vi "ui move files.vi"() -> ()   [LabVIEW 2023]
panel:
  out "Array 2":errorcluster[](array[cluster])
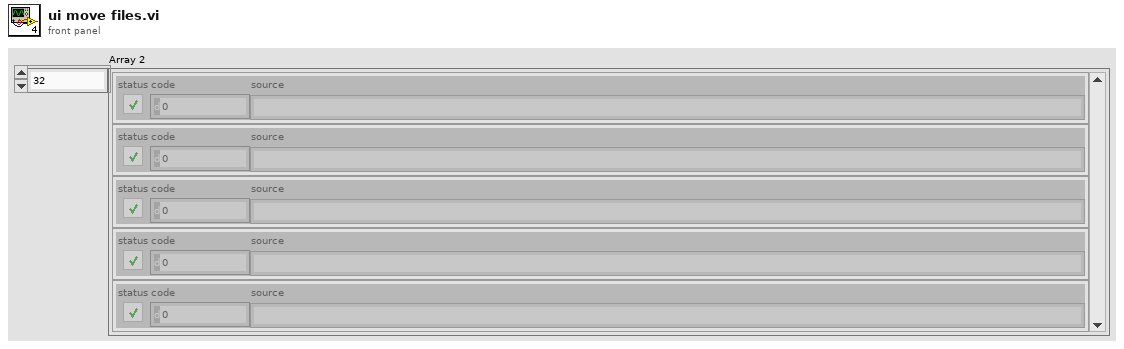
[diagram p1: front panel]
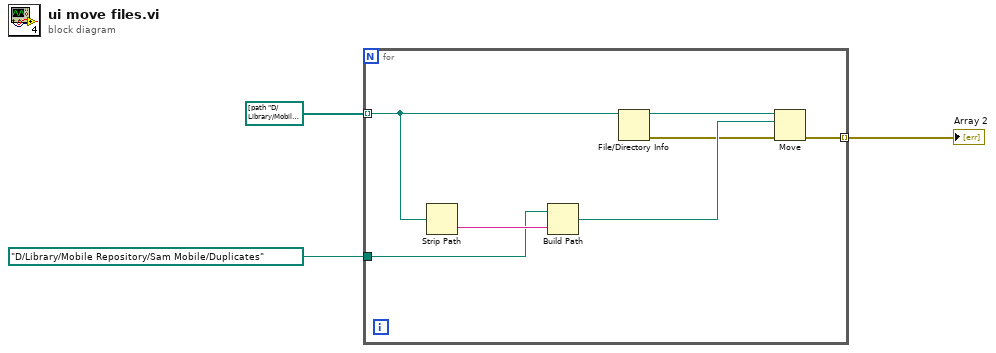
[diagram p0: block diagram]
diagram:
  n1 = for {
    tunnel: path[] [path "D:/Library/Mobile Repository/Sam Mobile/Albums/2017/08 August/iPhone 6s/20170810_162319 036_0000 iPhone 6s.JPG", path "D:/Library/Mobile Repository/Sam Mobile/Albums/2017/08 August/iPhone 6s/20170810_162319 121_0403 iPhone 6s.JPG", path "D:/Library/Mobile Repository/Sam Mobile/Albums/2017/08 August/iPhone 6s/20170814_132441 027_0000 iPhone 6s.JPG", path "D:/Library/Mobile Repository/Sam Mobile/Albums/2017/08 August/iPhone 6s/20170814_132441 121_0403 iPhone 6s.JPG", path "D:/Library/Mobile Repository/Sam Mobile/Albums/2017/08 August/iPhone 6s/20170814_134311 060_0000 iPhone 6s.JPG", path "D:/Library/Mobile Repository/Sam Mobile/Albums/2017/08 August/iPhone 6s/20170814_134311 121_0403 iPhone 6s.JPG", path "D:/Library/Mobile Repository/Sam Mobile/Albums/2017/08 August/iPhone 6s/20170816_123500 042_0000 iPhone 6s.JPG", path "D:/Library/Mobile Repository/Sam Mobile/Albums/2017/08 August/iPhone 6s/20170816_123500 121_0403 iPhone 6s.JPG", path "D:/Library/Mobile Repository/Sam Mobile/Albums/2017/08 August/iPhone 6s/20170822_182046 064_0000 iPhone 6s.JPG", path "D:/Library/Mobile Repository/Sam Mobile/Albums/2017/08 August/iPhone 6s/20170822_182046 121_0403 iPhone 6s.JPG", path "D:/Library/Mobile Repository/Sam Mobile/Albums/2017/08 August/iPhone 6s/20170823_115543 027_0000 iPhone 6s.JPG", path "D:/Library/Mobile Repository/Sam Mobile/Albums/2017/08 August/iPhone 6s/20170823_115543 121_0403 iPhone 6s.JPG", path "D:/Library/Mobile Repository/Sam Mobile/Albums/2017/08 August/iPhone 6s/20170823_115549 031_0000 iPhone 6s.JPG", path "D:/Library/Mobile Repository/Sam Mobile/Albums/2017/08 August/iPhone 6s/20170823_115549 121_0403 iPhone 6s.JPG", path "D:/Library/Mobile Repository/Sam Mobile/Albums/2017/08 August/iPhone 6s/20170825_201654 088_0000 iPhone 6s.JPG", path "D:/Library/Mobile Repository/Sam Mobile/Albums/2017/08 August/iPhone 6s/20170825_201654 121_0403 iPhone 6s.JPG", path "D:/Library/Mobile Repository/Sam Mobile/Albums/2017/08 August/iPhone 6s/20170825_204405 020_0000 iPhone 6s.JPG", path "D:/Library/Mobile Repository/Sam Mobile/Albums/2017/08 August/iPhone 6s/20170825_204405 121_0403 iPhone 6s.JPG", path "D:/Library/Mobile Repository/Sam Mobile/Albums/2017/09 September/iPhone 6s/20170907_130931 040_0000 iPhone 6s.JPG", path "D:/Library/Mobile Repository/Sam Mobile/Albums/2017/09 September/iPhone 6s/20170907_130931 121_0403 iPhone 6s.JPG", path "D:/Library/Mobile Repository/Sam Mobile/Albums/2017/09 September/iPhone 6s/20170907_223224 028_0000 iPhone 6s.JPG", path "D:/Library/Mobile Repository/Sam Mobile/Albums/2017/09 September/iPhone 6s/20170907_223224 121_0403 iPhone 6s.JPG", path "D:/Library/Mobile Repository/Sam Mobile/Albums/2017/09 September/iPhone 6s/20170923_163143 016_0000 iPhone 6s.JPG", path "D:/Library/Mobile Repository/Sam Mobile/Albums/2017/09 September/iPhone 6s/20170923_163143 121_0403 iPhone 6s.JPG", path "D:/Library/Mobile Repository/Sam Mobile/Albums/2017/10 October/iPhone 6s/20171013_075457 058_0000 iPhone 6s.JPG", path "D:/Library/Mobile Repository/Sam Mobile/Albums/2017/10 October/iPhone 6s/20171013_075457 121_0403 iPhone 6s.JPG", path "D:/Library/Mobile Repository/Sam Mobile/Albums/2017/10 October/iPhone 6s/20171030_155745 035_0000 iPhone 6s.JPG", path "D:/Library/Mobile Repository/Sam Mobile/Albums/2017/10 October/iPhone 6s/20171030_155745 121_0403 iPhone 6s.JPG", path "D:/Library/Mobile Repository/Sam Mobile/Albums/2017/12 December/iPhone 6s/20171204_111158 031_0000 iPhone 6s.JPG", path "D:/Library/Mobile Repository/Sam Mobile/Albums/2017/12 December/iPhone 6s/20171204_111158 121_0403 iPhone 6s.JPG", path "D:/Library/Mobile Repository/Sam Mobile/Albums/2017/12 December/iPhone 6s/20171209_180705 096_0000 iPhone 6s.JPG", path "D:/Library/Mobile Repository/Sam Mobile/Albums/2017/12 December/iPhone 6s/20171209_180705 121_0403 iPhone 6s.JPG", path "D:/Library/Mobile Repository/Sam Mobile/Albums/2017/12 December/iPhone 6s/20171221_164753 051_0000 iPhone 6s.JPG", path "D:/Library/Mobile Repository/Sam Mobile/Albums/2017/12 December/iPhone 6s/20171221_164753 121_0403 iPhone 6s.JPG", path "D:/Library/Mobile Repository/Sam Mobile/Albums/2018/02 February/iPhone 6s/20180203_103521 071_0000 iPhone 6s.JPG", path "D:/Library/Mobile Repository/Sam Mobile/Albums/2018/02 February/iPhone 6s/20180203_103521 121_0403 iPhone 6s.JPG", path "D:/Library/Mobile Repository/Sam Mobile/Albums/2018/02 February/iPhone 6s/20180212_064540 016_0000 iPhone 6s.JPG", path "D:/Library/Mobile Repository/Sam Mobile/Albums/2018/02 February/iPhone 6s/20180212_064540 121_0403 iPhone 6s.JPG", path "D:/Library/Mobile Repository/Sam Mobile/Albums/2018/02 February/iPhone 6s/20180224_102935 031_0000 iPhone 6s.JPG", path "D:/Library/Mobile Repository/Sam Mobile/Albums/2018/02 February/iPhone 6s/20180224_102935 121_0403 iPhone 6s.JPG", path "D:/Library/Mobile Repository/Sam Mobile/Albums/2018/02 February/iPhone 6s/20180224_152749 099_0000 iPhone 6s.JPG", path "D:/Library/Mobile Repository/Sam Mobile/Albums/2018/02 February/iPhone 6s/20180224_152749 121_0403 iPhone 6s.JPG", path "D:/Library/Mobile Repository/Sam Mobile/Albums/2018/03 March/iPhone 6s/20180315_064600 038_0000 iPhone 6s.JPG", path "D:/Library/Mobile Repository/Sam Mobile/Albums/2018/03 March/iPhone 6s/20180315_064600 121_0403 iPhone 6s.JPG", path "D:/Library/Mobile Repository/Sam Mobile/Albums/2018/03 March/iPhone 6s/20180318_193958 057_0000 iPhone 6s.JPG", path "D:/Library/Mobile Repository/Sam Mobile/Albums/2018/03 March/iPhone 6s/20180318_193958 121_0403 iPhone 6s.JPG", path "D:/Library/Mobile Repository/Sam Mobile/Albums/2018/04 April/iPhone 6s/20180426_163707 061_0000 iPhone 6s.JPG", path "D:/Library/Mobile Repository/Sam Mobile/Albums/2018/04 April/iPhone 6s/20180426_163707 121_0403 iPhone 6s.JPG", path "D:/Library/Mobile Repository/Sam Mobile/Albums/2018/05 May/iPhone 6s/20180513_133729 108_0000 iPhone 6s.JPG", path "D:/Library/Mobile Repository/Sam Mobile/Albums/2018/05 May/iPhone 6s/20180513_133729 121_0403 iPhone 6s.JPG", path "D:/Library/Mobile Repository/Sam Mobile/Albums/2018/05 May/iPhone 6s/20180518_112206 115_0000 iPhone 6s.JPG", path "D:/Library/Mobile Repository/Sam Mobile/Albums/2018/05 May/iPhone 6s/20180518_112206 121_0403 iPhone 6s.JPG", path "D:/Library/Mobile Repository/Sam Mobile/Albums/2018/05 May/iPhone 6s/20180521_132134 040_4745 iPhone 6s.JPG", path "D:/Library/Mobile Repository/Sam Mobile/Albums/2018/05 May/iPhone 6s/20180521_132134 121_0403 iPhone 6s.JPG", path "D:/Library/Mobile Repository/Sam Mobile/Albums/2018/06 June/iPhone 6s/20180629_113101 031_0000 iPhone 6s.JPG", path "D:/Library/Mobile Repository/Sam Mobile/Albums/2018/06 June/iPhone 6s/20180629_113101 121_0403 iPhone 6s.JPG", path "D:/Library/Mobile Repository/Sam Mobile/Albums/2018/06 June/iPhone 6s/20180629_113248 039_2914 iPhone 6s.JPG", path "D:/Library/Mobile Repository/Sam Mobile/Albums/2018/06 June/iPhone 6s/20180629_113248 121_0403 iPhone 6s.JPG", path "D:/Library/Mobile Repository/Sam Mobile/Albums/2018/07 July/iPhone 6s/20180719_113510 030_0000 iPhone 6s.JPG", path "D:/Library/Mobile Repository/Sam Mobile/Albums/2018/07 July/iPhone 6s/20180719_113510 121_0403 iPhone 6s.JPG", path "D:/Library/Mobile Repository/Sam Mobile/Albums/2018/07 July/iPhone 6s/20180720_182812 053_0000 iPhone 6s.JPG", path "D:/Library/Mobile Repository/Sam Mobile/Albums/2018/07 July/iPhone 6s/20180720_182812 121_0403 iPhone 6s.JPG", path "D:/Library/Mobile Repository/Sam Mobile/Albums/2018/07 July/iPhone 6s/20180723_190344 047_0000 iPhone 6s.JPG", path "D:/Library/Mobile Repository/Sam Mobile/Albums/2018/07 July/iPhone 6s/20180723_190344 121_0403 iPhone 6s.JPG", path "D:/Library/Mobile Repository/Sam Mobile/Albums/2018/07 July/iPhone 6s/20180730_211945 022_0000 iPhone 6s.JPG", path "D:/Library/Mobile Repository/Sam Mobile/Albums/2018/07 July/iPhone 6s/20180730_211945 121_0403 iPhone 6s.JPG", path "D:/Library/Mobile Repository/Sam Mobile/Albums/2018/08 August/iPhone 6s/20180811_092853 121_0304 iPhone 6s.JPG", path "D:/Library/Mobile Repository/Sam Mobile/Albums/2018/08 August/iPhone 6s/20180811_092853 121_0403 iPhone 6s.JPG", path "D:/Library/Mobile Repository/Sam Mobile/Albums/2018/08 August/iPhone 6s/20180812_113231 064_0000 iPhone 6s.JPG", path "D:/Library/Mobile Repository/Sam Mobile/Albums/2018/08 August/iPhone 6s/20180812_113231 121_0403 iPhone 6s.JPG", path "D:/Library/Mobile Repository/Sam Mobile/Albums/2018/09 September/iPhone 6s/20180901_123218 049_0304 iPhone 6s.JPG", path "D:/Library/Mobile Repository/Sam Mobile/Albums/2018/09 September/iPhone 6s/20180901_123218 049_0403 iPhone 6s.JPG", path "D:/Library/Mobile Repository/Sam Mobile/Albums/2018/10 October/iPhone 6s/20181008_175917 030_0000 iPhone 6s.JPG", path "D:/Library/Mobile Repository/Sam Mobile/Albums/2018/10 October/iPhone 6s/20181008_175917 121_0403 iPhone 6s.JPG", path "D:/Library/Mobile Repository/Sam Mobile/Albums/2018/12 December/iPhone 6s/20181210_155900 113_0000 iPhone 6s.JPG", path "D:/Library/Mobile Repository/Sam Mobile/Albums/2018/12 December/iPhone 6s/20181210_155900 121_0403 iPhone 6s.JPG", path "D:/Library/Mobile Repository/Sam Mobile/Albums/2019/01 January/iPhone 6s/20190106_113535 112_0000 iPhone 6s.JPG", path "D:/Library/Mobile Repository/Sam Mobile/Albums/2019/01 January/iPhone 6s/20190106_113535 121_0403 iPhone 6s.JPG", path "D:/Library/Mobile Repository/Sam Mobile/Albums/2019/01 January/iPhone 6s/20190112_084609 027_0000 iPhone 6s.JPG", path "D:/Library/Mobile Repository/Sam Mobile/Albums/2019/01 January/iPhone 6s/20190112_084609 121_0403 iPhone 6s.JPG", path "D:/Library/Mobile Repository/Sam Mobile/Albums/2019/01 January/iPhone 6s/20190112_084725 115_0000 iPhone 6s.JPG", path "D:/Library/Mobile Repository/Sam Mobile/Albums/2019/01 January/iPhone 6s/20190112_084725 121_0403 iPhone 6s.JPG", path "D:/Library/Mobile Repository/Sam Mobile/Albums/2019/01 January/iPhone 6s/20190126_103106 082_0000 iPhone 6s.JPG", path "D:/Library/Mobile Repository/Sam Mobile/Albums/2019/01 January/iPhone 6s/20190126_103106 121_0403 iPhone 6s.JPG", path "D:/Library/Mobile Repository/Sam Mobile/Albums/2019/02 February/iPhone 6s/20190219_194932 045_0000 iPhone 6s.JPG", path "D:/Library/Mobile Repository/Sam Mobile/Albums/2019/02 February/iPhone 6s/20190219_194932 121_0403 iPhone 6s.JPG", path "D:/Library/Mobile Repository/Sam Mobile/Albums/2019/03 March/iPhone 6s/20190315_211817 049_0000 iPhone 6s.JPG", path "D:/Library/Mobile Repository/Sam Mobile/Albums/2019/03 March/iPhone 6s/20190315_211817 121_0403 iPhone 6s.JPG", path "D:/Library/Mobile Repository/Sam Mobile/Albums/2019/03 March/iPhone 6s/20190319_212044 066_0000 iPhone 6s.JPG", path "D:/Library/Mobile Repository/Sam Mobile/Albums/2019/03 March/iPhone 6s/20190319_212044 121_0403 iPhone 6s.JPG", path "D:/Library/Mobile Repository/Sam Mobile/Albums/2019/04 April/iPhone 6s/20190410_091255 062_0000 iPhone 6s.JPG", path "D:/Library/Mobile Repository/Sam Mobile/Albums/2019/04 April/iPhone 6s/20190410_091255 121_0403 iPhone 6s.JPG", path "D:/Library/Mobile Repository/Sam Mobile/Albums/2019/04 April/iPhone 6s/20190410_091539 062_0000 iPhone 6s.JPG", path "D:/Library/Mobile Repository/Sam Mobile/Albums/2019/04 April/iPhone 6s/20190410_091539 121_0403 iPhone 6s.JPG", path "D:/Library/Mobile Repository/Sam Mobile/Albums/2019/04 April/iPhone 6s/20190410_094849 072_0000 iPhone 6s.JPG", path "D:/Library/Mobile Repository/Sam Mobile/Albums/2019/04 April/iPhone 6s/20190410_094849 121_0403 iPhone 6s.JPG", path "D:/Library/Mobile Repository/Sam Mobile/Albums/2019/04 April/iPhone 6s/20190420_141805 033_0000 iPhone 6s.JPG", path "D:/Library/Mobile Repository/Sam Mobile/Albums/2019/04 April/iPhone 6s/20190420_141805 121_0403 iPhone 6s.JPG", path "D:/Library/Mobile Repository/Sam Mobile/Albums/2019/05 May/iPhone 6s/20190516_180355 049_0000 iPhone 6s.JPG", path "D:/Library/Mobile Repository/Sam Mobile/Albums/2019/05 May/iPhone 6s/20190516_180355 121_0403 iPhone 6s.JPG", path "D:/Library/Mobile Repository/Sam Mobile/Albums/2019/05 May/iPhone 6s/20190519_175531 038_0000 iPhone 6s.JPG", path "D:/Library/Mobile Repository/Sam Mobile/Albums/2019/05 May/iPhone 6s/20190519_175531 121_0403 iPhone 6s.JPG", path "D:/Library/Mobile Repository/Sam Mobile/Albums/2019/05 May/iPhone 6s/20190523_190807 103_0000 iPhone 6s.JPG", path "D:/Library/Mobile Repository/Sam Mobile/Albums/2019/05 May/iPhone 6s/20190523_190807 121_0403 iPhone 6s.JPG", path "D:/Library/Mobile Repository/Sam Mobile/Albums/2019/06 June/iPhone 6s/20190608_173251 031_0000 iPhone 6s.JPG", path "D:/Library/Mobile Repository/Sam Mobile/Albums/2019/06 June/iPhone 6s/20190608_173251 121_0403 iPhone 6s.JPG", path "D:/Library/Mobile Repository/Sam Mobile/Albums/2019/06 June/iPhone 6s/20190608_215637 022_0000 iPhone 6s.JPG", path "D:/Library/Mobile Repository/Sam Mobile/Albums/2019/06 June/iPhone 6s/20190608_215637 121_0403 iPhone 6s.JPG", path "D:/Library/Mobile Repository/Sam Mobile/Albums/2019/07 July/iPhone 6s/20190706_160745 047_0000 iPhone 6s.JPG", path "D:/Library/Mobile Repository/Sam Mobile/Albums/2019/07 July/iPhone 6s/20190706_160745 121_0403 iPhone 6s.JPG", path "D:/Library/Mobile Repository/Sam Mobile/Albums/2019/07 July/iPhone 6s/20190721_093251 052_0000 iPhone 6s.JPG", path "D:/Library/Mobile Repository/Sam Mobile/Albums/2019/07 July/iPhone 6s/20190721_093251 121_0403 iPhone 6s.JPG", path "D:/Library/Mobile Repository/Sam Mobile/Albums/2019/08 August/iPhone 6s/20190810_091113 115_0000 iPhone 6s.JPG", path "D:/Library/Mobile Repository/Sam Mobile/Albums/2019/08 August/iPhone 6s/20190810_091113 121_0403 iPhone 6s.JPG", path "D:/Library/Mobile Repository/Sam Mobile/Albums/2019/08 August/iPhone 6s/20190817_105504 034_0000 iPhone 6s.JPG", path "D:/Library/Mobile Repository/Sam Mobile/Albums/2019/08 August/iPhone 6s/20190817_105504 121_0403 iPhone 6s.JPG", path "D:/Library/Mobile Repository/Sam Mobile/Albums/2019/09 September/iPhone 6s/20190907_143850 066_0000 iPhone 6s.JPG", path "D:/Library/Mobile Repository/Sam Mobile/Albums/2019/09 September/iPhone 6s/20190907_143850 121_0403 iPhone 6s.JPG", path "D:/Library/Mobile Repository/Sam Mobile/Albums/2019/09 September/iPhone 6s/20190910_001051 027_0000 iPhone 6s.JPG", path "D:/Library/Mobile Repository/Sam Mobile/Albums/2019/09 September/iPhone 6s/20190910_001051 121_0403 iPhone 6s.JPG", path "D:/Library/Mobile Repository/Sam Mobile/Albums/2019/09 September/iPhone 6s/20190918_162911 030_0000 iPhone 6s.JPG", path "D:/Library/Mobile Repository/Sam Mobile/Albums/2019/09 September/iPhone 6s/20190918_162911 121_0403 iPhone 6s.JPG", path "D:/Library/Mobile Repository/Sam Mobile/Albums/2019/10 October/iPhone 6s/20191006_111017 039_0000 iPhone 6s.JPG", path "D:/Library/Mobile Repository/Sam Mobile/Albums/2019/10 October/iPhone 6s/20191006_111017 121_0403 iPhone 6s.JPG", path "D:/Library/Mobile Repository/Sam Mobile/Albums/2019/10 October/iPhone 6s/20191010_103749 042_0000 iPhone 6s.JPG", path "D:/Library/Mobile Repository/Sam Mobile/Albums/2019/10 October/iPhone 6s/20191010_103749 121_0403 iPhone 6s.JPG", path "D:/Library/Mobile Repository/Sam Mobile/Albums/2019/10 October/iPhone 6s/20191023_130324 099_0000 iPhone 6s.JPG", path "D:/Library/Mobile Repository/Sam Mobile/Albums/2019/10 October/iPhone 6s/20191023_130324 121_0403 iPhone 6s.JPG", path "D:/Library/Mobile Repository/Sam Mobile/Albums/2019/11 November/iPhone 6s/20191102_142400 033_0000 iPhone 6s.JPG", path "D:/Library/Mobile Repository/Sam Mobile/Albums/2019/11 November/iPhone 6s/20191102_142400 121_0403 iPhone 6s.JPG", path "D:/Library/Mobile Repository/Sam Mobile/Albums/2019/11 November/iPhone 6s/20191111_204028 011_0000 iPhone 6s.JPG", path "D:/Library/Mobile Repository/Sam Mobile/Albums/2019/11 November/iPhone 6s/20191111_204028 121_0403 iPhone 6s.JPG", path "D:/Library/Mobile Repository/Sam Mobile/Albums/2019/11 November/iPhone 6s/20191111_204316 014_0000 iPhone 6s.JPG", path "D:/Library/Mobile Repository/Sam Mobile/Albums/2019/11 November/iPhone 6s/20191111_204316 121_0403 iPhone 6s.JPG", path "D:/Library/Mobile Repository/Sam Mobile/Albums/2019/11 November/iPhone 6s/20191123_203345 078_0000 iPhone 6s.JPG", path "D:/Library/Mobile Repository/Sam Mobile/Albums/2019/11 November/iPhone 6s/20191123_203345 121_0403 iPhone 6s.JPG", path "D:/Library/Mobile Repository/Sam Mobile/Albums/2019/12 December/iPhone 6s/20191204_222631 042_0000 iPhone 6s.JPG", path "D:/Library/Mobile Repository/Sam Mobile/Albums/2019/12 December/iPhone 6s/20191204_222631 121_0403 iPhone 6s.JPG", path "D:/Library/Mobile Repository/Sam Mobile/Albums/2019/12 December/iPhone 6s/20191224_094055 121_0304 iPhone 6s.JPG", path "D:/Library/Mobile Repository/Sam Mobile/Albums/2019/12 December/iPhone 6s/20191224_094055 121_0403 iPhone 6s.JPG", path "D:/Library/Mobile Repository/Sam Mobile/Albums/2020/01 January/iPhone 6s/20200125_103055 043_0000 iPhone 6s.JPG", path "D:/Library/Mobile Repository/Sam Mobile/Albums/2020/01 January/iPhone 6s/20200125_103055 121_0403 iPhone 6s.JPG", path "D:/Library/Mobile Repository/Sam Mobile/Albums/2020/02 February/iPhone 6s/20200202_192427 075_0000 iPhone 6s.JPG", path "D:/Library/Mobile Repository/Sam Mobile/Albums/2020/02 February/iPhone 6s/20200202_192427 121_0403 iPhone 6s.JPG", path "D:/Library/Mobile Repository/Sam Mobile/Albums/2020/03 March/iPhone 6s/20200310_135353 025_0000 iPhone 6s.JPG", path "D:/Library/Mobile Repository/Sam Mobile/Albums/2020/03 March/iPhone 6s/20200310_135353 121_0403 iPhone 6s.JPG", path "D:/Library/Mobile Repository/Sam Mobile/Albums/2020/03 March/iPhone 6s/20200324_082125 053_0000 iPhone 6s.JPG", path "D:/Library/Mobile Repository/Sam Mobile/Albums/2020/03 March/iPhone 6s/20200324_082125 121_0403 iPhone 6s.JPG", path "D:/Library/Mobile Repository/Sam Mobile/Albums/2020/03 March/iPhone 6s/20200324_082348 071_0000 iPhone 6s.JPG", path "D:/Library/Mobile Repository/Sam Mobile/Albums/2020/03 March/iPhone 6s/20200324_082348 121_0403 iPhone 6s.JPG", path "D:/Library/Mobile Repository/Sam Mobile/Albums/2020/04 April/iPhone 6s/20200404_214631 037_0000 iPhone 6s.JPG", path "D:/Library/Mobile Repository/Sam Mobile/Albums/2020/04 April/iPhone 6s/20200404_214631 121_0403 iPhone 6s.JPG", path "D:/Library/Mobile Repository/Sam Mobile/Albums/2020/04 April/iPhone 6s/20200426_205825 079_0000 iPhone 6s.JPG", path "D:/Library/Mobile Repository/Sam Mobile/Albums/2020/04 April/iPhone 6s/20200426_205825 121_0403 iPhone 6s.JPG", path "D:/Library/Mobile Repository/Sam Mobile/Albums/2020/07 July/iPhone 6s/20200727_124741 077_0000 iPhone 6s.JPG", path "D:/Library/Mobile Repository/Sam Mobile/Albums/2020/07 July/iPhone 6s/20200727_124741 121_0403 iPhone 6s.JPG", path "D:/Library/Mobile Repository/Sam Mobile/Albums/2020/08 August/iPhone 6s/20200825_221705 090_0000 iPhone 6s.JPG", path "D:/Library/Mobile Repository/Sam Mobile/Albums/2020/08 August/iPhone 6s/20200825_221705 121_0403 iPhone 6s.JPG", path "D:/Library/Mobile Repository/Sam Mobile/Albums/2020/09 September/iPhone 6s/20200920_113554 015_0000 iPhone 6s.JPG", path "D:/Library/Mobile Repository/Sam Mobile/Albums/2020/09 September/iPhone 6s/20200920_113554 121_0403 iPhone 6s.JPG", path "D:/Library/Mobile Repository/Sam Mobile/Albums/2020/10 October/iPhone 6s/20201002_174203 101_0000 iPhone 6s.JPG", path "D:/Library/Mobile Repository/Sam Mobile/Albums/2020/10 October/iPhone 6s/20201002_174203 121_0403 iPhone 6s.JPG", path "D:/Library/Mobile Repository/Sam Mobile/Albums/2020/10 October/iPhone 6s/20201017_131705 020_0000 iPhone 6s.JPG", path "D:/Library/Mobile Repository/Sam Mobile/Albums/2020/10 October/iPhone 6s/20201017_131705 121_0403 iPhone 6s.JPG", path "D:/Library/Mobile Repository/Sam Mobile/Albums/2020/10 October/iPhone 6s/20201020_091612 014_0000 iPhone 6s.JPG", path "D:/Library/Mobile Repository/Sam Mobile/Albums/2020/10 October/iPhone 6s/20201020_091612 121_0403 iPhone 6s.JPG", path "D:/Library/Mobile Repository/Sam Mobile/Albums/2020/11 November/iPhone 6s/20201102_093115 033_0000 iPhone 6s.JPG", path "D:/Library/Mobile Repository/Sam Mobile/Albums/2020/11 November/iPhone 6s/20201102_093115 121_0403 iPhone 6s.JPG", path "D:/Library/Mobile Repository/Sam Mobile/Albums/2020/11 November/iPhone 6s/20201103_142351 062_0000 iPhone 6s.JPG", path "D:/Library/Mobile Repository/Sam Mobile/Albums/2020/11 November/iPhone 6s/20201103_142351 121_0403 iPhone 6s.JPG", path "D:/Library/Mobile Repository/Sam Mobile/Albums/2020/11 November/iPhone 6s/20201106_190833 093_0000 iPhone 6s.JPG", path "D:/Library/Mobile Repository/Sam Mobile/Albums/2020/11 November/iPhone 6s/20201106_190833 121_0403 iPhone 6s.JPG", path "D:/Library/Mobile Repository/Sam Mobile/Albums/2021/01 January/iPhone SE/20210110_114045 035_0000 iPhone SE.JPG", path "D:/Library/Mobile Repository/Sam Mobile/Albums/2021/01 January/iPhone SE/20210110_114045 121_0403 iPhone SE.JPG", path "D:/Library/Mobile Repository/Sam Mobile/Albums/2021/01 January/iPhone SE/20210124_173927 026_0000 iPhone SE.JPG", path "D:/Library/Mobile Repository/Sam Mobile/Albums/2021/01 January/iPhone SE/20210124_173927 121_0403 iPhone SE.JPG", path "D:/Library/Mobile Repository/Sam Mobile/Albums/2021/03 March/iPhone SE/20210306_155858 087_0000 iPhone SE.JPG", path "D:/Library/Mobile Repository/Sam Mobile/Albums/2021/03 March/iPhone SE/20210306_155858 121_0403 iPhone SE.JPG", path "D:/Library/Mobile Repository/Sam Mobile/Albums/2021/03 March/iPhone SE/20210312_181408 088_0000 iPhone SE.JPG", path "D:/Library/Mobile Repository/Sam Mobile/Albums/2021/03 March/iPhone SE/20210312_181408 121_0403 iPhone SE.JPG", path "D:/Library/Mobile Repository/Sam Mobile/Albums/2021/04 April/iPhone SE/20210403_194008 028_0000 iPhone SE.JPG", path "D:/Library/Mobile Repository/Sam Mobile/Albums/2021/04 April/iPhone SE/20210403_194008 121_0403 iPhone SE.JPG", path "D:/Library/Mobile Repository/Sam Mobile/Albums/2021/05 May/iPhone SE/20210529_163718 020_0000 iPhone SE.JPG", path "D:/Library/Mobile Repository/Sam Mobile/Albums/2021/05 May/iPhone SE/20210529_163718 121_0403 iPhone SE.JPG", path "D:/Library/Mobile Repository/Sam Mobile/Albums/2021/06 June/iPhone SE/20210603_194256 082_1609 iPhone SE.JPG", path "D:/Library/Mobile Repository/Sam Mobile/Albums/2021/06 June/iPhone SE/20210603_194256 121_0403 iPhone SE.JPG", path "D:/Library/Mobile Repository/Sam Mobile/Albums/2021/07 July/iPhone SE/20210707_110414 039_0000 iPhone SE.JPG", path "D:/Library/Mobile Repository/Sam Mobile/Albums/2021/07 July/iPhone SE/20210707_110414 121_0403 iPhone SE.JPG", path "D:/Library/Mobile Repository/Sam Mobile/Albums/2021/07 July/iPhone SE/20210711_120127 078_0000 iPhone SE.JPG", path "D:/Library/Mobile Repository/Sam Mobile/Albums/2021/07 July/iPhone SE/20210711_120127 121_0403 iPhone SE.JPG", path "D:/Library/Mobile Repository/Sam Mobile/Albums/2021/07 July/iPhone SE/20210711_120302 088_0000 iPhone SE.JPG", path "D:/Library/Mobile Repository/Sam Mobile/Albums/2021/07 July/iPhone SE/20210711_120302 121_0403 iPhone SE.JPG", path "D:/Library/Mobile Repository/Sam Mobile/Albums/2021/07 July/iPhone SE/20210722_185415 092_0000 iPhone SE.JPG", path "D:/Library/Mobile Repository/Sam Mobile/Albums/2021/07 July/iPhone SE/20210722_185415 121_0403 iPhone SE.JPG", path "D:/Library/Mobile Repository/Sam Mobile/Albums/2021/08 August/iPhone SE/20210806_192444 077_0000 iPhone SE.JPG", path "D:/Library/Mobile Repository/Sam Mobile/Albums/2021/08 August/iPhone SE/20210806_192444 121_0403 iPhone SE.JPG", path "D:/Library/Mobile Repository/Sam Mobile/Albums/2022/03 March/iPhone SE/20220324_102052 082_1609 iPhone SE.JPG", path "D:/Library/Mobile Repository/Sam Mobile/Albums/2022/03 March/iPhone SE/20220324_102052 110_0403 iPhone SE.JPG", path "D:/Library/Mobile Repository/Sam Mobile/Albums/2022/03 March/iPhone SE/20220324_114316 082_1609 iPhone SE.JPG", path "D:/Library/Mobile Repository/Sam Mobile/Albums/2022/03 March/iPhone SE/20220324_114316 110_0403 iPhone SE.JPG", path "D:/Library/Mobile Repository/Sam Mobile/Albums/2022/03 March/iPhone SE/20220324_114806 110_0304 iPhone SE.JPG", path "D:/Library/Mobile Repository/Sam Mobile/Albums/2022/03 March/iPhone SE/20220324_114806 121_0304 iPhone SE.JPG", path "D:/Library/Mobile Repository/Sam Mobile/Albums/2022/03 March/iPhone SE/20220324_114833 110_0304 iPhone SE.JPG", path "D:/Library/Mobile Repository/Sam Mobile/Albums/2022/03 March/iPhone SE/20220324_114833 121_0304 iPhone SE.JPG", path "D:/Library/Mobile Repository/Sam Mobile/Albums/2022/03 March/iPhone SE/20220324_133518 082_1609 iPhone SE.JPG", path "D:/Library/Mobile Repository/Sam Mobile/Albums/2022/03 March/iPhone SE/20220324_133518 110_0403 iPhone SE.JPG", path "D:/Library/Mobile Repository/Sam Mobile/Albums/2022/03 March/iPhone SE/20220324_133531 082_1609 iPhone SE.JPG", path "D:/Library/Mobile Repository/Sam Mobile/Albums/2022/03 March/iPhone SE/20220324_133531 110_0403 iPhone SE.JPG", path "D:/Library/Mobile Repository/Sam Mobile/Albums/2022/03 March/iPhone SE/20220324_134958 082_1609 iPhone SE.JPG", path "D:/Library/Mobile Repository/Sam Mobile/Albums/2022/03 March/iPhone SE/20220324_134958 110_0403 iPhone SE.JPG", path "D:/Library/Mobile Repository/Sam Mobile/Albums/2022/03 March/iPhone SE/20220331_112844 082_1609 iPhone SE.JPG", path "D:/Library/Mobile Repository/Sam Mobile/Albums/2022/03 March/iPhone SE/20220331_112844 110_0403 iPhone SE.JPG", path "D:/Library/Mobile Repository/Sam Mobile/Albums/2022/03 March/iPhone SE/20220331_112925 082_1609 iPhone SE.JPG", path "D:/Library/Mobile Repository/Sam Mobile/Albums/2022/03 March/iPhone SE/20220331_112925 110_0403 iPhone SE.JPG", path "D:/Library/Mobile Repository/Sam Mobile/Albums/2022/03 March/iPhone SE/20220331_113028 082_1609 iPhone SE.JPG", path "D:/Library/Mobile Repository/Sam Mobile/Albums/2022/03 March/iPhone SE/20220331_113028 110_0403 iPhone SE.JPG", path "D:/Library/Mobile Repository/Sam Mobile/Albums/2022/06 June/iPhone 12/20220623_185013 082_1609 iPhone 12.JPG", path "D:/Library/Mobile Repository/Sam Mobile/Albums/2022/06 June/iPhone 12/20220623_185013 121_0403 iPhone 12.JPG", path "D:/Library/Mobile Repository/Sam Mobile/Albums/2022/06 June/iPhone 12/20220629_190101 023_0000 iPhone 12.JPG", path "D:/Library/Mobile Repository/Sam Mobile/Albums/2022/06 June/iPhone 12/20220629_190101 121_0403 iPhone 12.JPG", path "D:/Library/Mobile Repository/Sam Mobile/Albums/2022/06 June/iPhone 12/20220629_191223 110_0403 iPhone 12.JPG", path "D:/Library/Mobile Repository/Sam Mobile/Albums/2022/06 June/iPhone 12/20220629_191223 121_0403 iPhone 12.JPG", path "D:/Library/Mobile Repository/Sam Mobile/Albums/2022/06 June/iPhone 12/20220629_191719 110_0403 iPhone 12.JPG", path "D:/Library/Mobile Repository/Sam Mobile/Albums/2022/06 June/iPhone 12/20220629_191719 121_0403 iPhone 12.JPG", path "D:/Library/Mobile Repository/Sam Mobile/Albums/2022/06 June/iPhone 12/20220630_130151 110_0403 iPhone 12.JPG", path "D:/Library/Mobile Repository/Sam Mobile/Albums/2022/06 June/iPhone 12/20220630_130151 121_0403 iPhone 12.JPG", path "D:/Library/Mobile Repository/Sam Mobile/Albums/2022/07 July/iPhone 12/20220701_130456 029_0000 iPhone 12.JPG", path "D:/Library/Mobile Repository/Sam Mobile/Albums/2022/07 July/iPhone 12/20220701_130456 121_0403 iPhone 12.JPG", path "D:/Library/Mobile Repository/Sam Mobile/Albums/2022/07 July/iPhone 12/20220701_165602 006_0000 iPhone 12.JPG", path "D:/Library/Mobile Repository/Sam Mobile/Albums/2022/07 July/iPhone 12/20220701_165602 121_0403 iPhone 12.JPG", path "D:/Library/Mobile Repository/Sam Mobile/Albums/2022/07 July/iPhone 12/20220702_150102 110_0403 iPhone 12.JPG", path "D:/Library/Mobile Repository/Sam Mobile/Albums/2022/07 July/iPhone 12/20220702_150102 121_0403 iPhone 12.JPG", path "D:/Library/Mobile Repository/Sam Mobile/Albums/2022/07 July/iPhone 12/20220709_085812 082_1609 iPhone 12.JPG", path "D:/Library/Mobile Repository/Sam Mobile/Albums/2022/07 July/iPhone 12/20220709_085812 091_1609 iPhone 12.JPG", path "D:/Library/Mobile Repository/Sam Mobile/Albums/2022/07 July/iPhone 12/20220709_085812 121_0403 iPhone 12.JPG", path "D:/Library/Mobile Repository/Sam Mobile/Albums/2022/07 July/iPhone 12/20220710_124915 082_1609 iPhone 12.JPG", path "D:/Library/Mobile Repository/Sam Mobile/Albums/2022/07 July/iPhone 12/20220710_124915 091_1609 iPhone 12.JPG", path "D:/Library/Mobile Repository/Sam Mobile/Albums/2022/07 July/iPhone 12/20220710_124915 121_0403 iPhone 12.JPG", path "D:/Library/Mobile Repository/Sam Mobile/Albums/2022/07 July/iPhone 12/20220711_131706 091_1609 iPhone 12.JPG", path "D:/Library/Mobile Repository/Sam Mobile/Albums/2022/07 July/iPhone 12/20220711_131706 121_0403 iPhone 12.JPG", path "D:/Library/Mobile Repository/Sam Mobile/Albums/2022/07 July/iPhone 12/20220711_131711 082_1609 iPhone 12.JPG", path "D:/Library/Mobile Repository/Sam Mobile/Albums/2022/07 July/iPhone 12/20220711_131711 091_1609 iPhone 12.JPG", path "D:/Library/Mobile Repository/Sam Mobile/Albums/2022/07 July/iPhone 12/20220711_131711 121_0403 iPhone 12.JPG", path "D:/Library/Mobile Repository/Sam Mobile/Albums/2022/07 July/iPhone 12/20220711_131740 082_1609 iPhone 12.JPG", path "D:/Library/Mobile Repository/Sam Mobile/Albums/2022/07 July/iPhone 12/20220711_131740 091_1609 iPhone 12.JPG", path "D:/Library/Mobile Repository/Sam Mobile/Albums/2022/07 July/iPhone 12/20220711_131740 121_0403 iPhone 12.JPG", path "D:/Library/Mobile Repository/Sam Mobile/Albums/2022/07 July/iPhone 12/20220712_094432 082_1609 iPhone 12.JPG", path "D:/Library/Mobile Repository/Sam Mobile/Albums/2022/07 July/iPhone 12/20220712_094432 121_0403 iPhone 12.JPG", path "D:/Library/Mobile Repository/Sam Mobile/Albums/2022/07 July/iPhone 12/20220713_140852 082_1609 iPhone 12.JPG", path "D:/Library/Mobile Repository/Sam Mobile/Albums/2022/07 July/iPhone 12/20220713_140852 091_1609 iPhone 12.JPG", path "D:/Library/Mobile Repository/Sam Mobile/Albums/2022/07 July/iPhone 12/20220713_140852 121_0403 iPhone 12.JPG", path "D:/Library/Mobile Repository/Sam Mobile/Albums/2022/07 July/iPhone 12/20220714_100950 082_1609 iPhone 12.JPG", path "D:/Library/Mobile Repository/Sam Mobile/Albums/2022/07 July/iPhone 12/20220714_100950 091_1609 iPhone 12.JPG", path "D:/Library/Mobile Repository/Sam Mobile/Albums/2022/07 July/iPhone 12/20220714_100950 121_0403 iPhone 12.JPG", path "D:/Library/Mobile Repository/Sam Mobile/Albums/2022/07 July/iPhone 12/20220714_103534 082_1609 iPhone 12.JPG", path "D:/Library/Mobile Repository/Sam Mobile/Albums/2022/07 July/iPhone 12/20220714_103534 091_1609 iPhone 12.JPG", path "D:/Library/Mobile Repository/Sam Mobile/Albums/2022/07 July/iPhone 12/20220714_103534 121_0403 iPhone 12.JPG", path "D:/Library/Mobile Repository/Sam Mobile/Albums/2022/07 July/iPhone 12/20220714_103755 082_1609 iPhone 12.JPG", path "D:/Library/Mobile Repository/Sam Mobile/Albums/2022/07 July/iPhone 12/20220714_103755 091_1609 iPhone 12.JPG", path "D:/Library/Mobile Repository/Sam Mobile/Albums/2022/07 July/iPhone 12/20220714_103755 121_0403 iPhone 12.JPG", path "D:/Library/Mobile Repository/Sam Mobile/Albums/2022/07 July/iPhone 12/20220715_182135 082_1609 iPhone 12.JPG", path "D:/Library/Mobile Repository/Sam Mobile/Albums/2022/07 July/iPhone 12/20220715_182135 091_1609 iPhone 12.JPG", path "D:/Library/Mobile Repository/Sam Mobile/Albums/2022/07 July/iPhone 12/20220715_182135 121_0403 iPhone 12.JPG", path "D:/Library/Mobile Repository/Sam Mobile/Albums/2022/07 July/iPhone 12/20220715_182948 082_1609 iPhone 12.JPG", path "D:/Library/Mobile Repository/Sam Mobile/Albums/2022/07 July/iPhone 12/20220715_182948 091_1609 iPhone 12.JPG", path "D:/Library/Mobile Repository/Sam Mobile/Albums/2022/07 July/iPhone 12/20220715_182948 121_0403 iPhone 12.JPG", path "D:/Library/Mobile Repository/Sam Mobile/Albums/2022/07 July/iPhone 12/20220715_183238 082_1609 iPhone 12.JPG", path "D:/Library/Mobile Repository/Sam Mobile/Albums/2022/07 July/iPhone 12/20220715_183238 091_1609 iPhone 12.JPG", path "D:/Library/Mobile Repository/Sam Mobile/Albums/2022/07 July/iPhone 12/20220715_183238 121_0403 iPhone 12.JPG", path "D:/Library/Mobile Repository/Sam Mobile/Albums/2022/07 July/iPhone 12/20220715_183325 082_1609 iPhone 12.JPG", path "D:/Library/Mobile Repository/Sam Mobile/Albums/2022/07 July/iPhone 12/20220715_183325 091_1609 iPhone 12.JPG", path "D:/Library/Mobile Repository/Sam Mobile/Albums/2022/07 July/iPhone 12/20220715_183325 121_0403 iPhone 12.JPG", path "D:/Library/Mobile Repository/Sam Mobile/Albums/2022/07 July/iPhone 12/20220723_161536 028_0000 iPhone 12.JPG", path "D:/Library/Mobile Repository/Sam Mobile/Albums/2022/07 July/iPhone 12/20220723_161536 121_0403 iPhone 12.JPG", path "D:/Library/Mobile Repository/Sam Mobile/Albums/2022/07 July/iPhone 12/20220730_194549 091_0916 iPhone 12.JPG", path "D:/Library/Mobile Repository/Sam Mobile/Albums/2022/07 July/iPhone 12/20220730_194549 121_0403 iPhone 12.JPG", path "D:/Library/Mobile Repository/Sam Mobile/Albums/2022/07 July/iPhone 12/20220730_212000 082_1609 iPhone 12.JPG", path "D:/Library/Mobile Repository/Sam Mobile/Albums/2022/07 July/iPhone 12/20220730_212000 091_1609 iPhone 12.JPG", path "D:/Library/Mobile Repository/Sam Mobile/Albums/2022/07 July/iPhone 12/20220730_212000 121_0403 iPhone 12.JPG", path "D:/Library/Mobile Repository/Sam Mobile/Albums/2022/07 July/iPhone 12/20220730_215327 082_1609 iPhone 12.JPG", path "D:/Library/Mobile Repository/Sam Mobile/Albums/2022/07 July/iPhone 12/20220730_215327 091_1609 iPhone 12.JPG", path "D:/Library/Mobile Repository/Sam Mobile/Albums/2022/07 July/iPhone 12/20220730_215327 121_0403 iPhone 12.JPG", path "D:/Library/Mobile Repository/Sam Mobile/Albums/2022/07 July/iPhone 12/20220730_215725 082_1609 iPhone 12.JPG", path "D:/Library/Mobile Repository/Sam Mobile/Albums/2022/07 July/iPhone 12/20220730_215725 121_0403 iPhone 12.JPG", path "D:/Library/Mobile Repository/Sam Mobile/Albums/2022/07 July/iPhone 12/20220730_215757 082_1609 iPhone 12.JPG", path "D:/Library/Mobile Repository/Sam Mobile/Albums/2022/07 July/iPhone 12/20220730_215757 121_0403 iPhone 12.JPG", path "D:/Library/Mobile Repository/Sam Mobile/Albums/2022/07 July/iPhone 12/20220730_221630 082_1609 iPhone 12.JPG", path "D:/Library/Mobile Repository/Sam Mobile/Albums/2022/07 July/iPhone 12/20220730_221630 091_1609 iPhone 12.JPG", path "D:/Library/Mobile Repository/Sam Mobile/Albums/2022/07 July/iPhone 12/20220730_221630 121_0403 iPhone 12.JPG", path "D:/Library/Mobile Repository/Sam Mobile/Albums/2022/07 July/iPhone 12/20220730_221720 082_1609 iPhone 12.JPG", path "D:/Library/Mobile Repository/Sam Mobile/Albums/2022/07 July/iPhone 12/20220730_221720 091_1609 iPhone 12.JPG", path "D:/Library/Mobile Repository/Sam Mobile/Albums/2022/07 July/iPhone 12/20220730_221720 121_0403 iPhone 12.JPG", path "D:/Library/Mobile Repository/Sam Mobile/Albums/2022/07 July/iPhone 12/20220730_221734 082_1609 iPhone 12.JPG", path "D:/Library/Mobile Repository/Sam Mobile/Albums/2022/07 July/iPhone 12/20220730_221734 091_1609 iPhone 12.JPG", path "D:/Library/Mobile Repository/Sam Mobile/Albums/2022/07 July/iPhone 12/20220730_221734 121_0403 iPhone 12.JPG", path "D:/Library/Mobile Repository/Sam Mobile/Albums/2022/08 August/iPhone 12/20220801_114551 082_1609 iPhone 12.JPG", path "D:/Library/Mobile Repository/Sam Mobile/Albums/2022/08 August/iPhone 12/20220801_114551 091_1609 iPhone 12.JPG", path "D:/Library/Mobile Repository/Sam Mobile/Albums/2022/08 August/iPhone 12/20220801_114551 121_0403 iPhone 12.JPG", path "D:/Library/Mobile Repository/Sam Mobile/Albums/2022/08 August/iPhone 12/20220802_174320 082_1609 iPhone 12.JPG", path "D:/Library/Mobile Repository/Sam Mobile/Albums/2022/08 August/iPhone 12/20220802_174320 091_1609 iPhone 12.JPG", path "D:/Library/Mobile Repository/Sam Mobile/Albums/2022/08 August/iPhone 12/20220802_174320 121_0403 iPhone 12.JPG", path "D:/Library/Mobile Repository/Sam Mobile/Albums/2022/08 August/iPhone 12/20220803_152050 082_1609 iPhone 12.JPG", path "D:/Library/Mobile Repository/Sam Mobile/Albums/2022/08 August/iPhone 12/20220803_152050 091_1609 iPhone 12.JPG", path "D:/Library/Mobile Repository/Sam Mobile/Albums/2022/08 August/iPhone 12/20220803_152050 121_0403 iPhone 12.JPG", path "D:/Library/Mobile Repository/Sam Mobile/Albums/2022/08 August/iPhone 12/20220803_175329 082_1609 iPhone 12.JPG", path "D:/Library/Mobile Repository/Sam Mobile/Albums/2022/08 August/iPhone 12/20220803_175329 091_1609 iPhone 12.JPG", path "D:/Library/Mobile Repository/Sam Mobile/Albums/2022/08 August/iPhone 12/20220803_175329 121_0403 iPhone 12.JPG", path "D:/Library/Mobile Repository/Sam Mobile/Albums/2022/08 August/iPhone 12/20220803_175414 082_1609 iPhone 12.JPG", path "D:/Library/Mobile Repository/Sam Mobile/Albums/2022/08 August/iPhone 12/20220803_175414 091_1609 iPhone 12.JPG", path "D:/Library/Mobile Repository/Sam Mobile/Albums/2022/08 August/iPhone 12/20220803_175414 121_0403 iPhone 12.JPG", path "D:/Library/Mobile Repository/Sam Mobile/Albums/2022/08 August/iPhone 12/20220805_212914 082_1609 iPhone 12.JPG", path "D:/Library/Mobile Repository/Sam Mobile/Albums/2022/08 August/iPhone 12/20220805_212914 121_0403 iPhone 12.JPG", path "D:/Library/Mobile Repository/Sam Mobile/Albums/2022/08 August/iPhone 12/20220806_150052 074_0000 iPhone 12.JPG", path "D:/Library/Mobile Repository/Sam Mobile/Albums/2022/08 August/iPhone 12/20220806_150052 121_0403 iPhone 12.JPG", path "D:/Library/Mobile Repository/Sam Mobile/Albums/2022/08 August/iPhone 12/20220806_204659 082_1609 iPhone 12.JPG", path "D:/Library/Mobile Repository/Sam Mobile/Albums/2022/08 August/iPhone 12/20220806_204659 091_1609 iPhone 12.JPG", path "D:/Library/Mobile Repository/Sam Mobile/Albums/2022/08 August/iPhone 12/20220806_204659 121_0403 iPhone 12.JPG", path "D:/Library/Mobile Repository/Sam Mobile/Albums/2022/08 August/iPhone 12/20220806_204704 082_1609 iPhone 12.JPG", path "D:/Library/Mobile Repository/Sam Mobile/Albums/2022/08 August/iPhone 12/20220806_204704 091_1609 iPhone 12.JPG", path "D:/Library/Mobile Repository/Sam Mobile/Albums/2022/08 August/iPhone 12/20220806_204704 121_0403 iPhone 12.JPG", path "D:/Library/Mobile Repository/Sam Mobile/Albums/2022/08 August/iPhone 12/20220806_204801 082_1609 iPhone 12.JPG", path "D:/Library/Mobile Repository/Sam Mobile/Albums/2022/08 August/iPhone 12/20220806_204801 091_1609 iPhone 12.JPG", path "D:/Library/Mobile Repository/Sam Mobile/Albums/2022/08 August/iPhone 12/20220806_204801 121_0403 iPhone 12.JPG", path "D:/Library/Mobile Repository/Sam Mobile/Albums/2022/08 August/iPhone 12/20220806_204805 091_0916 iPhone 12.JPG", path "D:/Library/Mobile Repository/Sam Mobile/Albums/2022/08 August/iPhone 12/20220806_204805 121_0403 iPhone 12.JPG", path "D:/Library/Mobile Repository/Sam Mobile/Albums/2022/08 August/iPhone 12/20220806_204810 091_0916 iPhone 12.JPG", path "D:/Library/Mobile Repository/Sam Mobile/Albums/2022/08 August/iPhone 12/20220806_204810 110_0403 iPhone 12.JPG", path "D:/Library/Mobile Repository/Sam Mobile/Albums/2022/08 August/iPhone 12/20220806_204810 121_0403 iPhone 12.JPG", path "D:/Library/Mobile Repository/Sam Mobile/Albums/2022/08 August/iPhone 12/20220806_204812 091_0916 iPhone 12.JPG", path "D:/Library/Mobile Repository/Sam Mobile/Albums/2022/08 August/iPhone 12/20220806_204812 110_0403 iPhone 12.JPG", path "D:/Library/Mobile Repository/Sam Mobile/Albums/2022/08 August/iPhone 12/20220806_204812 121_0403 iPhone 12.JPG", path "D:/Library/Mobile Repository/Sam Mobile/Albums/2022/08 August/iPhone 12/20220807_180146 089_0000 iPhone 12.JPG", path "D:/Library/Mobile Repository/Sam Mobile/Albums/2022/08 August/iPhone 12/20220807_180146 121_0403 iPhone 12.JPG", path "D:/Library/Mobile Repository/Sam Mobile/Albums/2022/08 August/iPhone 12/20220807_181044 121_0304 iPhone 12.JPG", path "D:/Library/Mobile Repository/Sam Mobile/Albums/2022/08 August/iPhone 12/20220807_181044 121_0403 iPhone 12.JPG", path "D:/Library/Mobile Repository/Sam Mobile/Albums/2022/08 August/iPhone 12/20220809_124037 082_1609 iPhone 12.JPG", path "D:/Library/Mobile Repository/Sam Mobile/Albums/2022/08 August/iPhone 12/20220809_124037 091_1609 iPhone 12.JPG", path "D:/Library/Mobile Repository/Sam Mobile/Albums/2022/08 August/iPhone 12/20220809_124037 121_0403 iPhone 12.JPG", path "D:/Library/Mobile Repository/Sam Mobile/Albums/2022/08 August/iPhone 12/20220809_124503 082_1609 iPhone 12.JPG", path "D:/Library/Mobile Repository/Sam Mobile/Albums/2022/08 August/iPhone 12/20220809_124503 091_1609 iPhone 12.JPG", path "D:/Library/Mobile Repository/Sam Mobile/Albums/2022/08 August/iPhone 12/20220809_124503 121_0403 iPhone 12.JPG", path "D:/Library/Mobile Repository/Sam Mobile/Albums/2022/08 August/iPhone 12/20220810_120340 022_0000 iPhone 12.JPG", path "D:/Library/Mobile Repository/Sam Mobile/Albums/2022/08 August/iPhone 12/20220810_120340 110_0403 iPhone 12.JPG", path "D:/Library/Mobile Repository/Sam Mobile/Albums/2022/08 August/iPhone 12/20220810_120340 121_0403 iPhone 12.JPG", path "D:/Library/Mobile Repository/Sam Mobile/Albums/2022/08 August/iPhone 12/20220811_203614 110_0403 iPhone 12.JPG", path "D:/Library/Mobile Repository/Sam Mobile/Albums/2022/08 August/iPhone 12/20220811_203614 121_0403 iPhone 12.JPG", path "D:/Library/Mobile Repository/Sam Mobile/Albums/2022/08 August/iPhone 12/20220811_223750 082_0916 iPhone 12.JPG", path "D:/Library/Mobile Repository/Sam Mobile/Albums/2022/08 August/iPhone 12/20220811_223750 082_1609 iPhone 12.JPG", path "D:/Library/Mobile Repository/Sam Mobile/Albums/2022/08 August/iPhone 12/20220812_173711 082_1609 iPhone 12.JPG", path "D:/Library/Mobile Repository/Sam Mobile/Albums/2022/08 August/iPhone 12/20220812_173711 121_0403 iPhone 12.JPG", path "D:/Library/Mobile Repository/Sam Mobile/Albums/2022/08 August/iPhone 12/20220812_192048 082_1609 iPhone 12.JPG", path "D:/Library/Mobile Repository/Sam Mobile/Albums/2022/08 August/iPhone 12/20220812_192048 091_0000 iPhone 12.JPG", path "D:/Library/Mobile Repository/Sam Mobile/Albums/2022/08 August/iPhone 12/20220812_192048 121_0403 iPhone 12.JPG", path "D:/Library/Mobile Repository/Sam Mobile/Albums/2022/08 August/iPhone 12/20220812_192052 082_1609 iPhone 12.JPG", path "D:/Library/Mobile Repository/Sam Mobile/Albums/2022/08 August/iPhone 12/20220812_192052 091_0000 iPhone 12.JPG", path "D:/Library/Mobile Repository/Sam Mobile/Albums/2022/08 August/iPhone 12/20220812_192052 121_0403 iPhone 12.JPG", path "D:/Library/Mobile Repository/Sam Mobile/Albums/2022/08 August/iPhone 12/20220812_192255 082_1609 iPhone 12.JPG", path "D:/Library/Mobile Repository/Sam Mobile/Albums/2022/08 August/iPhone 12/20220812_192255 091_0000 iPhone 12.JPG", path "D:/Library/Mobile Repository/Sam Mobile/Albums/2022/08 August/iPhone 12/20220812_192255 121_0403 iPhone 12.JPG", path "D:/Library/Mobile Repository/Sam Mobile/Albums/2022/08 August/iPhone 12/20220812_192340 082_1609 iPhone 12.JPG", path "D:/Library/Mobile Repository/Sam Mobile/Albums/2022/08 August/iPhone 12/20220812_192340 091_1609 iPhone 12.JPG", path "D:/Library/Mobile Repository/Sam Mobile/Albums/2022/08 August/iPhone 12/20220812_192340 121_0403 iPhone 12.JPG", path "D:/Library/Mobile Repository/Sam Mobile/Albums/2022/08 August/iPhone 12/20220812_192359 082_1609 iPhone 12.JPG", path "D:/Library/Mobile Repository/Sam Mobile/Albums/2022/08 August/iPhone 12/20220812_192359 091_1609 iPhone 12.JPG", path "D:/Library/Mobile Repository/Sam Mobile/Albums/2022/08 August/iPhone 12/20220812_192359 121_0403 iPhone 12.JPG", path "D:/Library/Mobile Repository/Sam Mobile/Albums/2022/08 August/iPhone 12/20220813_180510 067_0000 iPhone 12.JPG", path "D:/Library/Mobile Repository/Sam Mobile/Albums/2022/08 August/iPhone 12/20220813_180510 121_0403 iPhone 12.JPG", path "D:/Library/Mobile Repository/Sam Mobile/Albums/2022/08 August/iPhone 12/20220813_181140 074_0000 iPhone 12.JPG", path "D:/Library/Mobile Repository/Sam Mobile/Albums/2022/08 August/iPhone 12/20220813_181140 121_0403 iPhone 12.JPG", path "D:/Library/Mobile Repository/Sam Mobile/Albums/2022/08 August/iPhone 12/20220815_143916 082_1609 iPhone 12.JPG", path "D:/Library/Mobile Repository/Sam Mobile/Albums/2022/08 August/iPhone 12/20220815_143916 091_1609 iPhone 12.JPG", path "D:/Library/Mobile Repository/Sam Mobile/Albums/2022/08 August/iPhone 12/20220815_143916 121_0403 iPhone 12.JPG", path "D:/Library/Mobile Repository/Sam Mobile/Albums/2022/08 August/iPhone 12/20220818_130608 082_1609 iPhone 12.JPG", path "D:/Library/Mobile Repository/Sam Mobile/Albums/2022/08 August/iPhone 12/20220818_130608 091_1609 iPhone 12.JPG", path "D:/Library/Mobile Repository/Sam Mobile/Albums/2022/08 August/iPhone 12/20220818_130608 121_0403 iPhone 12.JPG", path "D:/Library/Mobile Repository/Sam Mobile/Albums/2022/08 August/iPhone 12/20220820_125037 082_1609 iPhone 12.JPG", path "D:/Library/Mobile Repository/Sam Mobile/Albums/2022/08 August/iPhone 12/20220820_125037 091_1609 iPhone 12.JPG", path "D:/Library/Mobile Repository/Sam Mobile/Albums/2022/08 August/iPhone 12/20220820_125037 121_0403 iPhone 12.JPG", path "D:/Library/Mobile Repository/Sam Mobile/Albums/2022/08 August/iPhone 12/20220822_115113 082_1609 iPhone 12.JPG", path "D:/Library/Mobile Repository/Sam Mobile/Albums/2022/08 August/iPhone 12/20220822_115113 091_1609 iPhone 12.JPG", path "D:/Library/Mobile Repository/Sam Mobile/Albums/2022/08 August/iPhone 12/20220822_115113 121_0403 iPhone 12.JPG", path "D:/Library/Mobile Repository/Sam Mobile/Albums/2022/08 August/iPhone 12/20220822_115145 082_1609 iPhone 12.JPG", path "D:/Library/Mobile Repository/Sam Mobile/Albums/2022/08 August/iPhone 12/20220822_115145 091_1609 iPhone 12.JPG", path "D:/Library/Mobile Repository/Sam Mobile/Albums/2022/08 August/iPhone 12/20220822_115145 121_0403 iPhone 12.JPG", path "D:/Library/Mobile Repository/Sam Mobile/Albums/2022/08 August/iPhone 12/20220822_143820 082_1609 iPhone 12.JPG", path "D:/Library/Mobile Repository/Sam Mobile/Albums/2022/08 August/iPhone 12/20220822_143820 091_1609 iPhone 12.JPG", path "D:/Library/Mobile Repository/Sam Mobile/Albums/2022/08 August/iPhone 12/20220822_143820 121_0403 iPhone 12.JPG", path "D:/Library/Mobile Repository/Sam Mobile/Albums/2022/08 August/iPhone 12/20220823_112320 082_1609 iPhone 12.JPG", path "D:/Library/Mobile Repository/Sam Mobile/Albums/2022/08 August/iPhone 12/20220823_112320 091_1609 iPhone 12.JPG", path "D:/Library/Mobile Repository/Sam Mobile/Albums/2022/08 August/iPhone 12/20220823_112320 121_0403 iPhone 12.JPG", path "D:/Library/Mobile Repository/Sam Mobile/Albums/2022/08 August/iPhone 12/20220823_112408 082_1609 iPhone 12.JPG", path "D:/Library/Mobile Repository/Sam Mobile/Albums/2022/08 August/iPhone 12/20220823_112408 091_1609 iPhone 12.JPG", path "D:/Library/Mobile Repository/Sam Mobile/Albums/2022/08 August/iPhone 12/20220823_112408 121_0403 iPhone 12.JPG", path "D:/Library/Mobile Repository/Sam Mobile/Albums/2022/08 August/iPhone 12/20220825_070249 082_1609 iPhone 12.JPG", path "D:/Library/Mobile Repository/Sam Mobile/Albums/2022/08 August/iPhone 12/20220825_070249 121_0403 iPhone 12.JPG", path "D:/Library/Mobile Repository/Sam Mobile/Albums/2022/08 August/iPhone 12/20220825_115740 036_0000 iPhone 12.JPG", path "D:/Library/Mobile Repository/Sam Mobile/Albums/2022/08 August/iPhone 12/20220825_115740 121_0403 iPhone 12.JPG", path "D:/Library/Mobile Repository/Sam Mobile/Albums/2022/08 August/iPhone 12/20220826_165727 082_1609 iPhone 12.JPG", path "D:/Library/Mobile Repository/Sam Mobile/Albums/2022/08 August/iPhone 12/20220826_165727 091_1609 iPhone 12.JPG", path "D:/Library/Mobile Repository/Sam Mobile/Albums/2022/08 August/iPhone 12/20220826_165727 121_0403 iPhone 12.JPG", path "D:/Library/Mobile Repository/Sam Mobile/Albums/2022/08 August/iPhone 12/20220826_165751 082_1609 iPhone 12.JPG", path "D:/Library/Mobile Repository/Sam Mobile/Albums/2022/08 August/iPhone 12/20220826_165751 091_1609 iPhone 12.JPG", path "D:/Library/Mobile Repository/Sam Mobile/Albums/2022/08 August/iPhone 12/20220826_165751 121_0403 iPhone 12.JPG", path "D:/Library/Mobile Repository/Sam Mobile/Albums/2022/08 August/iPhone 12/20220826_165832 082_1609 iPhone 12.JPG", path "D:/Library/Mobile Repository/Sam Mobile/Albums/2022/08 August/iPhone 12/20220826_165832 091_1609 iPhone 12.JPG", path "D:/Library/Mobile Repository/Sam Mobile/Albums/2022/08 August/iPhone 12/20220826_165832 121_0403 iPhone 12.JPG", path "D:/Library/Mobile Repository/Sam Mobile/Albums/2022/08 August/iPhone 12/20220826_205412 082_1609 iPhone 12.JPG", path "D:/Library/Mobile Repository/Sam Mobile/Albums/2022/08 August/iPhone 12/20220826_205412 091_1609 iPhone 12.JPG", path "D:/Library/Mobile Repository/Sam Mobile/Albums/2022/08 August/iPhone 12/20220826_205412 121_0403 iPhone 12.JPG", path "D:/Library/Mobile Repository/Sam Mobile/Albums/2022/08 August/iPhone 12/20220826_205424 082_1609 iPhone 12.JPG", path "D:/Library/Mobile Repository/Sam Mobile/Albums/2022/08 August/iPhone 12/20220826_205424 091_1609 iPhone 12.JPG", path "D:/Library/Mobile Repository/Sam Mobile/Albums/2022/08 August/iPhone 12/20220826_205424 121_0403 iPhone 12.JPG", path "D:/Library/Mobile Repository/Sam Mobile/Albums/2022/08 August/iPhone 12/20220828_125812 082_1609 iPhone 12.JPG", path "D:/Library/Mobile Repository/Sam Mobile/Albums/2022/08 August/iPhone 12/20220828_125812 091_1609 iPhone 12.JPG", path "D:/Library/Mobile Repository/Sam Mobile/Albums/2022/08 August/iPhone 12/20220828_125812 121_0403 iPhone 12.JPG", path "D:/Library/Mobile Repository/Sam Mobile/Albums/2022/08 August/iPhone 12/20220828_131126 082_1609 iPhone 12.JPG", path "D:/Library/Mobile Repository/Sam Mobile/Albums/2022/08 August/iPhone 12/20220828_131126 091_1609 iPhone 12.JPG", path "D:/Library/Mobile Repository/Sam Mobile/Albums/2022/08 August/iPhone 12/20220828_131126 121_0403 iPhone 12.JPG", path "D:/Library/Mobile Repository/Sam Mobile/Albums/2022/08 August/iPhone 12/20220828_131147 082_1609 iPhone 12.JPG", path "D:/Library/Mobile Repository/Sam Mobile/Albums/2022/08 August/iPhone 12/20220828_131147 091_1609 iPhone 12.JPG", path "D:/Library/Mobile Repository/Sam Mobile/Albums/2022/08 August/iPhone 12/20220828_131147 121_0403 iPhone 12.JPG", path "D:/Library/Mobile Repository/Sam Mobile/Albums/2022/08 August/iPhone 12/20220828_131156 082_1609 iPhone 12.JPG", path "D:/Library/Mobile Repository/Sam Mobile/Albums/2022/08 August/iPhone 12/20220828_131156 091_1609 iPhone 12.JPG", path "D:/Library/Mobile Repository/Sam Mobile/Albums/2022/08 August/iPhone 12/20220828_131156 121_0403 iPhone 12.JPG", path "D:/Library/Mobile Repository/Sam Mobile/Albums/2022/08 August/iPhone 12/20220828_131159 082_1609 iPhone 12.JPG", path "D:/Library/Mobile Repository/Sam Mobile/Albums/2022/08 August/iPhone 12/20220828_131159 091_1609 iPhone 12.JPG", path "D:/Library/Mobile Repository/Sam Mobile/Albums/2022/08 August/iPhone 12/20220828_131159 121_0403 iPhone 12.JPG", path "D:/Library/Mobile Repository/Sam Mobile/Albums/2022/08 August/iPhone 12/20220828_131205 082_1609 iPhone 12.JPG", path "D:/Library/Mobile Repository/Sam Mobile/Albums/2022/08 August/iPhone 12/20220828_131205 091_1609 iPhone 12.JPG", path "D:/Library/Mobile Repository/Sam Mobile/Albums/2022/08 August/iPhone 12/20220828_131205 121_0403 iPhone 12.JPG", path "D:/Library/Mobile Repository/Sam Mobile/Albums/2022/08 August/iPhone 12/20220831_084100 024_0000 iPhone 12.JPG", path "D:/Library/Mobile Repository/Sam Mobile/Albums/2022/08 August/iPhone 12/20220831_084100 121_0403 iPhone 12.JPG", path "D:/Library/Mobile Repository/Sam Mobile/Albums/2022/09 September/iPhone 12/20220901_122010 082_1609 iPhone 12.JPG", path "D:/Library/Mobile Repository/Sam Mobile/Albums/2022/09 September/iPhone 12/20220901_122010 091_1609 iPhone 12.JPG", path "D:/Library/Mobile Repository/Sam Mobile/Albums/2022/09 September/iPhone 12/20220901_122010 121_0403 iPhone 12.JPG", path "D:/Library/Mobile Repository/Sam Mobile/Albums/2022/09 September/iPhone 12/20220901_144555 082_1609 iPhone 12.JPG", path "D:/Library/Mobile Repository/Sam Mobile/Albums/2022/09 September/iPhone 12/20220901_144555 091_1609 iPhone 12.JPG", path "D:/Library/Mobile Repository/Sam Mobile/Albums/2022/09 September/iPhone 12/20220901_144555 121_0403 iPhone 12.JPG", path "D:/Library/Mobile Repository/Sam Mobile/Albums/2022/09 September/iPhone 12/20220901_144609 082_1609 iPhone 12.JPG", path "D:/Library/Mobile Repository/Sam Mobile/Albums/2022/09 September/iPhone 12/20220901_144609 091_1609 iPhone 12.JPG", path "D:/Library/Mobile Repository/Sam Mobile/Albums/2022/09 September/iPhone 12/20220901_144609 121_0403 iPhone 12.JPG", path "D:/Library/Mobile Repository/Sam Mobile/Albums/2022/09 September/iPhone 12/20220903_175855 057_0000 iPhone 12.JPG", path "D:/Library/Mobile Repository/Sam Mobile/Albums/2022/09 September/iPhone 12/20220903_175855 121_0403 iPhone 12.JPG", path "D:/Library/Mobile Repository/Sam Mobile/Albums/2022/09 September/iPhone 12/20220906_124848 082_1609 iPhone 12.JPG", path "D:/Library/Mobile Repository/Sam Mobile/Albums/2022/09 September/iPhone 12/20220906_124848 091_1609 iPhone 12.JPG", path "D:/Library/Mobile Repository/Sam Mobile/Albums/2022/09 September/iPhone 12/20220906_124848 121_0403 iPhone 12.JPG", path "D:/Library/Mobile Repository/Sam Mobile/Albums/2022/09 September/iPhone 12/20220908_122004 082_1609 iPhone 12.JPG", path "D:/Library/Mobile Repository/Sam Mobile/Albums/2022/09 September/iPhone 12/20220908_122004 091_1609 iPhone 12.JPG", path "D:/Library/Mobile Repository/Sam Mobile/Albums/2022/09 September/iPhone 12/20220908_122004 121_0403 iPhone 12.JPG", path "D:/Library/Mobile Repository/Sam Mobile/Albums/2022/09 September/iPhone 12/20220908_122014 091_1609 iPhone 12.JPG", path "D:/Library/Mobile Repository/Sam Mobile/Albums/2022/09 September/iPhone 12/20220908_122014 121_0403 iPhone 12.JPG", path "D:/Library/Mobile Repository/Sam Mobile/Albums/2022/09 September/iPhone 12/20220908_122023 082_1609 iPhone 12.JPG", path "D:/Library/Mobile Repository/Sam Mobile/Albums/2022/09 September/iPhone 12/20220908_122023 091_1609 iPhone 12.JPG", path "D:/Library/Mobile Repository/Sam Mobile/Albums/2022/09 September/iPhone 12/20220908_122023 121_0403 iPhone 12.JPG", path "D:/Library/Mobile Repository/Sam Mobile/Albums/2022/09 September/iPhone 12/20220920_191733 067_0000 iPhone 12.JPG", path "D:/Library/Mobile Repository/Sam Mobile/Albums/2022/09 September/iPhone 12/20220920_191733 121_0403 iPhone 12.JPG", path "D:/Library/Mobile Repository/Sam Mobile/Albums/2022/09 September/iPhone 12/20220924_185958 082_1609 iPhone 12.JPG", path "D:/Library/Mobile Repository/Sam Mobile/Albums/2022/09 September/iPhone 12/20220924_185958 121_0403 iPhone 12.JPG", path "D:/Library/Mobile Repository/Sam Mobile/Albums/2022/09 September/iPhone 12/20220930_151054 082_1609 iPhone 12.JPG", path "D:/Library/Mobile Repository/Sam Mobile/Albums/2022/09 September/iPhone 12/20220930_151054 091_1609 iPhone 12.JPG", path "D:/Library/Mobile Repository/Sam Mobile/Albums/2022/09 September/iPhone 12/20220930_151054 121_0403 iPhone 12.JPG", path "D:/Library/Mobile Repository/Sam Mobile/Albums/2022/09 September/iPhone 12/20220930_151122 082_1609 iPhone 12.JPG", path "D:/Library/Mobile Repository/Sam Mobile/Albums/2022/09 September/iPhone 12/20220930_151122 091_1609 iPhone 12.JPG", path "D:/Library/Mobile Repository/Sam Mobile/Albums/2022/09 September/iPhone 12/20220930_151122 121_0403 iPhone 12.JPG", path "D:/Library/Mobile Repository/Sam Mobile/Albums/2022/09 September/iPhone 12/20220930_181647 091_0916 iPhone 12.JPG", path "D:/Library/Mobile Repository/Sam Mobile/Albums/2022/09 September/iPhone 12/20220930_181647 121_0403 iPhone 12.JPG", path "D:/Library/Mobile Repository/Sam Mobile/Albums/2022/09 September/iPhone 12/20220930_181655 082_1609 iPhone 12.JPG", path "D:/Library/Mobile Repository/Sam Mobile/Albums/2022/09 September/iPhone 12/20220930_181655 091_0916 iPhone 12.JPG", path "D:/Library/Mobile Repository/Sam Mobile/Albums/2022/09 September/iPhone 12/20220930_181655 121_0403 iPhone 12.JPG", path "D:/Library/Mobile Repository/Sam Mobile/Albums/2022/10 October/iPhone 12/20221001_171638 091_1609 iPhone 12.JPG", path "D:/Library/Mobile Repository/Sam Mobile/Albums/2022/10 October/iPhone 12/20221001_171638 121_0403 iPhone 12.JPG", path "D:/Library/Mobile Repository/Sam Mobile/Albums/2022/10 October/iPhone 12/20221001_172923 091_1609 iPhone 12.JPG", path "D:/Library/Mobile Repository/Sam Mobile/Albums/2022/10 October/iPhone 12/20221001_172923 121_0403 iPhone 12.JPG", path "D:/Library/Mobile Repository/Sam Mobile/Albums/2022/10 October/iPhone 12/20221002_113250 091_1609 iPhone 12.JPG", path "D:/Library/Mobile Repository/Sam Mobile/Albums/2022/10 October/iPhone 12/20221002_113250 121_0403 iPhone 12.JPG", path "D:/Library/Mobile Repository/Sam Mobile/Albums/2022/10 October/iPhone 12/20221002_180125 091_1609 iPhone 12.JPG", path "D:/Library/Mobile Repository/Sam Mobile/Albums/2022/10 October/iPhone 12/20221002_180125 121_0403 iPhone 12.JPG", path "D:/Library/Mobile Repository/Sam Mobile/Albums/2022/10 October/iPhone 12/20221002_214531 091_1609 iPhone 12.JPG", path "D:/Library/Mobile Repository/Sam Mobile/Albums/2022/10 October/iPhone 12/20221002_214531 121_0403 iPhone 12.JPG", path "D:/Library/Mobile Repository/Sam Mobile/Albums/2022/10 October/iPhone 12/20221002_214549 091_1609 iPhone 12.JPG", path "D:/Library/Mobile Repository/Sam Mobile/Albums/2022/10 October/iPhone 12/20221002_214549 121_0403 iPhone 12.JPG", path "D:/Library/Mobile Repository/Sam Mobile/Albums/2022/10 October/iPhone 12/20221002_214608 091_1609 iPhone 12.JPG", path "D:/Library/Mobile Repository/Sam Mobile/Albums/2022/10 October/iPhone 12/20221002_214608 121_0403 iPhone 12.JPG", path "D:/Library/Mobile Repository/Sam Mobile/Albums/2022/10 October/iPhone 12/20221002_214628 091_1609 iPhone 12.JPG", path "D:/Library/Mobile Repository/Sam Mobile/Albums/2022/10 October/iPhone 12/20221002_214628 121_0403 iPhone 12.JPG", path "D:/Library/Mobile Repository/Sam Mobile/Albums/2022/10 October/iPhone 12/20221002_214630 091_1609 iPhone 12.JPG", path "D:/Library/Mobile Repository/Sam Mobile/Albums/2022/10 October/iPhone 12/20221002_214630 121_0403 iPhone 12.JPG", path "D:/Library/Mobile Repository/Sam Mobile/Albums/2022/10 October/iPhone 12/20221003_205859 091_1609 iPhone 12.JPG", path "D:/Library/Mobile Repository/Sam Mobile/Albums/2022/10 October/iPhone 12/20221003_205859 121_0403 iPhone 12.JPG", path "D:/Library/Mobile Repository/Sam Mobile/Albums/2022/10 October/iPhone 12/20221004_114948 074_0000 iPhone 12.JPG", path "D:/Library/Mobile Repository/Sam Mobile/Albums/2022/10 October/iPhone 12/20221004_114948 121_0403 iPhone 12.JPG", path "D:/Library/Mobile Repository/Sam Mobile/Albums/2022/10 October/iPhone 12/20221004_164809 034_0000 iPhone 12.JPG", path "D:/Library/Mobile Repository/Sam Mobile/Albums/2022/10 October/iPhone 12/20221004_164809 121_0403 iPhone 12.JPG", path "D:/Library/Mobile Repository/Sam Mobile/Albums/2022/10 October/iPhone 12/20221005_110828 054_0000 iPhone 12.JPG", path "D:/Library/Mobile Repository/Sam Mobile/Albums/2022/10 October/iPhone 12/20221005_110828 121_0403 iPhone 12.JPG", path "D:/Library/Mobile Repository/Sam Mobile/Albums/2022/10 October/iPhone 12/20221010_131252 091_1609 iPhone 12.JPG", path "D:/Library/Mobile Repository/Sam Mobile/Albums/2022/10 October/iPhone 12/20221010_131252 121_0403 iPhone 12.JPG", path "D:/Library/Mobile Repository/Sam Mobile/Albums/2022/10 October/iPhone 12/20221010_131327 091_1609 iPhone 12.JPG", path "D:/Library/Mobile Repository/Sam Mobile/Albums/2022/10 October/iPhone 12/20221010_131327 121_0403 iPhone 12.JPG", path "D:/Library/Mobile Repository/Sam Mobile/Albums/2022/10 October/iPhone 12/20221010_142325 091_1609 iPhone 12.JPG", path "D:/Library/Mobile Repository/Sam Mobile/Albums/2022/10 October/iPhone 12/20221010_142325 121_0403 iPhone 12.JPG", path "D:/Library/Mobile Repository/Sam Mobile/Albums/2022/10 October/iPhone 12/20221014_090704 091_1609 iPhone 12.JPG", path "D:/Library/Mobile Repository/Sam Mobile/Albums/2022/10 October/iPhone 12/20221014_090704 121_0403 iPhone 12.JPG", path "D:/Library/Mobile Repository/Sam Mobile/Albums/2022/10 October/iPhone 12/20221014_090708 091_1609 iPhone 12.JPG", path "D:/Library/Mobile Repository/Sam Mobile/Albums/2022/10 October/iPhone 12/20221014_090708 121_0403 iPhone 12.JPG", path "D:/Library/Mobile Repository/Sam Mobile/Albums/2022/10 October/iPhone 12/20221018_180334 091_1609 iPhone 12.JPG", path "D:/Library/Mobile Repository/Sam Mobile/Albums/2022/10 October/iPhone 12/20221018_180334 121_0403 iPhone 12.JPG", path "D:/Library/Mobile Repository/Sam Mobile/Albums/2022/10 October/iPhone 12/20221024_190050 091_1609 iPhone 12.JPG", path "D:/Library/Mobile Repository/Sam Mobile/Albums/2022/10 October/iPhone 12/20221024_190050 121_0403 iPhone 12.JPG", path "D:/Library/Mobile Repository/Sam Mobile/Albums/2022/10 October/iPhone 12/20221024_190326 091_1609 iPhone 12.JPG", path "D:/Library/Mobile Repository/Sam Mobile/Albums/2022/10 October/iPhone 12/20221024_190326 121_0403 iPhone 12.JPG", path "D:/Library/Mobile Repository/Sam Mobile/Albums/2022/10 October/iPhone 12/20221024_190342 091_1609 iPhone 12.JPG", path "D:/Library/Mobile Repository/Sam Mobile/Albums/2022/10 October/iPhone 12/20221024_190342 121_0403 iPhone 12.JPG", path "D:/Library/Mobile Repository/Sam Mobile/Albums/2022/10 October/iPhone 12/20221028_131826 091_1609 iPhone 12.JPG", path "D:/Library/Mobile Repository/Sam Mobile/Albums/2022/10 October/iPhone 12/20221028_131826 121_0403 iPhone 12.JPG", path "D:/Library/Mobile Repository/Sam Mobile/Albums/2022/10 October/iPhone 12/20221028_221816 091_1609 iPhone 12.JPG", path "D:/Library/Mobile Repository/Sam Mobile/Albums/2022/10 October/iPhone 12/20221028_221816 121_0403 iPhone 12.JPG", path "D:/Library/Mobile Repository/Sam Mobile/Albums/2022/10 October/iPhone 12/20221028_221839 091_1609 iPhone 12.JPG", path "D:/Library/Mobile Repository/Sam Mobile/Albums/2022/10 October/iPhone 12/20221028_221839 121_0403 iPhone 12.JPG", path "D:/Library/Mobile Repository/Sam Mobile/Albums/2022/10 October/iPhone 12/20221029_124323 091_1609 iPhone 12.JPG", path "D:/Library/Mobile Repository/Sam Mobile/Albums/2022/10 October/iPhone 12/20221029_124323 121_0403 iPhone 12.JPG", path "D:/Library/Mobile Repository/Sam Mobile/Albums/2022/10 October/iPhone 12/20221029_124343 091_1609 iPhone 12.JPG", path "D:/Library/Mobile Repository/Sam Mobile/Albums/2022/10 October/iPhone 12/20221029_124343 121_0403 iPhone 12.JPG", path "D:/Library/Mobile Repository/Sam Mobile/Albums/2022/11 November/iPhone 12/20221102_180104 091_1609 iPhone 12.JPG", path "D:/Library/Mobile Repository/Sam Mobile/Albums/2022/11 November/iPhone 12/20221102_180104 121_0403 iPhone 12.JPG", path "D:/Library/Mobile Repository/Sam Mobile/Albums/2022/11 November/iPhone 12/20221103_133443 091_0000 iPhone 12.JPG", path "D:/Library/Mobile Repository/Sam Mobile/Albums/2022/11 November/iPhone 12/20221103_133443 121_0403 iPhone 12.JPG", path "D:/Library/Mobile Repository/Sam Mobile/Albums/2022/11 November/iPhone 12/20221105_173130 091_1609 iPhone 12.JPG", path "D:/Library/Mobile Repository/Sam Mobile/Albums/2022/11 November/iPhone 12/20221105_173130 121_0403 iPhone 12.JPG", path "D:/Library/Mobile Repository/Sam Mobile/Albums/2022/11 November/iPhone 12/20221106_083229 091_1609 iPhone 12.JPG", path "D:/Library/Mobile Repository/Sam Mobile/Albums/2022/11 November/iPhone 12/20221106_083229 121_0403 iPhone 12.JPG", path "D:/Library/Mobile Repository/Sam Mobile/Albums/2022/11 November/iPhone 12/20221108_184055 091_1609 iPhone 12.JPG", path "D:/Library/Mobile Repository/Sam Mobile/Albums/2022/11 November/iPhone 12/20221108_184055 121_0403 iPhone 12.JPG", path "D:/Library/Mobile Repository/Sam Mobile/Albums/2022/11 November/iPhone 12/20221109_220358 091_1609 iPhone 12.JPG", path "D:/Library/Mobile Repository/Sam Mobile/Albums/2022/11 November/iPhone 12/20221109_220358 121_0403 iPhone 12.JPG", path "D:/Library/Mobile Repository/Sam Mobile/Albums/2022/11 November/iPhone 12/20221110_155751 091_1609 iPhone 12.JPG", path "D:/Library/Mobile Repository/Sam Mobile/Albums/2022/11 November/iPhone 12/20221110_155751 121_0403 iPhone 12.JPG", path "D:/Library/Mobile Repository/Sam Mobile/Albums/2022/11 November/iPhone 12/20221110_155910 091_1609 iPhone 12.JPG", path "D:/Library/Mobile Repository/Sam Mobile/Albums/2022/11 November/iPhone 12/20221110_155910 121_0403 iPhone 12.JPG", path "D:/Library/Mobile Repository/Sam Mobile/Albums/2022/11 November/iPhone 12/20221110_160149 091_1609 iPhone 12.JPG", path "D:/Library/Mobile Repository/Sam Mobile/Albums/2022/11 November/iPhone 12/20221110_160149 121_0403 iPhone 12.JPG", path "D:/Library/Mobile Repository/Sam Mobile/Albums/2022/11 November/iPhone 12/20221110_160204 091_1609 iPhone 12.JPG", path "D:/Library/Mobile Repository/Sam Mobile/Albums/2022/11 November/iPhone 12/20221110_160204 121_0403 iPhone 12.JPG", path "D:/Library/Mobile Repository/Sam Mobile/Albums/2022/11 November/iPhone 12/20221110_204226 091_1609 iPhone 12.JPG", path "D:/Library/Mobile Repository/Sam Mobile/Albums/2022/11 November/iPhone 12/20221110_204226 121_0403 iPhone 12.JPG", path "D:/Library/Mobile Repository/Sam Mobile/Albums/2022/11 November/iPhone 12/20221111_103731 091_1609 iPhone 12.JPG", path "D:/Library/Mobile Repository/Sam Mobile/Albums/2022/11 November/iPhone 12/20221111_103731 121_0403 iPhone 12.JPG", path "D:/Library/Mobile Repository/Sam Mobile/Albums/2022/11 November/iPhone 12/20221111_103755 091_1609 iPhone 12.JPG", path "D:/Library/Mobile Repository/Sam Mobile/Albums/2022/11 November/iPhone 12/20221111_103755 121_0403 iPhone 12.JPG", path "D:/Library/Mobile Repository/Sam Mobile/Albums/2022/11 November/iPhone 12/20221113_085644 091_1609 iPhone 12.JPG", path "D:/Library/Mobile Repository/Sam Mobile/Albums/2022/11 November/iPhone 12/20221113_085644 121_0403 iPhone 12.JPG", path "D:/Library/Mobile Repository/Sam Mobile/Albums/2022/11 November/iPhone 12/20221113_085726 091_1609 iPhone 12.JPG", path "D:/Library/Mobile Repository/Sam Mobile/Albums/2022/11 November/iPhone 12/20221113_085726 121_0403 iPhone 12.JPG", path "D:/Library/Mobile Repository/Sam Mobile/Albums/2022/11 November/iPhone 12/20221113_085812 091_1609 iPhone 12.JPG", path "D:/Library/Mobile Repository/Sam Mobile/Albums/2022/11 November/iPhone 12/20221113_085812 121_0403 iPhone 12.JPG", path "D:/Library/Mobile Repository/Sam Mobile/Albums/2022/11 November/iPhone 12/20221113_085942 091_1609 iPhone 12.JPG", path "D:/Library/Mobile Repository/Sam Mobile/Albums/2022/11 November/iPhone 12/20221113_085942 121_0403 iPhone 12.JPG", path "D:/Library/Mobile Repository/Sam Mobile/Albums/2022/11 November/iPhone 12/20221113_090308 091_1609 iPhone 12.JPG", path "D:/Library/Mobile Repository/Sam Mobile/Albums/2022/11 November/iPhone 12/20221113_090308 121_0403 iPhone 12.JPG", path "D:/Library/Mobile Repository/Sam Mobile/Albums/2022/11 November/iPhone 12/20221113_090522 091_1609 iPhone 12.JPG", path "D:/Library/Mobile Repository/Sam Mobile/Albums/2022/11 November/iPhone 12/20221113_090522 121_0403 iPhone 12.JPG", path "D:/Library/Mobile Repository/Sam Mobile/Albums/2022/11 November/iPhone 12/20221113_092056 091_1609 iPhone 12.JPG", path "D:/Library/Mobile Repository/Sam Mobile/Albums/2022/11 November/iPhone 12/20221113_092056 121_0403 iPhone 12.JPG", path "D:/Library/Mobile Repository/Sam Mobile/Albums/2022/11 November/iPhone 12/20221115_102502 091_1609 iPhone 12.JPG", path "D:/Library/Mobile Repository/Sam Mobile/Albums/2022/11 November/iPhone 12/20221115_102502 121_0403 iPhone 12.JPG", path "D:/Library/Mobile Repository/Sam Mobile/Albums/2022/11 November/iPhone 12/20221116_105438 091_1609 iPhone 12.JPG", path "D:/Library/Mobile Repository/Sam Mobile/Albums/2022/11 November/iPhone 12/20221116_105438 121_0403 iPhone 12.JPG", path "D:/Library/Mobile Repository/Sam Mobile/Albums/2022/11 November/iPhone 12/20221116_105458 091_1609 iPhone 12.JPG", path "D:/Library/Mobile Repository/Sam Mobile/Albums/2022/11 November/iPhone 12/20221116_105458 121_0403 iPhone 12.JPG", path "D:/Library/Mobile Repository/Sam Mobile/Albums/2022/11 November/iPhone 12/20221116_105544 091_1609 iPhone 12.JPG", path "D:/Library/Mobile Repository/Sam Mobile/Albums/2022/11 November/iPhone 12/20221116_105544 121_0403 iPhone 12.JPG", path "D:/Library/Mobile Repository/Sam Mobile/Albums/2022/11 November/iPhone 12/20221118_165536 057_0000 iPhone 12.JPG", path "D:/Library/Mobile Repository/Sam Mobile/Albums/2022/11 November/iPhone 12/20221118_165536 121_0403 iPhone 12.JPG", path "D:/Library/Mobile Repository/Sam Mobile/Albums/2022/11 November/iPhone 12/20221119_145215 091_1609 iPhone 12.JPG", path "D:/Library/Mobile Repository/Sam Mobile/Albums/2022/11 November/iPhone 12/20221119_145215 121_0403 iPhone 12.JPG", path "D:/Library/Mobile Repository/Sam Mobile/Albums/2022/11 November/iPhone 12/20221119_145217 091_1609 iPhone 12.JPG", path "D:/Library/Mobile Repository/Sam Mobile/Albums/2022/11 November/iPhone 12/20221119_145217 121_0403 iPhone 12.JPG", path "D:/Library/Mobile Repository/Sam Mobile/Albums/2022/11 November/iPhone 12/20221123_181425 091_1609 iPhone 12.JPG", path "D:/Library/Mobile Repository/Sam Mobile/Albums/2022/11 November/iPhone 12/20221123_181425 121_0403 iPhone 12.JPG", path "D:/Library/Mobile Repository/Sam Mobile/Albums/2022/11 November/iPhone 12/20221123_181459 091_1609 iPhone 12.JPG", path "D:/Library/Mobile Repository/Sam Mobile/Albums/2022/11 November/iPhone 12/20221123_181459 121_0403 iPhone 12.JPG", path "D:/Library/Mobile Repository/Sam Mobile/Albums/2022/11 November/iPhone 12/20221123_181503 091_1609 iPhone 12.JPG", path "D:/Library/Mobile Repository/Sam Mobile/Albums/2022/11 November/iPhone 12/20221123_181503 121_0403 iPhone 12.JPG", path "D:/Library/Mobile Repository/Sam Mobile/Albums/2022/11 November/iPhone 12/20221125_102948 033_0101 iPhone 12.JPG", path "D:/Library/Mobile Repository/Sam Mobile/Albums/2022/11 November/iPhone 12/20221125_102948 121_0403 iPhone 12.JPG", path "D:/Library/Mobile Repository/Sam Mobile/Albums/2022/11 November/iPhone 12/20221127_202836 091_1609 iPhone 12.JPG", path "D:/Library/Mobile Repository/Sam Mobile/Albums/2022/11 November/iPhone 12/20221127_202836 121_0403 iPhone 12.JPG", path "D:/Library/Mobile Repository/Sam Mobile/Albums/2022/11 November/iPhone 12/20221128_122430 091_1609 iPhone 12.JPG", path "D:/Library/Mobile Repository/Sam Mobile/Albums/2022/11 November/iPhone 12/20221128_122430 121_0403 iPhone 12.JPG", path "D:/Library/Mobile Repository/Sam Mobile/Albums/2022/11 November/iPhone 12/20221128_122532 091_1609 iPhone 12.JPG", path "D:/Library/Mobile Repository/Sam Mobile/Albums/2022/11 November/iPhone 12/20221128_122532 121_0403 iPhone 12.JPG", path "D:/Library/Mobile Repository/Sam Mobile/Albums/2022/11 November/iPhone 12/20221129_130500 091_1609 iPhone 12.JPG", path "D:/Library/Mobile Repository/Sam Mobile/Albums/2022/11 November/iPhone 12/20221129_130500 121_0403 iPhone 12.JPG", path "D:/Library/Mobile Repository/Sam Mobile/Albums/2022/11 November/iPhone 12/20221129_130826 091_1609 iPhone 12.JPG", path "D:/Library/Mobile Repository/Sam Mobile/Albums/2022/11 November/iPhone 12/20221129_130826 121_0403 iPhone 12.JPG", path "D:/Library/Mobile Repository/Sam Mobile/Albums/2022/11 November/iPhone 12/20221130_194654 091_1609 iPhone 12.JPG", path "D:/Library/Mobile Repository/Sam Mobile/Albums/2022/11 November/iPhone 12/20221130_194654 121_0403 iPhone 12.JPG", path "D:/Library/Mobile Repository/Sam Mobile/Albums/2022/11 November/iPhone 12/20221130_194659 091_1609 iPhone 12.JPG", path "D:/Library/Mobile Repository/Sam Mobile/Albums/2022/11 November/iPhone 12/20221130_194659 121_0403 iPhone 12.JPG", path "D:/Library/Mobile Repository/Sam Mobile/Albums/2022/11 November/iPhone 12/20221130_194709 091_1609 iPhone 12.JPG", path "D:/Library/Mobile Repository/Sam Mobile/Albums/2022/11 November/iPhone 12/20221130_194709 121_0403 iPhone 12.JPG", path "D:/Library/Mobile Repository/Sam Mobile/Albums/2022/11 November/iPhone 12/20221130_194713 091_1609 iPhone 12.JPG", path "D:/Library/Mobile Repository/Sam Mobile/Albums/2022/11 November/iPhone 12/20221130_194713 121_0403 iPhone 12.JPG", path "D:/Library/Mobile Repository/Sam Mobile/Albums/2022/11 November/iPhone 12/20221130_194730 091_1609 iPhone 12.JPG", path "D:/Library/Mobile Repository/Sam Mobile/Albums/2022/11 November/iPhone 12/20221130_194730 121_0403 iPhone 12.JPG", path "D:/Library/Mobile Repository/Sam Mobile/Albums/2022/11 November/iPhone 12/20221130_194739 091_1609 iPhone 12.JPG", path "D:/Library/Mobile Repository/Sam Mobile/Albums/2022/11 November/iPhone 12/20221130_194739 121_0403 iPhone 12.JPG", path "D:/Library/Mobile Repository/Sam Mobile/Albums/2022/11 November/iPhone 12/20221130_194756 091_1609 iPhone 12.JPG", path "D:/Library/Mobile Repository/Sam Mobile/Albums/2022/11 November/iPhone 12/20221130_194756 121_0403 iPhone 12.JPG", path "D:/Library/Mobile Repository/Sam Mobile/Albums/2022/11 November/iPhone 12/20221130_194801 091_1609 iPhone 12.JPG", path "D:/Library/Mobile Repository/Sam Mobile/Albums/2022/11 November/iPhone 12/20221130_194801 121_0403 iPhone 12.JPG", path "D:/Library/Mobile Repository/Sam Mobile/Albums/2022/11 November/iPhone 12/20221130_195016 091_1609 iPhone 12.JPG", path "D:/Library/Mobile Repository/Sam Mobile/Albums/2022/11 November/iPhone 12/20221130_195016 121_0403 iPhone 12.JPG", path "D:/Library/Mobile Repository/Sam Mobile/Albums/2022/11 November/iPhone 12/20221130_195020 091_1609 iPhone 12.JPG", path "D:/Library/Mobile Repository/Sam Mobile/Albums/2022/11 November/iPhone 12/20221130_195020 121_0403 iPhone 12.JPG", path "D:/Library/Mobile Repository/Sam Mobile/Albums/2022/11 November/iPhone 12/20221130_195345 091_1609 iPhone 12.JPG", path "D:/Library/Mobile Repository/Sam Mobile/Albums/2022/11 November/iPhone 12/20221130_195345 121_0403 iPhone 12.JPG", path "D:/Library/Mobile Repository/Sam Mobile/Albums/2022/11 November/iPhone 12/20221130_195350 091_1609 iPhone 12.JPG", path "D:/Library/Mobile Repository/Sam Mobile/Albums/2022/11 November/iPhone 12/20221130_195350 121_0403 iPhone 12.JPG", path "D:/Library/Mobile Repository/Sam Mobile/Albums/2022/12 December/iPhone 12/20221202_185554 091_1609 iPhone 12.JPG", path "D:/Library/Mobile Repository/Sam Mobile/Albums/2022/12 December/iPhone 12/20221202_185554 121_0403 iPhone 12.JPG", path "D:/Library/Mobile Repository/Sam Mobile/Albums/2022/12 December/iPhone 12/20221202_185559 091_1609 iPhone 12.JPG", path "D:/Library/Mobile Repository/Sam Mobile/Albums/2022/12 December/iPhone 12/20221202_185559 121_0403 iPhone 12.JPG", path "D:/Library/Mobile Repository/Sam Mobile/Albums/2022/12 December/iPhone 12/20221202_185604 091_1609 iPhone 12.JPG", path "D:/Library/Mobile Repository/Sam Mobile/Albums/2022/12 December/iPhone 12/20221202_185604 121_0403 iPhone 12.JPG", path "D:/Library/Mobile Repository/Sam Mobile/Albums/2022/12 December/iPhone 12/20221203_135533 086_0000 iPhone 12.JPG", path "D:/Library/Mobile Repository/Sam Mobile/Albums/2022/12 December/iPhone 12/20221203_135533 121_0403 iPhone 12.JPG", path "D:/Library/Mobile Repository/Sam Mobile/Albums/2022/12 December/iPhone 12/20221203_135603 091_1609 iPhone 12.JPG", path "D:/Library/Mobile Repository/Sam Mobile/Albums/2022/12 December/iPhone 12/20221203_135603 121_0403 iPhone 12.JPG", path "D:/Library/Mobile Repository/Sam Mobile/Albums/2022/12 December/iPhone 12/20221210_080935 091_1609 iPhone 12.JPG", path "D:/Library/Mobile Repository/Sam Mobile/Albums/2022/12 December/iPhone 12/20221210_080935 121_0403 iPhone 12.JPG", path "D:/Library/Mobile Repository/Sam Mobile/Albums/2022/12 December/iPhone 12/20221210_080950 091_1609 iPhone 12.JPG", path "D:/Library/Mobile Repository/Sam Mobile/Albums/2022/12 December/iPhone 12/20221210_080950 121_0403 iPhone 12.JPG", path "D:/Library/Mobile Repository/Sam Mobile/Albums/2022/12 December/iPhone 12/20221213_164523 091_1609 iPhone 12.JPG", path "D:/Library/Mobile Repository/Sam Mobile/Albums/2022/12 December/iPhone 12/20221213_164523 121_0403 iPhone 12.JPG", path "D:/Library/Mobile Repository/Sam Mobile/Albums/2022/12 December/iPhone 12/20221218_221100 091_1609 iPhone 12.JPG", path "D:/Library/Mobile Repository/Sam Mobile/Albums/2022/12 December/iPhone 12/20221218_221100 121_0403 iPhone 12.JPG", path "D:/Library/Mobile Repository/Sam Mobile/Albums/2022/12 December/iPhone 12/20221218_231342 091_1609 iPhone 12.JPG", path "D:/Library/Mobile Repository/Sam Mobile/Albums/2022/12 December/iPhone 12/20221218_231342 121_0403 iPhone 12.JPG", path "D:/Library/Mobile Repository/Sam Mobile/Albums/2022/12 December/iPhone 12/20221219_000101 091_1609 iPhone 12.JPG", path "D:/Library/Mobile Repository/Sam Mobile/Albums/2022/12 December/iPhone 12/20221219_000101 121_0403 iPhone 12.JPG", path "D:/Library/Mobile Repository/Sam Mobile/Albums/2022/12 December/iPhone 12/20221219_000121 091_1609 iPhone 12.JPG", path "D:/Library/Mobile Repository/Sam Mobile/Albums/2022/12 December/iPhone 12/20221219_000121 121_0403 iPhone 12.JPG", path "D:/Library/Mobile Repository/Sam Mobile/Albums/2022/12 December/iPhone 12/20221219_000125 091_1609 iPhone 12.JPG", path "D:/Library/Mobile Repository/Sam Mobile/Albums/2022/12 December/iPhone 12/20221219_000125 121_0403 iPhone 12.JPG", path "D:/Library/Mobile Repository/Sam Mobile/Albums/2022/12 December/iPhone 12/20221219_000142 091_1609 iPhone 12.JPG", path "D:/Library/Mobile Repository/Sam Mobile/Albums/2022/12 December/iPhone 12/20221219_000142 121_0403 iPhone 12.JPG", path "D:/Library/Mobile Repository/Sam Mobile/Albums/2022/12 December/iPhone 12/20221219_000153 091_1609 iPhone 12.JPG", path "D:/Library/Mobile Repository/Sam Mobile/Albums/2022/12 December/iPhone 12/20221219_000153 121_0403 iPhone 12.JPG", path "D:/Library/Mobile Repository/Sam Mobile/Albums/2022/12 December/iPhone 12/20221219_000200 091_1609 iPhone 12.JPG", path "D:/Library/Mobile Repository/Sam Mobile/Albums/2022/12 December/iPhone 12/20221219_000200 121_0403 iPhone 12.JPG", path "D:/Library/Mobile Repository/Sam Mobile/Albums/2022/12 December/iPhone 12/20221219_000215 091_1609 iPhone 12.JPG", path "D:/Library/Mobile Repository/Sam Mobile/Albums/2022/12 December/iPhone 12/20221219_000215 121_0403 iPhone 12.JPG", path "D:/Library/Mobile Repository/Sam Mobile/Albums/2022/12 December/iPhone 12/20221219_000218 091_1609 iPhone 12.JPG", path "D:/Library/Mobile Repository/Sam Mobile/Albums/2022/12 December/iPhone 12/20221219_000218 121_0403 iPhone 12.JPG", path "D:/Library/Mobile Repository/Sam Mobile/Albums/2022/12 December/iPhone 12/20221219_122627 091_1609 iPhone 12.JPG", path "D:/Library/Mobile Repository/Sam Mobile/Albums/2022/12 December/iPhone 12/20221219_122627 121_0403 iPhone 12.JPG", path "D:/Library/Mobile Repository/Sam Mobile/Albums/2022/12 December/iPhone 12/20221222_173822 091_1609 iPhone 12.JPG", path "D:/Library/Mobile Repository/Sam Mobile/Albums/2022/12 December/iPhone 12/20221222_173822 121_0403 iPhone 12.JPG", path "D:/Library/Mobile Repository/Sam Mobile/Albums/2022/12 December/iPhone 12/20221222_174058 091_1609 iPhone 12.JPG", path "D:/Library/Mobile Repository/Sam Mobile/Albums/2022/12 December/iPhone 12/20221222_174058 121_0403 iPhone 12.JPG", path "D:/Library/Mobile Repository/Sam Mobile/Albums/2022/12 December/iPhone 12/20221222_174108 091_1609 iPhone 12.JPG", path "D:/Library/Mobile Repository/Sam Mobile/Albums/2022/12 December/iPhone 12/20221222_174108 121_0403 iPhone 12.JPG", path "D:/Library/Mobile Repository/Sam Mobile/Albums/2022/12 December/iPhone 12/20221223_151618 091_1609 iPhone 12.JPG", path "D:/Library/Mobile Repository/Sam Mobile/Albums/2022/12 December/iPhone 12/20221223_151618 121_0403 iPhone 12.JPG", path "D:/Library/Mobile Repository/Sam Mobile/Albums/2022/12 December/iPhone 12/20221223_160733 091_1609 iPhone 12.JPG", path "D:/Library/Mobile Repository/Sam Mobile/Albums/2022/12 December/iPhone 12/20221223_160733 121_0403 iPhone 12.JPG", path "D:/Library/Mobile Repository/Sam Mobile/Albums/2022/12 December/iPhone 12/20221224_114759 091_1609 iPhone 12.JPG", path "D:/Library/Mobile Repository/Sam Mobile/Albums/2022/12 December/iPhone 12/20221224_114759 121_0403 iPhone 12.JPG", path "D:/Library/Mobile Repository/Sam Mobile/Albums/2022/12 December/iPhone 12/20221225_083005 091_1609 iPhone 12.JPG", path "D:/Library/Mobile Repository/Sam Mobile/Albums/2022/12 December/iPhone 12/20221225_083005 121_0403 iPhone 12.JPG", path "D:/Library/Mobile Repository/Sam Mobile/Albums/2022/12 December/iPhone 12/20221225_144421 091_1609 iPhone 12.JPG", path "D:/Library/Mobile Repository/Sam Mobile/Albums/2022/12 December/iPhone 12/20221225_144421 121_0403 iPhone 12.JPG", path "D:/Library/Mobile Repository/Sam Mobile/Albums/2022/12 December/iPhone 12/20221225_144444 091_1609 iPhone 12.JPG", path "D:/Library/Mobile Repository/Sam Mobile/Albums/2022/12 December/iPhone 12/20221225_144444 121_0403 iPhone 12.JPG", path "D:/Library/Mobile Repository/Sam Mobile/Albums/2022/12 December/iPhone 12/20221225_144448 091_1609 iPhone 12.JPG", path "D:/Library/Mobile Repository/Sam Mobile/Albums/2022/12 December/iPhone 12/20221225_144448 121_0403 iPhone 12.JPG", path "D:/Library/Mobile Repository/Sam Mobile/Albums/2022/12 December/iPhone 12/20221225_144500 091_1609 iPhone 12.JPG", path "D:/Library/Mobile Repository/Sam Mobile/Albums/2022/12 December/iPhone 12/20221225_144500 121_0403 iPhone 12.JPG", path "D:/Library/Mobile Repository/Sam Mobile/Albums/2022/12 December/iPhone 12/20221225_144509 091_1609 iPhone 12.JPG", path "D:/Library/Mobile Repository/Sam Mobile/Albums/2022/12 December/iPhone 12/20221225_144509 121_0403 iPhone 12.JPG", path "D:/Library/Mobile Repository/Sam Mobile/Albums/2023/01 January/iPhone 12/20230102_205936 091_1609 iPhone 12.JPG", path "D:/Library/Mobile Repository/Sam Mobile/Albums/2023/01 January/iPhone 12/20230102_205936 121_0403 iPhone 12.JPG", path "D:/Library/Mobile Repository/Sam Mobile/Albums/2023/01 January/iPhone 12/20230102_205944 091_1609 iPhone 12.JPG", path "D:/Library/Mobile Repository/Sam Mobile/Albums/2023/01 January/iPhone 12/20230102_205944 121_0403 iPhone 12.JPG", path "D:/Library/Mobile Repository/Sam Mobile/Albums/2023/01 January/iPhone 12/20230102_210004 091_1609 iPhone 12.JPG", path "D:/Library/Mobile Repository/Sam Mobile/Albums/2023/01 January/iPhone 12/20230102_210004 121_0403 iPhone 12.JPG", path "D:/Library/Mobile Repository/Sam Mobile/Albums/2023/01 January/iPhone 12/20230102_210012 091_1609 iPhone 12.JPG", path "D:/Library/Mobile Repository/Sam Mobile/Albums/2023/01 January/iPhone 12/20230102_210012 121_0403 iPhone 12.JPG", path "D:/Library/Mobile Repository/Sam Mobile/Albums/2023/01 January/iPhone 12/20230102_210022 091_1609 iPhone 12.JPG", path "D:/Library/Mobile Repository/Sam Mobile/Albums/2023/01 January/iPhone 12/20230102_210022 121_0403 iPhone 12.JPG", path "D:/Library/Mobile Repository/Sam Mobile/Albums/2023/01 January/iPhone 12/20230102_212104 091_1609 iPhone 12.JPG", path "D:/Library/Mobile Repository/Sam Mobile/Albums/2023/01 January/iPhone 12/20230102_212104 121_0403 iPhone 12.JPG", path "D:/Library/Mobile Repository/Sam Mobile/Albums/2023/01 January/iPhone 12/20230102_212123 091_1609 iPhone 12.JPG", path "D:/Library/Mobile Repository/Sam Mobile/Albums/2023/01 January/iPhone 12/20230102_212123 121_0403 iPhone 12.JPG", path "D:/Library/Mobile Repository/Sam Mobile/Albums/2023/01 January/iPhone 12/20230102_212128 091_1609 iPhone 12.JPG", path "D:/Library/Mobile Repository/Sam Mobile/Albums/2023/01 January/iPhone 12/20230102_212128 121_0403 iPhone 12.JPG", path "D:/Library/Mobile Repository/Sam Mobile/Albums/2023/01 January/iPhone 12/20230102_212138 091_1609 iPhone 12.JPG", path "D:/Library/Mobile Repository/Sam Mobile/Albums/2023/01 January/iPhone 12/20230102_212138 121_0403 iPhone 12.JPG", path "D:/Library/Mobile Repository/Sam Mobile/Albums/2023/01 January/iPhone 12/20230102_212227 091_1609 iPhone 12.JPG", path "D:/Library/Mobile Repository/Sam Mobile/Albums/2023/01 January/iPhone 12/20230102_212227 121_0403 iPhone 12.JPG", path "D:/Library/Mobile Repository/Sam Mobile/Albums/2023/01 January/iPhone 12/20230106_083616 091_1609 iPhone 12.JPG", path "D:/Library/Mobile Repository/Sam Mobile/Albums/2023/01 January/iPhone 12/20230106_083616 121_0403 iPhone 12.JPG", path "D:/Library/Mobile Repository/Sam Mobile/Albums/2023/01 January/iPhone 12/20230106_083619 091_1609 iPhone 12.JPG", path "D:/Library/Mobile Repository/Sam Mobile/Albums/2023/01 January/iPhone 12/20230106_083619 121_0403 iPhone 12.JPG", path "D:/Library/Mobile Repository/Sam Mobile/Albums/2023/01 January/iPhone 12/20230106_095742 091_1609 iPhone 12.JPG", path "D:/Library/Mobile Repository/Sam Mobile/Albums/2023/01 January/iPhone 12/20230106_095742 121_0403 iPhone 12.JPG", path "D:/Library/Mobile Repository/Sam Mobile/Albums/2023/01 January/iPhone 12/20230106_095748 091_1609 iPhone 12.JPG", path "D:/Library/Mobile Repository/Sam Mobile/Albums/2023/01 January/iPhone 12/20230106_095748 121_0403 iPhone 12.JPG", path "D:/Library/Mobile Repository/Sam Mobile/Albums/2023/01 January/iPhone 12/20230106_122032 091_1609 iPhone 12.JPG", path "D:/Library/Mobile Repository/Sam Mobile/Albums/2023/01 January/iPhone 12/20230106_122032 121_0403 iPhone 12.JPG", path "D:/Library/Mobile Repository/Sam Mobile/Albums/2023/01 January/iPhone 12/20230106_122133 091_1609 iPhone 12.JPG", path "D:/Library/Mobile Repository/Sam Mobile/Albums/2023/01 January/iPhone 12/20230106_122133 121_0403 iPhone 12.JPG", path "D:/Library/Mobile Repository/Sam Mobile/Albums/2023/01 January/iPhone 12/20230106_135548 091_1609 iPhone 12.JPG", path "D:/Library/Mobile Repository/Sam Mobile/Albums/2023/01 January/iPhone 12/20230106_135548 121_0403 iPhone 12.JPG", path "D:/Library/Mobile Repository/Sam Mobile/Albums/2023/01 January/iPhone 12/20230106_135945 091_1609 iPhone 12.JPG", path "D:/Library/Mobile Repository/Sam Mobile/Albums/2023/01 January/iPhone 12/20230106_135945 121_0403 iPhone 12.JPG", path "D:/Library/Mobile Repository/Sam Mobile/Albums/2023/01 January/iPhone 12/20230106_140003 091_1609 iPhone 12.JPG", path "D:/Library/Mobile Repository/Sam Mobile/Albums/2023/01 January/iPhone 12/20230106_140003 121_0403 iPhone 12.JPG", path "D:/Library/Mobile Repository/Sam Mobile/Albums/2023/01 January/iPhone 12/20230106_140006 091_1609 iPhone 12.JPG", path "D:/Library/Mobile Repository/Sam Mobile/Albums/2023/01 January/iPhone 12/20230106_140006 121_0403 iPhone 12.JPG", path "D:/Library/Mobile Repository/Sam Mobile/Albums/2023/01 January/iPhone 12/20230106_144620 091_1609 iPhone 12.JPG", path "D:/Library/Mobile Repository/Sam Mobile/Albums/2023/01 January/iPhone 12/20230106_144620 121_0403 iPhone 12.JPG", path "D:/Library/Mobile Repository/Sam Mobile/Albums/2023/01 January/iPhone 12/20230106_144625 091_1609 iPhone 12.JPG", path "D:/Library/Mobile Repository/Sam Mobile/Albums/2023/01 January/iPhone 12/20230106_144625 121_0403 iPhone 12.JPG", path "D:/Library/Mobile Repository/Sam Mobile/Albums/2023/01 January/iPhone 12/20230106_144700 091_1609 iPhone 12.JPG", path "D:/Library/Mobile Repository/Sam Mobile/Albums/2023/01 January/iPhone 12/20230106_144700 121_0403 iPhone 12.JPG", path "D:/Library/Mobile Repository/Sam Mobile/Albums/2023/01 January/iPhone 12/20230106_144702 091_1609 iPhone 12.JPG", path "D:/Library/Mobile Repository/Sam Mobile/Albums/2023/01 January/iPhone 12/20230106_144702 121_0403 iPhone 12.JPG", path "D:/Library/Mobile Repository/Sam Mobile/Albums/2023/01 January/iPhone 12/20230106_144720 091_1609 iPhone 12.JPG", path "D:/Library/Mobile Repository/Sam Mobile/Albums/2023/01 January/iPhone 12/20230106_144720 121_0403 iPhone 12.JPG", path "D:/Library/Mobile Repository/Sam Mobile/Albums/2023/01 January/iPhone 12/20230106_144737 091_1609 iPhone 12.JPG", path "D:/Library/Mobile Repository/Sam Mobile/Albums/2023/01 January/iPhone 12/20230106_144737 121_0403 iPhone 12.JPG", path "D:/Library/Mobile Repository/Sam Mobile/Albums/2023/01 January/iPhone 12/20230106_144744 091_0916 iPhone 12.JPG", path "D:/Library/Mobile Repository/Sam Mobile/Albums/2023/01 January/iPhone 12/20230106_144744 121_0304 iPhone 12.JPG", path "D:/Library/Mobile Repository/Sam Mobile/Albums/2023/01 January/iPhone 12/20230106_144755 091_1609 iPhone 12.JPG", path "D:/Library/Mobile Repository/Sam Mobile/Albums/2023/01 January/iPhone 12/20230106_144755 121_0403 iPhone 12.JPG", path "D:/Library/Mobile Repository/Sam Mobile/Albums/2023/01 January/iPhone 12/20230106_165140 091_1609 iPhone 12.JPG", path "D:/Library/Mobile Repository/Sam Mobile/Albums/2023/01 January/iPhone 12/20230106_165140 121_0403 iPhone 12.JPG", path "D:/Library/Mobile Repository/Sam Mobile/Albums/2023/01 January/iPhone 12/20230106_165144 091_1609 iPhone 12.JPG", path "D:/Library/Mobile Repository/Sam Mobile/Albums/2023/01 January/iPhone 12/20230106_165144 121_0403 iPhone 12.JPG", path "D:/Library/Mobile Repository/Sam Mobile/Albums/2023/01 January/iPhone 12/20230106_170121 091_1609 iPhone 12.JPG", path "D:/Library/Mobile Repository/Sam Mobile/Albums/2023/01 January/iPhone 12/20230106_170121 121_0403 iPhone 12.JPG", path "D:/Library/Mobile Repository/Sam Mobile/Albums/2023/01 January/iPhone 12/20230106_170141 091_1609 iPhone 12.JPG", path "D:/Library/Mobile Repository/Sam Mobile/Albums/2023/01 January/iPhone 12/20230106_170141 121_0403 iPhone 12.JPG", path "D:/Library/Mobile Repository/Sam Mobile/Albums/2023/01 January/iPhone 12/20230106_170219 091_1609 iPhone 12.JPG", path "D:/Library/Mobile Repository/Sam Mobile/Albums/2023/01 January/iPhone 12/20230106_170219 121_0403 iPhone 12.JPG", path "D:/Library/Mobile Repository/Sam Mobile/Albums/2023/01 January/iPhone 12/20230106_170721 091_1609 iPhone 12.JPG", path "D:/Library/Mobile Repository/Sam Mobile/Albums/2023/01 January/iPhone 12/20230106_170721 121_0403 iPhone 12.JPG", path "D:/Library/Mobile Repository/Sam Mobile/Albums/2023/01 January/iPhone 12/20230106_170729 091_1609 iPhone 12.JPG", path "D:/Library/Mobile Repository/Sam Mobile/Albums/2023/01 January/iPhone 12/20230106_170729 121_0403 iPhone 12.JPG", path "D:/Library/Mobile Repository/Sam Mobile/Albums/2023/01 January/iPhone 12/20230106_174004 091_1609 iPhone 12.JPG", path "D:/Library/Mobile Repository/Sam Mobile/Albums/2023/01 January/iPhone 12/20230106_174004 121_0403 iPhone 12.JPG", path "D:/Library/Mobile Repository/Sam Mobile/Albums/2023/01 January/iPhone 12/20230106_174007 091_1609 iPhone 12.JPG", path "D:/Library/Mobile Repository/Sam Mobile/Albums/2023/01 January/iPhone 12/20230106_174007 121_0403 iPhone 12.JPG", path "D:/Library/Mobile Repository/Sam Mobile/Albums/2023/01 January/iPhone 12/20230106_174015 091_1609 iPhone 12.JPG", path "D:/Library/Mobile Repository/Sam Mobile/Albums/2023/01 January/iPhone 12/20230106_174015 121_0403 iPhone 12.JPG", path "D:/Library/Mobile Repository/Sam Mobile/Albums/2023/01 January/iPhone 12/20230106_174750 091_1609 iPhone 12.JPG", path "D:/Library/Mobile Repository/Sam Mobile/Albums/2023/01 January/iPhone 12/20230106_174750 121_0403 iPhone 12.JPG", path "D:/Library/Mobile Repository/Sam Mobile/Albums/2023/01 January/iPhone 12/20230106_174755 091_1609 iPhone 12.JPG", path "D:/Library/Mobile Repository/Sam Mobile/Albums/2023/01 January/iPhone 12/20230106_174755 121_0403 iPhone 12.JPG", path "D:/Library/Mobile Repository/Sam Mobile/Albums/2023/01 January/iPhone 12/20230107_115722 091_1609 iPhone 12.JPG", path "D:/Library/Mobile Repository/Sam Mobile/Albums/2023/01 January/iPhone 12/20230107_115722 121_0403 iPhone 12.JPG", path "D:/Library/Mobile Repository/Sam Mobile/Albums/2023/01 January/iPhone 12/20230107_123636 091_1609 iPhone 12.JPG", path "D:/Library/Mobile Repository/Sam Mobile/Albums/2023/01 January/iPhone 12/20230107_123636 121_0403 iPhone 12.JPG", path "D:/Library/Mobile Repository/Sam Mobile/Albums/2023/01 January/iPhone 12/20230107_151239 091_1609 iPhone 12.JPG", path "D:/Library/Mobile Repository/Sam Mobile/Albums/2023/01 January/iPhone 12/20230107_151239 121_0403 iPhone 12.JPG", path "D:/Library/Mobile Repository/Sam Mobile/Albums/2023/01 January/iPhone 12/20230107_151245 091_1609 iPhone 12.JPG", path "D:/Library/Mobile Repository/Sam Mobile/Albums/2023/01 January/iPhone 12/20230107_151245 121_0403 iPhone 12.JPG", path "D:/Library/Mobile Repository/Sam Mobile/Albums/2023/01 January/iPhone 12/20230108_000938 021_0000 iPhone 12.JPG", path "D:/Library/Mobile Repository/Sam Mobile/Albums/2023/01 January/iPhone 12/20230108_000938 023_0000 iPhone 12.JPG", path "D:/Library/Mobile Repository/Sam Mobile/Albums/2023/01 January/iPhone 12/20230108_000938 121_0304 iPhone 12.JPG", path "D:/Library/Mobile Repository/Sam Mobile/Albums/2023/01 January/iPhone 12/20230108_000938 121_0403 iPhone 12.JPG", path "D:/Library/Mobile Repository/Sam Mobile/Albums/2023/01 January/iPhone 12/20230108_093847 121_0304 iPhone 12.JPG", path "D:/Library/Mobile Repository/Sam Mobile/Albums/2023/01 January/iPhone 12/20230108_093847 121_0403 iPhone 12.JPG", path "D:/Library/Mobile Repository/Sam Mobile/Albums/2023/01 January/iPhone 12/20230108_203021 091_1609 iPhone 12.JPG", path "D:/Library/Mobile Repository/Sam Mobile/Albums/2023/01 January/iPhone 12/20230108_203021 121_0403 iPhone 12.JPG", path "D:/Library/Mobile Repository/Sam Mobile/Albums/2023/01 January/iPhone 12/20230109_110354 121_0304 iPhone 12.JPG", path "D:/Library/Mobile Repository/Sam Mobile/Albums/2023/01 January/iPhone 12/20230109_110354 121_0403 iPhone 12.JPG", path "D:/Library/Mobile Repository/Sam Mobile/Albums/2023/01 January/iPhone 12/20230109_183016 121_0304 iPhone 12.JPG", path "D:/Library/Mobile Repository/Sam Mobile/Albums/2023/01 January/iPhone 12/20230109_183016 121_0403 iPhone 12.JPG", path "D:/Library/Mobile Repository/Sam Mobile/Albums/2023/01 January/iPhone 12/20230114_193305 121_0304 iPhone 12.JPG", path "D:/Library/Mobile Repository/Sam Mobile/Albums/2023/01 January/iPhone 12/20230114_193305 121_0403 iPhone 12.JPG", path "D:/Library/Mobile Repository/Sam Mobile/Albums/2023/01 January/iPhone 12/20230115_091333 091_1609 iPhone 12.JPG", path "D:/Library/Mobile Repository/Sam Mobile/Albums/2023/01 January/iPhone 12/20230115_091333 121_0403 iPhone 12.JPG", path "D:/Library/Mobile Repository/Sam Mobile/Albums/2023/01 January/iPhone 12/20230115_091339 091_1609 iPhone 12.JPG", path "D:/Library/Mobile Repository/Sam Mobile/Albums/2023/01 January/iPhone 12/20230115_091339 121_0403 iPhone 12.JPG", path "D:/Library/Mobile Repository/Sam Mobile/Albums/2023/01 January/iPhone 12/20230115_091539 091_1609 iPhone 12.JPG", path "D:/Library/Mobile Repository/Sam Mobile/Albums/2023/01 January/iPhone 12/20230115_091539 121_0403 iPhone 12.JPG", path "D:/Library/Mobile Repository/Sam Mobile/Albums/2023/01 January/iPhone 12/20230115_091541 091_1609 iPhone 12.JPG", path "D:/Library/Mobile Repository/Sam Mobile/Albums/2023/01 January/iPhone 12/20230115_091541 121_0403 iPhone 12.JPG", path "D:/Library/Mobile Repository/Sam Mobile/Albums/2023/01 January/iPhone 12/20230115_092959 091_1609 iPhone 12.JPG", path "D:/Library/Mobile Repository/Sam Mobile/Albums/2023/01 January/iPhone 12/20230115_092959 121_0403 iPhone 12.JPG", path "D:/Library/Mobile Repository/Sam Mobile/Albums/2023/01 January/iPhone 12/20230115_100732 091_1609 iPhone 12.JPG", path "D:/Library/Mobile Repository/Sam Mobile/Albums/2023/01 January/iPhone 12/20230115_100732 121_0403 iPhone 12.JPG", path "D:/Library/Mobile Repository/Sam Mobile/Albums/2023/01 January/iPhone 12/20230115_123111 091_1609 iPhone 12.JPG", path "D:/Library/Mobile Repository/Sam Mobile/Albums/2023/01 January/iPhone 12/20230115_123111 121_0403 iPhone 12.JPG", path "D:/Library/Mobile Repository/Sam Mobile/Albums/2023/01 January/iPhone 12/20230115_155446 091_1609 iPhone 12.JPG", path "D:/Library/Mobile Repository/Sam Mobile/Albums/2023/01 January/iPhone 12/20230115_155446 121_0403 iPhone 12.JPG", path "D:/Library/Mobile Repository/Sam Mobile/Albums/2023/01 January/iPhone 12/20230115_155525 091_1609 iPhone 12.JPG", path "D:/Library/Mobile Repository/Sam Mobile/Albums/2023/01 January/iPhone 12/20230115_155525 121_0403 iPhone 12.JPG", path "D:/Library/Mobile Repository/Sam Mobile/Albums/2023/01 January/iPhone 12/20230115_155536 091_1609 iPhone 12.JPG", path "D:/Library/Mobile Repository/Sam Mobile/Albums/2023/01 January/iPhone 12/20230115_155536 121_0403 iPhone 12.JPG", path "D:/Library/Mobile Repository/Sam Mobile/Albums/2023/01 January/iPhone 12/20230115_155548 091_1609 iPhone 12.JPG", path "D:/Library/Mobile Repository/Sam Mobile/Albums/2023/01 January/iPhone 12/20230115_155548 121_0403 iPhone 12.JPG", path "D:/Library/Mobile Repository/Sam Mobile/Albums/2023/01 January/iPhone 12/20230115_155621 091_1609 iPhone 12.JPG", path "D:/Library/Mobile Repository/Sam Mobile/Albums/2023/01 January/iPhone 12/20230115_155621 121_0403 iPhone 12.JPG", path "D:/Library/Mobile Repository/Sam Mobile/Albums/2023/01 January/iPhone 12/20230115_161014 091_1609 iPhone 12.JPG", path "D:/Library/Mobile Repository/Sam Mobile/Albums/2023/01 January/iPhone 12/20230115_161014 121_0403 iPhone 12.JPG", path "D:/Library/Mobile Repository/Sam Mobile/Albums/2023/01 January/iPhone 12/20230115_161015 091_1609 iPhone 12.JPG", path "D:/Library/Mobile Repository/Sam Mobile/Albums/2023/01 January/iPhone 12/20230115_161015 121_0403 iPhone 12.JPG", path "D:/Library/Mobile Repository/Sam Mobile/Albums/2023/01 January/iPhone 12/20230115_161239 091_1609 iPhone 12.JPG", path "D:/Library/Mobile Repository/Sam Mobile/Albums/2023/01 January/iPhone 12/20230115_161239 121_0403 iPhone 12.JPG", path "D:/Library/Mobile Repository/Sam Mobile/Albums/2023/01 January/iPhone 12/20230115_161418 091_1609 iPhone 12.JPG", path "D:/Library/Mobile Repository/Sam Mobile/Albums/2023/01 January/iPhone 12/20230115_161418 121_0403 iPhone 12.JPG", path "D:/Library/Mobile Repository/Sam Mobile/Albums/2023/01 January/iPhone 12/20230115_161536 091_1609 iPhone 12.JPG", path "D:/Library/Mobile Repository/Sam Mobile/Albums/2023/01 January/iPhone 12/20230115_161536 121_0403 iPhone 12.JPG", path "D:/Library/Mobile Repository/Sam Mobile/Albums/2023/01 January/iPhone 12/20230115_161629 091_1609 iPhone 12.JPG", path "D:/Library/Mobile Repository/Sam Mobile/Albums/2023/01 January/iPhone 12/20230115_161629 121_0403 iPhone 12.JPG", path "D:/Library/Mobile Repository/Sam Mobile/Albums/2023/01 January/iPhone 12/20230115_161643 091_1609 iPhone 12.JPG", path "D:/Library/Mobile Repository/Sam Mobile/Albums/2023/01 January/iPhone 12/20230115_161643 121_0403 iPhone 12.JPG", path "D:/Library/Mobile Repository/Sam Mobile/Albums/2023/01 January/iPhone 12/20230115_162127 091_1609 iPhone 12.JPG", path "D:/Library/Mobile Repository/Sam Mobile/Albums/2023/01 January/iPhone 12/20230115_162127 121_0403 iPhone 12.JPG", path "D:/Library/Mobile Repository/Sam Mobile/Albums/2023/01 January/iPhone 12/20230115_162130 091_1609 iPhone 12.JPG", path "D:/Library/Mobile Repository/Sam Mobile/Albums/2023/01 January/iPhone 12/20230115_162130 121_0403 iPhone 12.JPG", path "D:/Library/Mobile Repository/Sam Mobile/Albums/2023/01 January/iPhone 12/20230115_163047 091_1609 iPhone 12.JPG", path "D:/Library/Mobile Repository/Sam Mobile/Albums/2023/01 January/iPhone 12/20230115_163047 121_0403 iPhone 12.JPG", path "D:/Library/Mobile Repository/Sam Mobile/Albums/2023/01 January/iPhone 12/20230115_163435 091_0916 iPhone 12.JPG", path "D:/Library/Mobile Repository/Sam Mobile/Albums/2023/01 January/iPhone 12/20230115_163435 121_0304 iPhone 12.JPG", path "D:/Library/Mobile Repository/Sam Mobile/Albums/2023/01 January/iPhone 12/20230115_163642 091_1609 iPhone 12.JPG", path "D:/Library/Mobile Repository/Sam Mobile/Albums/2023/01 January/iPhone 12/20230115_163642 121_0403 iPhone 12.JPG", path "D:/Library/Mobile Repository/Sam Mobile/Albums/2023/01 January/iPhone 12/20230115_163711 091_1609 iPhone 12.JPG", path "D:/Library/Mobile Repository/Sam Mobile/Albums/2023/01 January/iPhone 12/20230115_163711 121_0403 iPhone 12.JPG", path "D:/Library/Mobile Repository/Sam Mobile/Albums/2023/01 January/iPhone 12/20230115_163830 091_1609 iPhone 12.JPG", path "D:/Library/Mobile Repository/Sam Mobile/Albums/2023/01 January/iPhone 12/20230115_163830 121_0403 iPhone 12.JPG", path "D:/Library/Mobile Repository/Sam Mobile/Albums/2023/01 January/iPhone 12/20230115_163955 091_1609 iPhone 12.JPG", path "D:/Library/Mobile Repository/Sam Mobile/Albums/2023/01 January/iPhone 12/20230115_163955 121_0403 iPhone 12.JPG", path "D:/Library/Mobile Repository/Sam Mobile/Albums/2023/01 January/iPhone 12/20230115_182848 091_1609 iPhone 12.JPG", path "D:/Library/Mobile Repository/Sam Mobile/Albums/2023/01 January/iPhone 12/20230115_182848 121_0403 iPhone 12.JPG", path "D:/Library/Mobile Repository/Sam Mobile/Albums/2023/01 January/iPhone 12/20230115_183054 091_1609 iPhone 12.JPG", path "D:/Library/Mobile Repository/Sam Mobile/Albums/2023/01 January/iPhone 12/20230115_183054 121_0403 iPhone 12.JPG", path "D:/Library/Mobile Repository/Sam Mobile/Albums/2023/01 January/iPhone 12/20230115_183255 091_1609 iPhone 12.JPG", path "D:/Library/Mobile Repository/Sam Mobile/Albums/2023/01 January/iPhone 12/20230115_183255 121_0403 iPhone 12.JPG", path "D:/Library/Mobile Repository/Sam Mobile/Albums/2023/01 January/iPhone 12/20230115_183311 091_1609 iPhone 12.JPG", path "D:/Library/Mobile Repository/Sam Mobile/Albums/2023/01 January/iPhone 12/20230115_183311 121_0403 iPhone 12.JPG", path "D:/Library/Mobile Repository/Sam Mobile/Albums/2023/01 January/iPhone 12/20230115_183314 091_1609 iPhone 12.JPG", path "D:/Library/Mobile Repository/Sam Mobile/Albums/2023/01 January/iPhone 12/20230115_183314 121_0403 iPhone 12.JPG", path "D:/Library/Mobile Repository/Sam Mobile/Albums/2023/01 January/iPhone 12/20230115_183342 091_1609 iPhone 12.JPG", path "D:/Library/Mobile Repository/Sam Mobile/Albums/2023/01 January/iPhone 12/20230115_183342 121_0403 iPhone 12.JPG", path "D:/Library/Mobile Repository/Sam Mobile/Albums/2023/01 January/iPhone 12/20230115_183351 091_1609 iPhone 12.JPG", path "D:/Library/Mobile Repository/Sam Mobile/Albums/2023/01 January/iPhone 12/20230115_183351 121_0403 iPhone 12.JPG", path "D:/Library/Mobile Repository/Sam Mobile/Albums/2023/01 January/iPhone 12/20230115_183419 091_1609 iPhone 12.JPG", path "D:/Library/Mobile Repository/Sam Mobile/Albums/2023/01 January/iPhone 12/20230115_183419 121_0403 iPhone 12.JPG", path "D:/Library/Mobile Repository/Sam Mobile/Albums/2023/01 January/iPhone 12/20230115_183431 091_1609 iPhone 12.JPG", path "D:/Library/Mobile Repository/Sam Mobile/Albums/2023/01 January/iPhone 12/20230115_183431 121_0403 iPhone 12.JPG", path "D:/Library/Mobile Repository/Sam Mobile/Albums/2023/01 January/iPhone 12/20230115_183728 091_1609 iPhone 12.JPG", path "D:/Library/Mobile Repository/Sam Mobile/Albums/2023/01 January/iPhone 12/20230115_183728 121_0403 iPhone 12.JPG", path "D:/Library/Mobile Repository/Sam Mobile/Albums/2023/01 January/iPhone 12/20230115_185452 091_1609 iPhone 12.JPG", path "D:/Library/Mobile Repository/Sam Mobile/Albums/2023/01 January/iPhone 12/20230115_185452 121_0403 iPhone 12.JPG", path "D:/Library/Mobile Repository/Sam Mobile/Albums/2023/01 January/iPhone 12/20230115_185512 091_1609 iPhone 12.JPG", path "D:/Library/Mobile Repository/Sam Mobile/Albums/2023/01 January/iPhone 12/20230115_185512 121_0403 iPhone 12.JPG", path "D:/Library/Mobile Repository/Sam Mobile/Albums/2023/01 January/iPhone 12/20230116_083431 091_1609 iPhone 12.JPG", path "D:/Library/Mobile Repository/Sam Mobile/Albums/2023/01 January/iPhone 12/20230116_083431 121_0403 iPhone 12.JPG", path "D:/Library/Mobile Repository/Sam Mobile/Albums/2023/01 January/iPhone 12/20230116_083433 091_1609 iPhone 12.JPG", path "D:/Library/Mobile Repository/Sam Mobile/Albums/2023/01 January/iPhone 12/20230116_083433 121_0403 iPhone 12.JPG", path "D:/Library/Mobile Repository/Sam Mobile/Albums/2023/01 January/iPhone 12/20230116_083544 091_1609 iPhone 12.JPG", path "D:/Library/Mobile Repository/Sam Mobile/Albums/2023/01 January/iPhone 12/20230116_083544 121_0403 iPhone 12.JPG", path "D:/Library/Mobile Repository/Sam Mobile/Albums/2023/01 January/iPhone 12/20230116_083639 091_1609 iPhone 12.JPG", path "D:/Library/Mobile Repository/Sam Mobile/Albums/2023/01 January/iPhone 12/20230116_083639 121_0403 iPhone 12.JPG", path "D:/Library/Mobile Repository/Sam Mobile/Albums/2023/01 January/iPhone 12/20230116_090816 091_1609 iPhone 12.JPG", path "D:/Library/Mobile Repository/Sam Mobile/Albums/2023/01 January/iPhone 12/20230116_090816 121_0403 iPhone 12.JPG", path "D:/Library/Mobile Repository/Sam Mobile/Albums/2023/01 January/iPhone 12/20230116_090820 091_1609 iPhone 12.JPG", path "D:/Library/Mobile Repository/Sam Mobile/Albums/2023/01 January/iPhone 12/20230116_090820 121_0403 iPhone 12.JPG", path "D:/Library/Mobile Repository/Sam Mobile/Albums/2023/01 January/iPhone 12/20230116_092045 091_1609 iPhone 12.JPG", path "D:/Library/Mobile Repository/Sam Mobile/Albums/2023/01 January/iPhone 12/20230116_092045 121_0403 iPhone 12.JPG", path "D:/Library/Mobile Repository/Sam Mobile/Albums/2023/01 January/iPhone 12/20230116_092203 091_1609 iPhone 12.JPG", path "D:/Library/Mobile Repository/Sam Mobile/Albums/2023/01 January/iPhone 12/20230116_092203 121_0403 iPhone 12.JPG", path "D:/Library/Mobile Repository/Sam Mobile/Albums/2023/01 January/iPhone 12/20230116_092232 091_1609 iPhone 12.JPG", path "D:/Library/Mobile Repository/Sam Mobile/Albums/2023/01 January/iPhone 12/20230116_092232 121_0403 iPhone 12.JPG", path "D:/Library/Mobile Repository/Sam Mobile/Albums/2023/01 January/iPhone 12/20230116_092237 091_1609 iPhone 12.JPG", path "D:/Library/Mobile Repository/Sam Mobile/Albums/2023/01 January/iPhone 12/20230116_092237 121_0403 iPhone 12.JPG", path "D:/Library/Mobile Repository/Sam Mobile/Albums/2023/01 January/iPhone 12/20230116_092311 091_1609 iPhone 12.JPG", path "D:/Library/Mobile Repository/Sam Mobile/Albums/2023/01 January/iPhone 12/20230116_092311 121_0403 iPhone 12.JPG", path "D:/Library/Mobile Repository/Sam Mobile/Albums/2023/01 January/iPhone 12/20230116_092312 091_1609 iPhone 12.jpg", path "D:/Library/Mobile Repository/Sam Mobile/Albums/2023/01 January/iPhone 12/20230116_092312 121_0403 iPhone 12.JPG", path "D:/Library/Mobile Repository/Sam Mobile/Albums/2023/01 January/iPhone 12/20230116_092405 091_1609 iPhone 12.JPG", path "D:/Library/Mobile Repository/Sam Mobile/Albums/2023/01 January/iPhone 12/20230116_092405 121_0403 iPhone 12.jpg", path "D:/Library/Mobile Repository/Sam Mobile/Albums/2023/01 January/iPhone 12/20230116_092525 091_1609 iPhone 12.JPG", path "D:/Library/Mobile Repository/Sam Mobile/Albums/2023/01 January/iPhone 12/20230116_092525 121_0403 iPhone 12.JPG", path "D:/Library/Mobile Repository/Sam Mobile/Albums/2023/01 January/iPhone 12/20230116_092849 091_1609 iPhone 12.JPG", path "D:/Library/Mobile Repository/Sam Mobile/Albums/2023/01 January/iPhone 12/20230116_092849 121_0403 iPhone 12.JPG", path "D:/Library/Mobile Repository/Sam Mobile/Albums/2023/01 January/iPhone 12/20230116_092900 091_1609 iPhone 12.JPG", path "D:/Library/Mobile Repository/Sam Mobile/Albums/2023/01 January/iPhone 12/20230116_092900 121_0403 iPhone 12.JPG", path "D:/Library/Mobile Repository/Sam Mobile/Albums/2023/01 January/iPhone 12/20230116_095639 091_1609 iPhone 12.JPG", path "D:/Library/Mobile Repository/Sam Mobile/Albums/2023/01 January/iPhone 12/20230116_095639 121_0403 iPhone 12.JPG", path "D:/Library/Mobile Repository/Sam Mobile/Albums/2023/01 January/iPhone 12/20230116_095643 091_1609 iPhone 12.JPG", path "D:/Library/Mobile Repository/Sam Mobile/Albums/2023/01 January/iPhone 12/20230116_095643 121_0403 iPhone 12.JPG", path "D:/Library/Mobile Repository/Sam Mobile/Albums/2023/01 January/iPhone 12/20230116_100431 091_1609 iPhone 12.JPG", path "D:/Library/Mobile Repository/Sam Mobile/Albums/2023/01 January/iPhone 12/20230116_100431 121_0403 iPhone 12.JPG", path "D:/Library/Mobile Repository/Sam Mobile/Albums/2023/01 January/iPhone 12/20230116_101256 091_0916 iPhone 12.JPG", path "D:/Library/Mobile Repository/Sam Mobile/Albums/2023/01 January/iPhone 12/20230116_101256 121_0304 iPhone 12.JPG", path "D:/Library/Mobile Repository/Sam Mobile/Albums/2023/01 January/iPhone 12/20230116_101303 091_1609 iPhone 12.JPG", path "D:/Library/Mobile Repository/Sam Mobile/Albums/2023/01 January/iPhone 12/20230116_101303 121_0403 iPhone 12.JPG", path "D:/Library/Mobile Repository/Sam Mobile/Albums/2023/01 January/iPhone 12/20230116_101359 091_1609 iPhone 12.JPG", path "D:/Library/Mobile Repository/Sam Mobile/Albums/2023/01 January/iPhone 12/20230116_101359 121_0403 iPhone 12.JPG", path "D:/Library/Mobile Repository/Sam Mobile/Albums/2023/01 January/iPhone 12/20230116_110813 091_1609 iPhone 12.JPG", path "D:/Library/Mobile Repository/Sam Mobile/Albums/2023/01 January/iPhone 12/20230116_110813 121_0403 iPhone 12.JPG", path "D:/Library/Mobile Repository/Sam Mobile/Albums/2023/01 January/iPhone 12/20230116_110816 091_1609 iPhone 12.JPG", path "D:/Library/Mobile Repository/Sam Mobile/Albums/2023/01 January/iPhone 12/20230116_110816 121_0403 iPhone 12.JPG", path "D:/Library/Mobile Repository/Sam Mobile/Albums/2023/01 January/iPhone 12/20230122_071842 091_1609 iPhone 12.JPG", path "D:/Library/Mobile Repository/Sam Mobile/Albums/2023/01 January/iPhone 12/20230122_071842 121_0403 iPhone 12.JPG", path "D:/Library/Mobile Repository/Sam Mobile/Albums/2023/01 January/iPhone 12/20230124_130710 091_1609 iPhone 12.JPG", path "D:/Library/Mobile Repository/Sam Mobile/Albums/2023/01 January/iPhone 12/20230124_130710 121_0403 iPhone 12.JPG", path "D:/Library/Mobile Repository/Sam Mobile/Albums/2023/01 January/iPhone 12/20230124_130752 091_1609 iPhone 12.JPG", path "D:/Library/Mobile Repository/Sam Mobile/Albums/2023/01 January/iPhone 12/20230124_130752 121_0403 iPhone 12.JPG", path "D:/Library/Mobile Repository/Sam Mobile/Albums/2023/01 January/iPhone 12/20230124_132533 091_1609 iPhone 12.JPG", path "D:/Library/Mobile Repository/Sam Mobile/Albums/2023/01 January/iPhone 12/20230124_132533 121_0403 iPhone 12.JPG", path "D:/Library/Mobile Repository/Sam Mobile/Albums/2023/01 January/iPhone 12/20230130_103449 091_1609 iPhone 12.JPG", path "D:/Library/Mobile Repository/Sam Mobile/Albums/2023/01 January/iPhone 12/20230130_103449 121_0403 iPhone 12.JPG", path "D:/Library/Mobile Repository/Sam Mobile/Albums/2023/01 January/iPhone 12/20230130_103455 091_1609 iPhone 12.JPG", path "D:/Library/Mobile Repository/Sam Mobile/Albums/2023/01 January/iPhone 12/20230130_103455 121_0403 iPhone 12.JPG", path "D:/Library/Mobile Repository/Sam Mobile/Albums/2023/01 January/iPhone 12/20230130_171211 091_1609 iPhone 12.JPG", path "D:/Library/Mobile Repository/Sam Mobile/Albums/2023/01 January/iPhone 12/20230130_171211 121_0403 iPhone 12.JPG", path "D:/Library/Mobile Repository/Sam Mobile/Albums/2023/01 January/iPhone 12/20230130_171225 091_1609 iPhone 12.JPG", path "D:/Library/Mobile Repository/Sam Mobile/Albums/2023/01 January/iPhone 12/20230130_171225 121_0403 iPhone 12.JPG", path "D:/Library/Mobile Repository/Sam Mobile/Albums/2023/01 January/iPhone 12/20230131_085121 091_1609 iPhone 12.JPG", path "D:/Library/Mobile Repository/Sam Mobile/Albums/2023/01 January/iPhone 12/20230131_085121 121_0403 iPhone 12.JPG", path "D:/Library/Mobile Repository/Sam Mobile/Albums/2023/02 February/iPhone 12/20230207_160520 028_4225 iPhone 12.JPG", path "D:/Library/Mobile Repository/Sam Mobile/Albums/2023/02 February/iPhone 12/20230207_160520 121_0403 iPhone 12.JPG", path "D:/Library/Mobile Repository/Sam Mobile/Albums/2023/02 February/iPhone 12/20230214_113445 061_0304 iPhone 12.JPG", path "D:/Library/Mobile Repository/Sam Mobile/Albums/2023/02 February/iPhone 12/20230214_113445 121_0403 iPhone 12.JPG", path "D:/Library/Mobile Repository/Sam Mobile/Albums/2023/02 February/iPhone 12/20230214_113455 072_0000 iPhone 12.JPG", path "D:/Library/Mobile Repository/Sam Mobile/Albums/2023/02 February/iPhone 12/20230214_113455 121_0403 iPhone 12.JPG", path "D:/Library/Mobile Repository/Sam Mobile/Albums/2023/02 February/iPhone 12/20230218_122606 091_1609 iPhone 12.JPG", path "D:/Library/Mobile Repository/Sam Mobile/Albums/2023/02 February/iPhone 12/20230218_122606 121_0403 iPhone 12.JPG", path "D:/Library/Mobile Repository/Sam Mobile/Albums/2023/02 February/iPhone 12/20230218_122620 091_1609 iPhone 12.JPG", path "D:/Library/Mobile Repository/Sam Mobile/Albums/2023/02 February/iPhone 12/20230218_122620 121_0403 iPhone 12.JPG", path "D:/Library/Mobile Repository/Sam Mobile/Albums/2023/02 February/iPhone 12/20230223_130024 091_1609 iPhone 12.JPG", path "D:/Library/Mobile Repository/Sam Mobile/Albums/2023/02 February/iPhone 12/20230223_130024 121_0403 iPhone 12.JPG", path "D:/Library/Mobile Repository/Sam Mobile/Albums/2023/02 February/iPhone 12/20230224_183248 091_1609 iPhone 12.JPG", path "D:/Library/Mobile Repository/Sam Mobile/Albums/2023/02 February/iPhone 12/20230224_183248 121_0403 iPhone 12.JPG", path "D:/Library/Mobile Repository/Sam Mobile/Albums/2023/02 February/iPhone 12/20230225_112304 091_1609 iPhone 12.JPG", path "D:/Library/Mobile Repository/Sam Mobile/Albums/2023/02 February/iPhone 12/20230225_112304 121_0403 iPhone 12.JPG", path "D:/Library/Mobile Repository/Sam Mobile/Albums/2023/02 February/iPhone 12/20230225_112310 091_1609 iPhone 12.JPG", path "D:/Library/Mobile Repository/Sam Mobile/Albums/2023/02 February/iPhone 12/20230225_112310 121_0403 iPhone 12.JPG", path "D:/Library/Mobile Repository/Sam Mobile/Albums/2023/02 February/iPhone 12/20230225_112332 091_0916 iPhone 12.JPG", path "D:/Library/Mobile Repository/Sam Mobile/Albums/2023/02 February/iPhone 12/20230225_112332 121_0403 iPhone 12.JPG", path "D:/Library/Mobile Repository/Sam Mobile/Albums/2023/02 February/iPhone 12/20230225_112721 091_1609 iPhone 12.JPG", path "D:/Library/Mobile Repository/Sam Mobile/Albums/2023/02 February/iPhone 12/20230225_112721 121_0403 iPhone 12.JPG", path "D:/Library/Mobile Repository/Sam Mobile/Albums/2023/02 February/iPhone 12/20230225_115937 091_1609 iPhone 12.JPG", path "D:/Library/Mobile Repository/Sam Mobile/Albums/2023/02 February/iPhone 12/20230225_115937 121_0403 iPhone 12.JPG", path "D:/Library/Mobile Repository/Sam Mobile/Albums/2023/02 February/iPhone 12/20230225_120229 091_1609 iPhone 12.JPG", path "D:/Library/Mobile Repository/Sam Mobile/Albums/2023/02 February/iPhone 12/20230225_120229 121_0403 iPhone 12.JPG", path "D:/Library/Mobile Repository/Sam Mobile/Albums/2023/02 February/iPhone 12/20230225_120231 091_1609 iPhone 12.JPG", path "D:/Library/Mobile Repository/Sam Mobile/Albums/2023/02 February/iPhone 12/20230225_120231 121_0403 iPhone 12.JPG", path "D:/Library/Mobile Repository/Sam Mobile/Albums/2023/02 February/iPhone 12/20230225_120232 091_1609 iPhone 12.JPG", path "D:/Library/Mobile Repository/Sam Mobile/Albums/2023/02 February/iPhone 12/20230225_120232 121_0403 iPhone 12.JPG", path "D:/Library/Mobile Repository/Sam Mobile/Albums/2023/02 February/iPhone 12/20230225_122556 091_1609 iPhone 12.JPG", path "D:/Library/Mobile Repository/Sam Mobile/Albums/2023/02 February/iPhone 12/20230225_122556 121_0403 iPhone 12.JPG", path "D:/Library/Mobile Repository/Sam Mobile/Albums/2023/02 February/iPhone 12/20230225_122602 091_1609 iPhone 12.JPG", path "D:/Library/Mobile Repository/Sam Mobile/Albums/2023/02 February/iPhone 12/20230225_122602 121_0403 iPhone 12.JPG", path "D:/Library/Mobile Repository/Sam Mobile/Albums/2023/02 February/iPhone 12/20230227_180130 091_1609 iPhone 12.JPG", path "D:/Library/Mobile Repository/Sam Mobile/Albums/2023/02 February/iPhone 12/20230227_180130 121_0403 iPhone 12.JPG", path "D:/Library/Mobile Repository/Sam Mobile/Albums/2023/03 March/iPhone 12/20230301_204717 091_0000 iPhone 12.JPG", path "D:/Library/Mobile Repository/Sam Mobile/Albums/2023/03 March/iPhone 12/20230301_204717 121_0403 iPhone 12.JPG", path "D:/Library/Mobile Repository/Sam Mobile/Albums/2023/03 March/iPhone 12/20230306_181651 091_1609 iPhone 12.JPG", path "D:/Library/Mobile Repository/Sam Mobile/Albums/2023/03 March/iPhone 12/20230306_181651 121_0403 iPhone 12.JPG", path "D:/Library/Mobile Repository/Sam Mobile/Albums/2023/03 March/iPhone 12/20230306_181658 091_1609 iPhone 12.JPG", path "D:/Library/Mobile Repository/Sam Mobile/Albums/2023/03 March/iPhone 12/20230306_181658 121_0403 iPhone 12.JPG", path "D:/Library/Mobile Repository/Sam Mobile/Albums/2023/03 March/iPhone 12/20230306_181903 091_1609 iPhone 12.JPG", path "D:/Library/Mobile Repository/Sam Mobile/Albums/2023/03 March/iPhone 12/20230306_181903 121_0403 iPhone 12.JPG", path "D:/Library/Mobile Repository/Sam Mobile/Albums/2023/03 March/iPhone 12/20230306_181915 091_1609 iPhone 12.JPG", path "D:/Library/Mobile Repository/Sam Mobile/Albums/2023/03 March/iPhone 12/20230306_181915 121_0403 iPhone 12.JPG", path "D:/Library/Mobile Repository/Sam Mobile/Albums/2023/03 March/iPhone 12/20230308_175214 091_1609 iPhone 12.JPG", path "D:/Library/Mobile Repository/Sam Mobile/Albums/2023/03 March/iPhone 12/20230308_175214 121_0403 iPhone 12.JPG", path "D:/Library/Mobile Repository/Sam Mobile/Albums/2023/03 March/iPhone 12/20230308_175231 091_1609 iPhone 12.JPG", path "D:/Library/Mobile Repository/Sam Mobile/Albums/2023/03 March/iPhone 12/20230308_175231 121_0403 iPhone 12.JPG", path "D:/Library/Mobile Repository/Sam Mobile/Albums/2023/03 March/iPhone 12/20230312_112246 091_1609 iPhone 12.JPG", path "D:/Library/Mobile Repository/Sam Mobile/Albums/2023/03 March/iPhone 12/20230312_112246 121_0403 iPhone 12.JPG", path "D:/Library/Mobile Repository/Sam Mobile/Albums/2023/03 March/iPhone 12/20230312_112319 091_1609 iPhone 12.JPG", path "D:/Library/Mobile Repository/Sam Mobile/Albums/2023/03 March/iPhone 12/20230312_112319 121_0403 iPhone 12.JPG", path "D:/Library/Mobile Repository/Sam Mobile/Albums/2023/03 March/iPhone 12/20230312_112337 091_1609 iPhone 12.JPG", path "D:/Library/Mobile Repository/Sam Mobile/Albums/2023/03 March/iPhone 12/20230312_112337 121_0403 iPhone 12.JPG", path "D:/Library/Mobile Repository/Sam Mobile/Albums/2023/03 March/iPhone 12/20230313_154445 091_1609 iPhone 12.JPG", path "D:/Library/Mobile Repository/Sam Mobile/Albums/2023/03 March/iPhone 12/20230313_154445 121_0403 iPhone 12.JPG", path "D:/Library/Mobile Repository/Sam Mobile/Albums/2023/03 March/iPhone 12/20230313_171759 091_1609 iPhone 12.JPG", path "D:/Library/Mobile Repository/Sam Mobile/Albums/2023/03 March/iPhone 12/20230313_171759 121_0403 iPhone 12.JPG", path "D:/Library/Mobile Repository/Sam Mobile/Albums/2023/03 March/iPhone 12/20230313_173436 091_1609 iPhone 12.JPG", path "D:/Library/Mobile Repository/Sam Mobile/Albums/2023/03 March/iPhone 12/20230313_173436 121_0403 iPhone 12.JPG", path "D:/Library/Mobile Repository/Sam Mobile/Albums/2023/03 March/iPhone 12/20230316_212021 027_0000 iPhone 12.JPG", path "D:/Library/Mobile Repository/Sam Mobile/Albums/2023/03 March/iPhone 12/20230316_212021 121_0403 iPhone 12.JPG", path "D:/Library/Mobile Repository/Sam Mobile/Albums/2023/03 March/iPhone 12/20230324_164841 091_1609 iPhone 12.JPG", path "D:/Library/Mobile Repository/Sam Mobile/Albums/2023/03 March/iPhone 12/20230324_164841 121_0403 iPhone 12.JPG", path "D:/Library/Mobile Repository/Sam Mobile/Albums/2023/03 March/iPhone 12/20230324_164846 091_1609 iPhone 12.JPG", path "D:/Library/Mobile Repository/Sam Mobile/Albums/2023/03 March/iPhone 12/20230324_164846 121_0403 iPhone 12.JPG", path "D:/Library/Mobile Repository/Sam Mobile/Albums/2023/03 March/iPhone 12/20230324_165019 091_1609 iPhone 12.JPG", path "D:/Library/Mobile Repository/Sam Mobile/Albums/2023/03 March/iPhone 12/20230324_165019 121_0403 iPhone 12.JPG", path "D:/Library/Mobile Repository/Sam Mobile/Albums/2023/03 March/iPhone 12/20230324_165025 091_1609 iPhone 12.JPG", path "D:/Library/Mobile Repository/Sam Mobile/Albums/2023/03 March/iPhone 12/20230324_165025 121_0403 iPhone 12.JPG", path "D:/Library/Mobile Repository/Sam Mobile/Albums/2023/03 March/iPhone 12/20230327_151518 091_1609 iPhone 12.JPG", path "D:/Library/Mobile Repository/Sam Mobile/Albums/2023/03 March/iPhone 12/20230327_151518 121_0403 iPhone 12.JPG", path "D:/Library/Mobile Repository/Sam Mobile/Albums/2023/03 March/iPhone 12/20230327_151528 091_1609 iPhone 12.JPG", path "D:/Library/Mobile Repository/Sam Mobile/Albums/2023/03 March/iPhone 12/20230327_151528 121_0403 iPhone 12.JPG", path "D:/Library/Mobile Repository/Sam Mobile/Albums/2023/03 March/iPhone 12/20230327_151607 091_1609 iPhone 12.JPG", path "D:/Library/Mobile Repository/Sam Mobile/Albums/2023/03 March/iPhone 12/20230327_151607 121_0403 iPhone 12.JPG", path "D:/Library/Mobile Repository/Sam Mobile/Albums/2023/03 March/iPhone 12/20230327_151611 091_1609 iPhone 12.JPG", path "D:/Library/Mobile Repository/Sam Mobile/Albums/2023/03 March/iPhone 12/20230327_151611 121_0403 iPhone 12.JPG", path "D:/Library/Mobile Repository/Sam Mobile/Albums/2023/03 March/iPhone 12/20230327_152453 091_1609 iPhone 12.JPG", path "D:/Library/Mobile Repository/Sam Mobile/Albums/2023/03 March/iPhone 12/20230327_152453 121_0403 iPhone 12.JPG", path "D:/Library/Mobile Repository/Sam Mobile/Albums/2023/03 March/iPhone 12/20230327_152647 091_1609 iPhone 12.JPG", path "D:/Library/Mobile Repository/Sam Mobile/Albums/2023/03 March/iPhone 12/20230327_152647 121_0403 iPhone 12.JPG", path "D:/Library/Mobile Repository/Sam Mobile/Albums/2023/03 March/iPhone 12/20230327_152653 091_1609 iPhone 12.JPG", path "D:/Library/Mobile Repository/Sam Mobile/Albums/2023/03 March/iPhone 12/20230327_152653 121_0403 iPhone 12.JPG", path "D:/Library/Mobile Repository/Sam Mobile/Albums/2023/03 March/iPhone 12/20230327_152713 091_1609 iPhone 12.JPG", path "D:/Library/Mobile Repository/Sam Mobile/Albums/2023/03 March/iPhone 12/20230327_152713 121_0403 iPhone 12.JPG", path "D:/Library/Mobile Repository/Sam Mobile/Albums/2023/03 March/iPhone 12/20230327_152850 091_1609 iPhone 12.JPG", path "D:/Library/Mobile Repository/Sam Mobile/Albums/2023/03 March/iPhone 12/20230327_152850 121_0403 iPhone 12.JPG", path "D:/Library/Mobile Repository/Sam Mobile/Albums/2023/04 April/iPhone 12/20230407_114030 091_1609 iPhone 12.JPG", path "D:/Library/Mobile Repository/Sam Mobile/Albums/2023/04 April/iPhone 12/20230407_114030 121_0403 iPhone 12.JPG", path "D:/Library/Mobile Repository/Sam Mobile/Albums/2023/04 April/iPhone 12/20230408_100435 091_1609 iPhone 12.JPG", path "D:/Library/Mobile Repository/Sam Mobile/Albums/2023/04 April/iPhone 12/20230408_100435 121_0403 iPhone 12.JPG", path "D:/Library/Mobile Repository/Sam Mobile/Albums/2023/04 April/iPhone 12/20230408_100448 091_1609 iPhone 12.JPG", path "D:/Library/Mobile Repository/Sam Mobile/Albums/2023/04 April/iPhone 12/20230408_100448 121_0403 iPhone 12.JPG", path "D:/Library/Mobile Repository/Sam Mobile/Albums/2023/04 April/iPhone 12/20230411_202239 091_1609 iPhone 12.JPG", path "D:/Library/Mobile Repository/Sam Mobile/Albums/2023/04 April/iPhone 12/20230411_202239 121_0403 iPhone 12.JPG", path "D:/Library/Mobile Repository/Sam Mobile/Albums/2023/04 April/iPhone 12/20230412_093101 069_0000 iPhone 12.JPG", path "D:/Library/Mobile Repository/Sam Mobile/Albums/2023/04 April/iPhone 12/20230412_093101 121_0403 iPhone 12.JPG", path "D:/Library/Mobile Repository/Sam Mobile/Albums/2023/04 April/iPhone 12/20230413_202133 065_0000 iPhone 12.JPG", path "D:/Library/Mobile Repository/Sam Mobile/Albums/2023/04 April/iPhone 12/20230413_202133 121_0403 iPhone 12.JPG", path "D:/Library/Mobile Repository/Sam Mobile/Albums/2023/04 April/iPhone 12/20230413_202145 046_0000 iPhone 12.JPG", path "D:/Library/Mobile Repository/Sam Mobile/Albums/2023/04 April/iPhone 12/20230413_202145 121_0403 iPhone 12.JPG", path "D:/Library/Mobile Repository/Sam Mobile/Albums/2023/04 April/iPhone 12/20230413_202155 061_0000 iPhone 12.JPG", path "D:/Library/Mobile Repository/Sam Mobile/Albums/2023/04 April/iPhone 12/20230413_202155 121_0403 iPhone 12.JPG", path "D:/Library/Mobile Repository/Sam Mobile/Albums/2023/04 April/iPhone 12/20230425_062706 091_1609 iPhone 12.JPG", path "D:/Library/Mobile Repository/Sam Mobile/Albums/2023/04 April/iPhone 12/20230425_062706 121_0403 iPhone 12.JPG", path "D:/Library/Mobile Repository/Sam Mobile/Albums/2023/04 April/iPhone 12/20230425_062710 091_1609 iPhone 12.JPG", path "D:/Library/Mobile Repository/Sam Mobile/Albums/2023/04 April/iPhone 12/20230425_062710 121_0403 iPhone 12.JPG", path "D:/Library/Mobile Repository/Sam Mobile/Albums/2023/04 April/iPhone 12/20230425_062712 091_1609 iPhone 12.JPG", path "D:/Library/Mobile Repository/Sam Mobile/Albums/2023/04 April/iPhone 12/20230425_062712 121_0403 iPhone 12.JPG", path "D:/Library/Mobile Repository/Sam Mobile/Albums/2023/04 April/iPhone 12/20230425_070302 091_1609 iPhone 12.JPG", path "D:/Library/Mobile Repository/Sam Mobile/Albums/2023/04 April/iPhone 12/20230425_070302 121_0403 iPhone 12.JPG", path "D:/Library/Mobile Repository/Sam Mobile/Albums/2023/04 April/iPhone 12/20230425_070306 091_1609 iPhone 12.JPG", path "D:/Library/Mobile Repository/Sam Mobile/Albums/2023/04 April/iPhone 12/20230425_070306 121_0403 iPhone 12.JPG", path "D:/Library/Mobile Repository/Sam Mobile/Albums/2023/04 April/iPhone 12/20230425_072917 091_1609 iPhone 12.JPG", path "D:/Library/Mobile Repository/Sam Mobile/Albums/2023/04 April/iPhone 12/20230425_072917 121_0403 iPhone 12.JPG", path "D:/Library/Mobile Repository/Sam Mobile/Albums/2023/04 April/iPhone 12/20230425_081846 091_1609 iPhone 12.JPG", path "D:/Library/Mobile Repository/Sam Mobile/Albums/2023/04 April/iPhone 12/20230425_081846 121_0403 iPhone 12.JPG", path "D:/Library/Mobile Repository/Sam Mobile/Albums/2023/04 April/iPhone 12/20230425_085915 091_1609 iPhone 12.JPG", path "D:/Library/Mobile Repository/Sam Mobile/Albums/2023/04 April/iPhone 12/20230425_085915 121_0403 iPhone 12.JPG", path "D:/Library/Mobile Repository/Sam Mobile/Albums/2023/04 April/iPhone 12/20230425_085919 091_1609 iPhone 12.JPG", path "D:/Library/Mobile Repository/Sam Mobile/Albums/2023/04 April/iPhone 12/20230425_085919 121_0403 iPhone 12.JPG", path "D:/Library/Mobile Repository/Sam Mobile/Albums/2023/04 April/iPhone 12/20230426_101137 091_1609 iPhone 12.JPG", path "D:/Library/Mobile Repository/Sam Mobile/Albums/2023/04 April/iPhone 12/20230426_101137 121_0403 iPhone 12.JPG", path "D:/Library/Mobile Repository/Sam Mobile/Albums/2023/04 April/iPhone 12/20230426_101141 091_1609 iPhone 12.JPG", path "D:/Library/Mobile Repository/Sam Mobile/Albums/2023/04 April/iPhone 12/20230426_101141 121_0403 iPhone 12.JPG", path "D:/Library/Mobile Repository/Sam Mobile/Albums/2023/04 April/iPhone 12/20230427_122334 091_1609 iPhone 12.JPG", path "D:/Library/Mobile Repository/Sam Mobile/Albums/2023/04 April/iPhone 12/20230427_122334 121_0403 iPhone 12.JPG", path "D:/Library/Mobile Repository/Sam Mobile/Albums/2023/04 April/iPhone 12/20230427_122349 091_1609 iPhone 12.JPG", path "D:/Library/Mobile Repository/Sam Mobile/Albums/2023/04 April/iPhone 12/20230427_122349 121_0403 iPhone 12.JPG", path "D:/Library/Mobile Repository/Sam Mobile/Albums/2023/04 April/iPhone 12/20230427_122359 091_1609 iPhone 12.JPG", path "D:/Library/Mobile Repository/Sam Mobile/Albums/2023/04 April/iPhone 12/20230427_122359 121_0403 iPhone 12.JPG", path "D:/Library/Mobile Repository/Sam Mobile/Albums/2023/05 May/iPhone 12/20230503_084020 091_1609 iPhone 12.JPG", path "D:/Library/Mobile Repository/Sam Mobile/Albums/2023/05 May/iPhone 12/20230503_084020 121_0403 iPhone 12.JPG", path "D:/Library/Mobile Repository/Sam Mobile/Albums/2023/05 May/iPhone 12/20230503_084119 091_1609 iPhone 12.JPG", path "D:/Library/Mobile Repository/Sam Mobile/Albums/2023/05 May/iPhone 12/20230503_084119 121_0403 iPhone 12.JPG", path "D:/Library/Mobile Repository/Sam Mobile/Albums/2023/05 May/iPhone 12/20230503_084152 091_1609 iPhone 12.JPG", path "D:/Library/Mobile Repository/Sam Mobile/Albums/2023/05 May/iPhone 12/20230503_084152 121_0403 iPhone 12.JPG", path "D:/Library/Mobile Repository/Sam Mobile/Albums/2023/05 May/iPhone 12/20230503_084207 091_1609 iPhone 12.JPG", path "D:/Library/Mobile Repository/Sam Mobile/Albums/2023/05 May/iPhone 12/20230503_084207 121_0403 iPhone 12.JPG", path "D:/Library/Mobile Repository/Sam Mobile/Albums/2023/05 May/iPhone 12/20230503_092656 091_1609 iPhone 12.JPG", path "D:/Library/Mobile Repository/Sam Mobile/Albums/2023/05 May/iPhone 12/20230503_092656 121_0403 iPhone 12.JPG", path "D:/Library/Mobile Repository/Sam Mobile/Albums/2023/05 May/iPhone 12/20230503_092834 091_1609 iPhone 12.JPG", path "D:/Library/Mobile Repository/Sam Mobile/Albums/2023/05 May/iPhone 12/20230503_092834 121_0403 iPhone 12.JPG", path "D:/Library/Mobile Repository/Sam Mobile/Albums/2023/05 May/iPhone 12/20230503_093411 091_1609 iPhone 12.JPG", path "D:/Library/Mobile Repository/Sam Mobile/Albums/2023/05 May/iPhone 12/20230503_093411 121_0403 iPhone 12.JPG", path "D:/Library/Mobile Repository/Sam Mobile/Albums/2023/05 May/iPhone 12/20230503_093534 091_0000 iPhone 12.JPG", path "D:/Library/Mobile Repository/Sam Mobile/Albums/2023/05 May/iPhone 12/20230503_093534 121_0403 iPhone 12.JPG", path "D:/Library/Mobile Repository/Sam Mobile/Albums/2023/05 May/iPhone 12/20230503_093619 091_1609 iPhone 12.JPG", path "D:/Library/Mobile Repository/Sam Mobile/Albums/2023/05 May/iPhone 12/20230503_093619 121_0403 iPhone 12.JPG", path "D:/Library/Mobile Repository/Sam Mobile/Albums/2023/05 May/iPhone 12/20230503_093636 091_1609 iPhone 12.JPG", path "D:/Library/Mobile Repository/Sam Mobile/Albums/2023/05 May/iPhone 12/20230503_093636 121_0403 iPhone 12.JPG", path "D:/Library/Mobile Repository/Sam Mobile/Albums/2023/05 May/iPhone 12/20230503_093956 091_1609 iPhone 12.JPG", path "D:/Library/Mobile Repository/Sam Mobile/Albums/2023/05 May/iPhone 12/20230503_093956 121_0403 iPhone 12.JPG", path "D:/Library/Mobile Repository/Sam Mobile/Albums/2023/05 May/iPhone 12/20230503_124525 091_1609 iPhone 12.JPG", path "D:/Library/Mobile Repository/Sam Mobile/Albums/2023/05 May/iPhone 12/20230503_124525 121_0403 iPhone 12.JPG", path "D:/Library/Mobile Repository/Sam Mobile/Albums/2023/05 May/iPhone 12/20230503_125240 091_1609 iPhone 12.JPG", path "D:/Library/Mobile Repository/Sam Mobile/Albums/2023/05 May/iPhone 12/20230503_125240 121_0403 iPhone 12.JPG", path "D:/Library/Mobile Repository/Sam Mobile/Albums/2023/05 May/iPhone 12/20230503_133902 091_1609 iPhone 12.JPG", path "D:/Library/Mobile Repository/Sam Mobile/Albums/2023/05 May/iPhone 12/20230503_133902 121_0403 iPhone 12.JPG", path "D:/Library/Mobile Repository/Sam Mobile/Albums/2023/05 May/iPhone 12/20230503_170229 091_1609 iPhone 12.JPG", path "D:/Library/Mobile Repository/Sam Mobile/Albums/2023/05 May/iPhone 12/20230503_170229 121_0403 iPhone 12.JPG", path "D:/Library/Mobile Repository/Sam Mobile/Albums/2023/05 May/iPhone 12/20230503_170241 091_1609 iPhone 12.JPG", path "D:/Library/Mobile Repository/Sam Mobile/Albums/2023/05 May/iPhone 12/20230503_170241 121_0403 iPhone 12.JPG", path "D:/Library/Mobile Repository/Sam Mobile/Albums/2023/05 May/iPhone 12/20230503_170244 091_1609 iPhone 12.JPG", path "D:/Library/Mobile Repository/Sam Mobile/Albums/2023/05 May/iPhone 12/20230503_170244 121_0403 iPhone 12.JPG", path "D:/Library/Mobile Repository/Sam Mobile/Albums/2023/05 May/iPhone 12/20230504_090314 091_1609 iPhone 12.JPG", path "D:/Library/Mobile Repository/Sam Mobile/Albums/2023/05 May/iPhone 12/20230504_090314 121_0403 iPhone 12.JPG", path "D:/Library/Mobile Repository/Sam Mobile/Albums/2023/05 May/iPhone 12/20230504_090318 091_1609 iPhone 12.JPG", path "D:/Library/Mobile Repository/Sam Mobile/Albums/2023/05 May/iPhone 12/20230504_090318 121_0403 iPhone 12.JPG", path "D:/Library/Mobile Repository/Sam Mobile/Albums/2023/05 May/iPhone 12/20230504_090331 091_1609 iPhone 12.JPG", path "D:/Library/Mobile Repository/Sam Mobile/Albums/2023/05 May/iPhone 12/20230504_090331 121_0403 iPhone 12.JPG", path "D:/Library/Mobile Repository/Sam Mobile/Albums/2023/05 May/iPhone 12/20230504_090807 091_1609 iPhone 12.JPG", path "D:/Library/Mobile Repository/Sam Mobile/Albums/2023/05 May/iPhone 12/20230504_090807 121_0403 iPhone 12.JPG", path "D:/Library/Mobile Repository/Sam Mobile/Albums/2023/05 May/iPhone 12/20230504_090810 091_1609 iPhone 12.JPG", path "D:/Library/Mobile Repository/Sam Mobile/Albums/2023/05 May/iPhone 12/20230504_090810 121_0403 iPhone 12.JPG", path "D:/Library/Mobile Repository/Sam Mobile/Albums/2023/05 May/iPhone 12/20230504_090833 091_1609 iPhone 12.JPG", path "D:/Library/Mobile Repository/Sam Mobile/Albums/2023/05 May/iPhone 12/20230504_090833 121_0403 iPhone 12.JPG", path "D:/Library/Mobile Repository/Sam Mobile/Albums/2023/05 May/iPhone 12/20230504_094026 091_1609 iPhone 12.JPG", path "D:/Library/Mobile Repository/Sam Mobile/Albums/2023/05 May/iPhone 12/20230504_094026 121_0403 iPhone 12.JPG", path "D:/Library/Mobile Repository/Sam Mobile/Albums/2023/05 May/iPhone 12/20230504_094041 091_1609 iPhone 12.JPG", path "D:/Library/Mobile Repository/Sam Mobile/Albums/2023/05 May/iPhone 12/20230504_094041 121_0403 iPhone 12.JPG", path "D:/Library/Mobile Repository/Sam Mobile/Albums/2023/05 May/iPhone 12/20230504_094206 091_1609 iPhone 12.JPG", path "D:/Library/Mobile Repository/Sam Mobile/Albums/2023/05 May/iPhone 12/20230504_094206 121_0403 iPhone 12.JPG", path "D:/Library/Mobile Repository/Sam Mobile/Albums/2023/05 May/iPhone 12/20230504_094247 091_1609 iPhone 12.JPG", path "D:/Library/Mobile Repository/Sam Mobile/Albums/2023/05 May/iPhone 12/20230504_094247 121_0403 iPhone 12.JPG", path "D:/Library/Mobile Repository/Sam Mobile/Albums/2023/05 May/iPhone 12/20230504_095050 091_1609 iPhone 12.JPG", path "D:/Library/Mobile Repository/Sam Mobile/Albums/2023/05 May/iPhone 12/20230504_095050 121_0403 iPhone 12.JPG", path "D:/Library/Mobile Repository/Sam Mobile/Albums/2023/05 May/iPhone 12/20230504_103425 091_1609 iPhone 12.JPG", path "D:/Library/Mobile Repository/Sam Mobile/Albums/2023/05 May/iPhone 12/20230504_103425 121_0403 iPhone 12.JPG", path "D:/Library/Mobile Repository/Sam Mobile/Albums/2023/05 May/iPhone 12/20230504_103438 091_1609 iPhone 12.JPG", path "D:/Library/Mobile Repository/Sam Mobile/Albums/2023/05 May/iPhone 12/20230504_103438 121_0403 iPhone 12.JPG", path "D:/Library/Mobile Repository/Sam Mobile/Albums/2023/05 May/iPhone 12/20230504_103440 091_1609 iPhone 12.JPG", path "D:/Library/Mobile Repository/Sam Mobile/Albums/2023/05 May/iPhone 12/20230504_103440 121_0403 iPhone 12.JPG", path "D:/Library/Mobile Repository/Sam Mobile/Albums/2023/05 May/iPhone 12/20230504_103441 091_1609 iPhone 12.JPG", path "D:/Library/Mobile Repository/Sam Mobile/Albums/2023/05 May/iPhone 12/20230504_103441 121_0403 iPhone 12.JPG", path "D:/Library/Mobile Repository/Sam Mobile/Albums/2023/05 May/iPhone 12/20230504_123729 091_0000 iPhone 12.JPG", path "D:/Library/Mobile Repository/Sam Mobile/Albums/2023/05 May/iPhone 12/20230504_123729 121_0403 iPhone 12.JPG", path "D:/Library/Mobile Repository/Sam Mobile/Albums/2023/05 May/iPhone 12/20230504_124150 091_1609 iPhone 12.JPG", path "D:/Library/Mobile Repository/Sam Mobile/Albums/2023/05 May/iPhone 12/20230504_124150 121_0403 iPhone 12.JPG", path "D:/Library/Mobile Repository/Sam Mobile/Albums/2023/05 May/iPhone 12/20230504_124155 091_1609 iPhone 12.JPG", path "D:/Library/Mobile Repository/Sam Mobile/Albums/2023/05 May/iPhone 12/20230504_124155 121_0403 iPhone 12.JPG", path "D:/Library/Mobile Repository/Sam Mobile/Albums/2023/05 May/iPhone 12/20230504_161414 091_1609 iPhone 12.JPG", path "D:/Library/Mobile Repository/Sam Mobile/Albums/2023/05 May/iPhone 12/20230504_161414 121_0403 iPhone 12.JPG", path "D:/Library/Mobile Repository/Sam Mobile/Albums/2023/05 May/iPhone 12/20230504_161424 091_1609 iPhone 12.JPG", path "D:/Library/Mobile Repository/Sam Mobile/Albums/2023/05 May/iPhone 12/20230504_161424 121_0403 iPhone 12.JPG", path "D:/Library/Mobile Repository/Sam Mobile/Albums/2023/05 May/iPhone 12/20230504_162814 091_1609 iPhone 12.JPG", path "D:/Library/Mobile Repository/Sam Mobile/Albums/2023/05 May/iPhone 12/20230504_162814 121_0403 iPhone 12.JPG", path "D:/Library/Mobile Repository/Sam Mobile/Albums/2023/05 May/iPhone 12/20230504_162917 091_1609 iPhone 12.JPG", path "D:/Library/Mobile Repository/Sam Mobile/Albums/2023/05 May/iPhone 12/20230504_162917 121_0403 iPhone 12.JPG", path "D:/Library/Mobile Repository/Sam Mobile/Albums/2023/05 May/iPhone 12/20230504_162941 091_1609 iPhone 12.JPG", path "D:/Library/Mobile Repository/Sam Mobile/Albums/2023/05 May/iPhone 12/20230504_162941 121_0403 iPhone 12.JPG", path "D:/Library/Mobile Repository/Sam Mobile/Albums/2023/05 May/iPhone 12/20230504_162956 091_1609 iPhone 12.JPG", path "D:/Library/Mobile Repository/Sam Mobile/Albums/2023/05 May/iPhone 12/20230504_162956 121_0403 iPhone 12.JPG", path "D:/Library/Mobile Repository/Sam Mobile/Albums/2023/05 May/iPhone 12/20230504_162959 091_1609 iPhone 12.JPG", path "D:/Library/Mobile Repository/Sam Mobile/Albums/2023/05 May/iPhone 12/20230504_162959 121_0403 iPhone 12.JPG", path "D:/Library/Mobile Repository/Sam Mobile/Albums/2023/05 May/iPhone 12/20230504_163021 091_1609 iPhone 12.JPG", path "D:/Library/Mobile Repository/Sam Mobile/Albums/2023/05 May/iPhone 12/20230504_163021 121_0403 iPhone 12.JPG", path "D:/Library/Mobile Repository/Sam Mobile/Albums/2023/05 May/iPhone 12/20230504_163128 091_1609 iPhone 12.JPG", path "D:/Library/Mobile Repository/Sam Mobile/Albums/2023/05 May/iPhone 12/20230504_163128 121_0403 iPhone 12.JPG", path "D:/Library/Mobile Repository/Sam Mobile/Albums/2023/05 May/iPhone 12/20230504_163155 091_1609 iPhone 12.JPG", path "D:/Library/Mobile Repository/Sam Mobile/Albums/2023/05 May/iPhone 12/20230504_163155 121_0403 iPhone 12.JPG", path "D:/Library/Mobile Repository/Sam Mobile/Albums/2023/05 May/iPhone 12/20230504_163211 091_1609 iPhone 12.JPG", path "D:/Library/Mobile Repository/Sam Mobile/Albums/2023/05 May/iPhone 12/20230504_163211 121_0403 iPhone 12.JPG", path "D:/Library/Mobile Repository/Sam Mobile/Albums/2023/05 May/iPhone 12/20230504_163232 091_1609 iPhone 12.JPG", path "D:/Library/Mobile Repository/Sam Mobile/Albums/2023/05 May/iPhone 12/20230504_163232 121_0403 iPhone 12.JPG", path "D:/Library/Mobile Repository/Sam Mobile/Albums/2023/05 May/iPhone 12/20230504_163235 091_1609 iPhone 12.JPG", path "D:/Library/Mobile Repository/Sam Mobile/Albums/2023/05 May/iPhone 12/20230504_163235 121_0403 iPhone 12.JPG", path "D:/Library/Mobile Repository/Sam Mobile/Albums/2023/05 May/iPhone 12/20230504_163309 091_1609 iPhone 12.JPG", path "D:/Library/Mobile Repository/Sam Mobile/Albums/2023/05 May/iPhone 12/20230504_163309 121_0403 iPhone 12.JPG", path "D:/Library/Mobile Repository/Sam Mobile/Albums/2023/05 May/iPhone 12/20230504_163310 091_1609 iPhone 12.JPG", path "D:/Library/Mobile Repository/Sam Mobile/Albums/2023/05 May/iPhone 12/20230504_163310 121_0403 iPhone 12.JPG", path "D:/Library/Mobile Repository/Sam Mobile/Albums/2023/05 May/iPhone 12/20230504_164247 091_1609 iPhone 12.JPG", path "D:/Library/Mobile Repository/Sam Mobile/Albums/2023/05 May/iPhone 12/20230504_164247 121_0403 iPhone 12.JPG", path "D:/Library/Mobile Repository/Sam Mobile/Albums/2023/05 May/iPhone 12/20230504_164249 091_1609 iPhone 12.JPG", path "D:/Library/Mobile Repository/Sam Mobile/Albums/2023/05 May/iPhone 12/20230504_164249 121_0403 iPhone 12.JPG", path "D:/Library/Mobile Repository/Sam Mobile/Albums/2023/05 May/iPhone 12/20230504_180902 091_1609 iPhone 12.JPG", path "D:/Library/Mobile Repository/Sam Mobile/Albums/2023/05 May/iPhone 12/20230504_180902 121_0403 iPhone 12.JPG", path "D:/Library/Mobile Repository/Sam Mobile/Albums/2023/05 May/iPhone 12/20230504_180906 091_1609 iPhone 12.JPG", path "D:/Library/Mobile Repository/Sam Mobile/Albums/2023/05 May/iPhone 12/20230504_180906 121_0403 iPhone 12.JPG", path "D:/Library/Mobile Repository/Sam Mobile/Albums/2023/05 May/iPhone 12/20230504_181131 091_1609 iPhone 12.JPG", path "D:/Library/Mobile Repository/Sam Mobile/Albums/2023/05 May/iPhone 12/20230504_181131 121_0403 iPhone 12.JPG", path "D:/Library/Mobile Repository/Sam Mobile/Albums/2023/05 May/iPhone 12/20230504_181217 091_1609 iPhone 12.JPG", path "D:/Library/Mobile Repository/Sam Mobile/Albums/2023/05 May/iPhone 12/20230504_181217 121_0403 iPhone 12.JPG", path "D:/Library/Mobile Repository/Sam Mobile/Albums/2023/05 May/iPhone 12/20230504_195213 091_1609 iPhone 12.JPG", path "D:/Library/Mobile Repository/Sam Mobile/Albums/2023/05 May/iPhone 12/20230504_195213 121_0403 iPhone 12.JPG", path "D:/Library/Mobile Repository/Sam Mobile/Albums/2023/05 May/iPhone 12/20230504_195227 091_1609 iPhone 12.JPG", path "D:/Library/Mobile Repository/Sam Mobile/Albums/2023/05 May/iPhone 12/20230504_195227 121_0403 iPhone 12.JPG", path "D:/Library/Mobile Repository/Sam Mobile/Albums/2023/05 May/iPhone 12/20230505_104811 091_1609 iPhone 12.JPG", path "D:/Library/Mobile Repository/Sam Mobile/Albums/2023/05 May/iPhone 12/20230505_104811 121_0403 iPhone 12.JPG", path "D:/Library/Mobile Repository/Sam Mobile/Albums/2023/05 May/iPhone 12/20230505_104821 091_1609 iPhone 12.JPG", path "D:/Library/Mobile Repository/Sam Mobile/Albums/2023/05 May/iPhone 12/20230505_104821 121_0403 iPhone 12.JPG", path "D:/Library/Mobile Repository/Sam Mobile/Albums/2023/05 May/iPhone 12/20230505_104828 091_1609 iPhone 12.JPG", path "D:/Library/Mobile Repository/Sam Mobile/Albums/2023/05 May/iPhone 12/20230505_104828 121_0403 iPhone 12.JPG", path "D:/Library/Mobile Repository/Sam Mobile/Albums/2023/05 May/iPhone 12/20230505_104914 091_1609 iPhone 12.JPG", path "D:/Library/Mobile Repository/Sam Mobile/Albums/2023/05 May/iPhone 12/20230505_104914 121_0403 iPhone 12.JPG", path "D:/Library/Mobile Repository/Sam Mobile/Albums/2023/05 May/iPhone 12/20230505_104920 091_1609 iPhone 12.JPG", path "D:/Library/Mobile Repository/Sam Mobile/Albums/2023/05 May/iPhone 12/20230505_104920 121_0403 iPhone 12.JPG", path "D:/Library/Mobile Repository/Sam Mobile/Albums/2023/05 May/iPhone 12/20230505_122657 091_1609 iPhone 12.JPG", path "D:/Library/Mobile Repository/Sam Mobile/Albums/2023/05 May/iPhone 12/20230505_122657 121_0403 iPhone 12.JPG", path "D:/Library/Mobile Repository/Sam Mobile/Albums/2023/05 May/iPhone 12/20230505_122659 091_1609 iPhone 12.JPG", path "D:/Library/Mobile Repository/Sam Mobile/Albums/2023/05 May/iPhone 12/20230505_122659 121_0403 iPhone 12.JPG", path "D:/Library/Mobile Repository/Sam Mobile/Albums/2023/05 May/iPhone 12/20230505_135227 091_1609 iPhone 12.JPG", path "D:/Library/Mobile Repository/Sam Mobile/Albums/2023/05 May/iPhone 12/20230505_135227 121_0403 iPhone 12.JPG", path "D:/Library/Mobile Repository/Sam Mobile/Albums/2023/05 May/iPhone 12/20230511_121309 091_1609 iPhone 12.JPG", path "D:/Library/Mobile Repository/Sam Mobile/Albums/2023/05 May/iPhone 12/20230511_121309 121_0403 iPhone 12.JPG", path "D:/Library/Mobile Repository/Sam Mobile/Albums/2023/05 May/iPhone 12/20230511_124139 091_1609 iPhone 12.JPG", path "D:/Library/Mobile Repository/Sam Mobile/Albums/2023/05 May/iPhone 12/20230511_124139 121_0403 iPhone 12.JPG", path "D:/Library/Mobile Repository/Sam Mobile/Albums/2023/05 May/iPhone 12/20230511_124143 091_1609 iPhone 12.JPG", path "D:/Library/Mobile Repository/Sam Mobile/Albums/2023/05 May/iPhone 12/20230511_124143 121_0403 iPhone 12.JPG", path "D:/Library/Mobile Repository/Sam Mobile/Albums/2023/05 May/iPhone 12/20230511_124214 091_1609 iPhone 12.JPG", path "D:/Library/Mobile Repository/Sam Mobile/Albums/2023/05 May/iPhone 12/20230511_124214 121_0403 iPhone 12.JPG", path "D:/Library/Mobile Repository/Sam Mobile/Albums/2023/05 May/iPhone 12/20230511_125854 091_1609 iPhone 12.JPG", path "D:/Library/Mobile Repository/Sam Mobile/Albums/2023/05 May/iPhone 12/20230511_125854 121_0403 iPhone 12.JPG", path "D:/Library/Mobile Repository/Sam Mobile/Albums/2023/05 May/iPhone 12/20230525_145546 092_0000 iPhone 12.JPG", path "D:/Library/Mobile Repository/Sam Mobile/Albums/2023/05 May/iPhone 12/20230525_145546 121_0403 iPhone 12.JPG", path "D:/Library/Mobile Repository/Sam Mobile/Albums/2023/06 June/iPhone 12/20230606_203158 104_0000 iPhone 12.JPG", path "D:/Library/Mobile Repository/Sam Mobile/Albums/2023/06 June/iPhone 12/20230606_203158 121_0403 iPhone 12.JPG", path "D:/Library/Mobile Repository/Sam Mobile/Albums/2023/07 July/iPhone 12/20230711_115024 052_0000 iPhone 12.JPG", path "D:/Library/Mobile Repository/Sam Mobile/Albums/2023/07 July/iPhone 12/20230711_115024 121_0403 iPhone 12.JPG", path "D:/Library/Mobile Repository/Sam Mobile/Albums/2023/07 July/iPhone 12/20230711_125511 043_0000 iPhone 12.JPG", path "D:/Library/Mobile Repository/Sam Mobile/Albums/2023/07 July/iPhone 12/20230711_125511 121_0403 iPhone 12.JPG", path "D:/Library/Mobile Repository/Sam Mobile/Albums/2023/08 August/iPhone 12/20230801_215345 078_0000 iPhone 12.JPG", path "D:/Library/Mobile Repository/Sam Mobile/Albums/2023/08 August/iPhone 12/20230801_215345 121_0403 iPhone 12.JPG", path "D:/Library/Mobile Repository/Sam Mobile/Albums/2023/08 August/iPhone 12/20230806_135718 026_0000 iPhone 12.JPG", path "D:/Library/Mobile Repository/Sam Mobile/Albums/2023/08 August/iPhone 12/20230806_135718 121_0403 iPhone 12.JPG", path "D:/Library/Mobile Repository/Sam Mobile/Albums/2023/08 August/iPhone 12/20230806_173709 083_0000 iPhone 12.JPG", path "D:/Library/Mobile Repository/Sam Mobile/Albums/2023/08 August/iPhone 12/20230806_173709 121_0403 iPhone 12.JPG", path "D:/Library/Mobile Repository/Sam Mobile/Albums/2023/08 August/iPhone 12/20230806_173728 072_0000 iPhone 12.JPG", path "D:/Library/Mobile Repository/Sam Mobile/Albums/2023/08 August/iPhone 12/20230806_173728 121_0403 iPhone 12.JPG", path "D:/Library/Mobile Repository/Sam Mobile/Albums/2023/08 August/iPhone 12/20230815_204638 047_0000 iPhone 12.JPG", path "D:/Library/Mobile Repository/Sam Mobile/Albums/2023/08 August/iPhone 12/20230815_204638 121_0403 iPhone 12.JPG", path "D:/Library/Mobile Repository/Sam Mobile/Albums/2023/08 August/iPhone 12/20230819_100907 121_0403 iPhone 12.JPG", path "D:/Library/Mobile Repository/Sam Mobile/Albums/2023/08 August/iPhone 12/20230819_100907 124_0000 iPhone 12.JPG", path "D:/Library/Mobile Repository/Sam Mobile/Albums/2023/08 August/iPhone 12/20230826_183432 030_0000 iPhone 12.JPG", path "D:/Library/Mobile Repository/Sam Mobile/Albums/2023/08 August/iPhone 12/20230826_183432 121_0403 iPhone 12.JPG", path "D:/Library/Mobile Repository/Sam Mobile/Albums/2023/09 September/iPhone 12/20230925_062907 039_0000 iPhone 12.JPG", path "D:/Library/Mobile Repository/Sam Mobile/Albums/2023/09 September/iPhone 12/20230925_062907 071_0403 iPhone 12.JPG", path "D:/Library/Mobile Repository/Sam Mobile/Albums/2023/10 October/iPhone 12/20231008_192302 047_0000 iPhone 12.JPG", path "D:/Library/Mobile Repository/Sam Mobile/Albums/2023/10 October/iPhone 12/20231008_192302 121_0403 iPhone 12.JPG", path "D:/Library/Mobile Repository/Sam Mobile/Albums/2023/10 October/iPhone 12/20231010_081620 022_0000 iPhone 12.JPG", path "D:/Library/Mobile Repository/Sam Mobile/Albums/2023/10 October/iPhone 12/20231010_081620 121_0403 iPhone 12.JPG", path "D:/Library/Mobile Repository/Sam Mobile/Albums/2023/10 October/iPhone 12/20231021_124250 071_0304 iPhone 12.JPG", path "D:/Library/Mobile Repository/Sam Mobile/Albums/2023/10 October/iPhone 12/20231021_124250 071_0403 iPhone 12.JPG", path "D:/Library/Mobile Repository/Sam Mobile/Albums/2023/10 October/iPhone 12/20231021_124339 071_0304 iPhone 12.JPG", path "D:/Library/Mobile Repository/Sam Mobile/Albums/2023/10 October/iPhone 12/20231021_124339 071_0403 iPhone 12.JPG", path "D:/Library/Mobile Repository/Sam Mobile/Albums/2023/10 October/iPhone 12/20231021_124451 071_0304 iPhone 12.JPG", path "D:/Library/Mobile Repository/Sam Mobile/Albums/2023/10 October/iPhone 12/20231021_124451 071_0403 iPhone 12.JPG", path "D:/Library/Mobile Repository/Sam Mobile/Albums/2023/11 November/iPhone 12/20231102_082813 068_0000 iPhone 12.JPG", path "D:/Library/Mobile Repository/Sam Mobile/Albums/2023/11 November/iPhone 12/20231102_082813 121_0403 iPhone 12.JPG", path "D:/Library/Mobile Repository/Sam Mobile/Albums/2023/11 November/iPhone 12/20231125_192250 051_0000 iPhone 12.JPG", path "D:/Library/Mobile Repository/Sam Mobile/Albums/2023/11 November/iPhone 12/20231125_192250 121_0403 iPhone 12.JPG", path "D:/Library/Mobile Repository/Sam Mobile/Albums/2023/12 December/iPhone 12/20231208_152715 008_0101 iPhone 12.JPG", path "D:/Library/Mobile Repository/Sam Mobile/Albums/2023/12 December/iPhone 12/20231208_152715 121_0403 iPhone 12.JPG", path "D:/Library/Mobile Repository/Sam Mobile/Albums/2023/12 December/iPhone 12/20231212_110640 008_0000 iPhone 12.JPG", path "D:/Library/Mobile Repository/Sam Mobile/Albums/2023/12 December/iPhone 12/20231212_110640 121_0403 iPhone 12.JPG", path "D:/Library/Mobile Repository/Sam Mobile/Albums/2023/12 December/iPhone 12/20231218_204009 032_0000 iPhone 12.JPG", path "D:/Library/Mobile Repository/Sam Mobile/Albums/2023/12 December/iPhone 12/20231218_204009 121_0403 iPhone 12.JPG", path "D:/Library/Mobile Repository/Sam Mobile/Albums/2023/12 December/iPhone 12/20231220_192656 121_0304 iPhone 12.JPG", path "D:/Library/Mobile Repository/Sam Mobile/Albums/2023/12 December/iPhone 12/20231220_192656 121_0403 iPhone 12.JPG", path "D:/Library/Mobile Repository/Sam Mobile/Albums/2024/01 January/iPhone 12/20240101_162728 121_0304 iPhone 12.JPG", path "D:/Library/Mobile Repository/Sam Mobile/Albums/2024/01 January/iPhone 12/20240101_162728 121_0403 iPhone 12.JPG", path "D:/Library/Mobile Repository/Sam Mobile/Albums/2024/01 January/iPhone 12/20240101_162742 121_0304 iPhone 12.JPG", path "D:/Library/Mobile Repository/Sam Mobile/Albums/2024/01 January/iPhone 12/20240101_162742 121_0403 iPhone 12.JPG", path "D:/Library/Mobile Repository/Sam Mobile/Albums/2024/01 January/iPhone 12/20240105_202442 030_0000 iPhone 12.JPG", path "D:/Library/Mobile Repository/Sam Mobile/Albums/2024/01 January/iPhone 12/20240105_202442 121_0403 iPhone 12.JPG", path "D:/Library/Mobile Repository/Sam Mobile/Albums/2024/01 January/iPhone 12/20240111_120339 023_0000 iPhone 12.JPG", path "D:/Library/Mobile Repository/Sam Mobile/Albums/2024/01 January/iPhone 12/20240111_120339 121_0403 iPhone 12.JPG", path "D:/Library/Mobile Repository/Sam Mobile/Albums/2024/01 January/iPhone 12/20240114_185850 043_0000 iPhone 12.JPG", path "D:/Library/Mobile Repository/Sam Mobile/Albums/2024/01 January/iPhone 12/20240114_185850 121_0403 iPhone 12.JPG", path "D:/Library/Mobile Repository/Sam Mobile/Albums/2024/01 January/iPhone 12/20240114_190117 006_0000 iPhone 12.JPG", path "D:/Library/Mobile Repository/Sam Mobile/Albums/2024/01 January/iPhone 12/20240114_190117 121_0403 iPhone 12.JPG", path "D:/Library/Mobile Repository/Sam Mobile/Albums/2024/01 January/iPhone 12/20240117_153026 061_0000 iPhone 12.JPG", path "D:/Library/Mobile Repository/Sam Mobile/Albums/2024/01 January/iPhone 12/20240117_153026 121_0403 iPhone 12.JPG", path "D:/Library/Mobile Repository/Sam Mobile/Albums/2024/01 January/iPhone 12/20240121_125434 025_0000 iPhone 12.JPG", path "D:/Library/Mobile Repository/Sam Mobile/Albums/2024/01 January/iPhone 12/20240121_125434 121_0403 iPhone 12.JPG", path "D:/Library/Mobile Repository/Sam Mobile/Albums/2024/01 January/iPhone 12/20240121_130225 021_0000 iPhone 12.JPG", path "D:/Library/Mobile Repository/Sam Mobile/Albums/2024/01 January/iPhone 12/20240121_130225 121_0403 iPhone 12.JPG", path "D:/Library/Mobile Repository/Sam Mobile/Albums/2024/02 February/iPhone 12/20240211_150840 038_0000 iPhone 12.JPG", path "D:/Library/Mobile Repository/Sam Mobile/Albums/2024/02 February/iPhone 12/20240211_150840 121_0403 iPhone 12.JPG", path "D:/Library/Mobile Repository/Sam Mobile/Albums/2024/02 February/iPhone 12/20240216_180240 052_0000 iPhone 12.JPG", path "D:/Library/Mobile Repository/Sam Mobile/Albums/2024/02 February/iPhone 12/20240216_180240 121_0403 iPhone 12.JPG", path "D:/Library/Mobile Repository/Sam Mobile/Albums/2024/02 February/iPhone 12/20240227_155333 063_0000 iPhone 12.JPG", path "D:/Library/Mobile Repository/Sam Mobile/Albums/2024/02 February/iPhone 12/20240227_155333 121_0403 iPhone 12.JPG", path "D:/Library/Mobile Repository/Sam Mobile/Albums/2024/03 March/iPhone 12/20240301_185512 067_0000 iPhone 12.JPG", path "D:/Library/Mobile Repository/Sam Mobile/Albums/2024/03 March/iPhone 12/20240301_185512 121_0403 iPhone 12.JPG", path "D:/Library/Mobile Repository/Sam Mobile/Albums/2024/03 March/iPhone 12/20240308_090026 057_0000 iPhone 12.JPG", path "D:/Library/Mobile Repository/Sam Mobile/Albums/2024/03 March/iPhone 12/20240308_090026 121_0403 iPhone 12.JPG", path "D:/Library/Mobile Repository/Sam Mobile/Albums/2024/03 March/iPhone 12/20240308_225359 068_0000 iPhone 12.JPG", path "D:/Library/Mobile Repository/Sam Mobile/Albums/2024/03 March/iPhone 12/20240308_225359 121_0403 iPhone 12.JPG", path "D:/Library/Mobile Repository/Sam Mobile/Albums/2024/03 March/iPhone 12/20240313_114742 045_0000 iPhone 12.JPG", path "D:/Library/Mobile Repository/Sam Mobile/Albums/2024/03 March/iPhone 12/20240313_114742 121_0403 iPhone 12.JPG", path "D:/Library/Mobile Repository/Sam Mobile/Albums/2024/03 March/iPhone 12/20240315_151053 121_0304 iPhone 12.JPG", path "D:/Library/Mobile Repository/Sam Mobile/Albums/2024/03 March/iPhone 12/20240315_151053 121_0403 iPhone 12.JPG", path "D:/Library/Mobile Repository/Sam Mobile/Albums/2024/04 April/iPhone 12/20240404_163859 121_0403 iPhone 12 @_01.JPG", path "D:/Library/Mobile Repository/Sam Mobile/Albums/2024/04 April/iPhone 12/20240404_163859 121_0403 iPhone 12.JPG", path "D:/Library/Mobile Repository/Sam Mobile/Albums/2024/04 April/iPhone 12/20240406_072628 101_0000 iPhone 12.JPG", path "D:/Library/Mobile Repository/Sam Mobile/Albums/2024/04 April/iPhone 12/20240406_072628 121_0403 iPhone 12.JPG", path "D:/Library/Mobile Repository/Sam Mobile/Albums/2024/04 April/iPhone 12/20240407_205242 121_0304 iPhone 12.JPG", path "D:/Library/Mobile Repository/Sam Mobile/Albums/2024/04 April/iPhone 12/20240407_205242 121_0403 iPhone 12.JPG", path "D:/Library/Mobile Repository/Sam Mobile/Albums/2024/04 April/iPhone 12/20240421_221632 071_0304 iPhone 12.JPG", path "D:/Library/Mobile Repository/Sam Mobile/Albums/2024/04 April/iPhone 12/20240421_221632 071_0403 iPhone 12.JPG", path "D:/Library/Mobile Repository/Sam Mobile/Albums/2024/04 April/iPhone 12/20240421_221705 121_0304 iPhone 12.JPG", path "D:/Library/Mobile Repository/Sam Mobile/Albums/2024/04 April/iPhone 12/20240421_221705 121_0403 iPhone 12.JPG", path "D:/Library/Mobile Repository/Sam Mobile/Albums/2024/04 April/iPhone 12/20240421_221740 071_0304 iPhone 12.JPG", path "D:/Library/Mobile Repository/Sam Mobile/Albums/2024/04 April/iPhone 12/20240421_221740 071_0403 iPhone 12.JPG", path "D:/Library/Mobile Repository/Sam Mobile/Albums/2024/04 April/iPhone 12/20240426_173607 081_0000 iPhone 12.JPG", path "D:/Library/Mobile Repository/Sam Mobile/Albums/2024/04 April/iPhone 12/20240426_173607 121_0403 iPhone 12.JPG", path "D:/Library/Mobile Repository/Sam Mobile/Albums/2024/04 April/iPhone 12/20240426_175147 084_0000 iPhone 12.JPG", path "D:/Library/Mobile Repository/Sam Mobile/Albums/2024/04 April/iPhone 12/20240426_175147 121_0403 iPhone 12.JPG", path "D:/Library/Mobile Repository/Sam Mobile/Albums/2024/05 May/iPhone 12/20240508_090440 074_0000 iPhone 12.JPG", path "D:/Library/Mobile Repository/Sam Mobile/Albums/2024/05 May/iPhone 12/20240508_090440 121_0403 iPhone 12.JPG", path "D:/Library/Mobile Repository/Sam Mobile/Albums/2024/05 May/iPhone 13/20240518_122314 121_0304 iPhone 13.JPG", path "D:/Library/Mobile Repository/Sam Mobile/Albums/2024/05 May/iPhone 13/20240518_122314 121_0403 iPhone 13.JPG", path "D:/Library/Mobile Repository/Sam Mobile/Albums/2024/05 May/iPhone 13/20240518_122400 121_0304 iPhone 13.JPG", path "D:/Library/Mobile Repository/Sam Mobile/Albums/2024/05 May/iPhone 13/20240518_122400 121_0403 iPhone 13.JPG", path "D:/Library/Mobile Repository/Sam Mobile/Albums/2024/05 May/iPhone 13/20240518_122405 121_0304 iPhone 13.JPG", path "D:/Library/Mobile Repository/Sam Mobile/Albums/2024/05 May/iPhone 13/20240518_122405 121_0403 iPhone 13.JPG", path "D:/Library/Mobile Repository/Sam Mobile/Albums/2024/05 May/iPhone 13/20240518_122811 091_1609 iPhone 13.JPG", path "D:/Library/Mobile Repository/Sam Mobile/Albums/2024/05 May/iPhone 13/20240518_122811 121_0403 iPhone 13.JPG", path "D:/Library/Mobile Repository/Sam Mobile/Albums/2024/05 May/iPhone 13/20240518_122813 091_1609 iPhone 13.JPG", path "D:/Library/Mobile Repository/Sam Mobile/Albums/2024/05 May/iPhone 13/20240518_122813 121_0403 iPhone 13.JPG", path "D:/Library/Mobile Repository/Sam Mobile/Albums/2024/05 May/iPhone 13/20240519_100839 069_1609 iPhone 13.JPG", path "D:/Library/Mobile Repository/Sam Mobile/Albums/2024/05 May/iPhone 13/20240519_100839 121_0403 iPhone 13.JPG", path "D:/Library/Mobile Repository/Sam Mobile/Albums/2024/05 May/iPhone 13/20240519_103326 069_1609 iPhone 13.JPG", path "D:/Library/Mobile Repository/Sam Mobile/Albums/2024/05 May/iPhone 13/20240519_103326 121_0403 iPhone 13.JPG", path "D:/Library/Mobile Repository/Sam Mobile/Albums/2024/05 May/iPhone 13/20240519_133522 071_0403 iPhone 13.JPG", path "D:/Library/Mobile Repository/Sam Mobile/Albums/2024/05 May/iPhone 13/20240519_133522 121_0403 iPhone 13.JPG", path "D:/Library/Mobile Repository/Sam Mobile/Albums/2024/06 June/iPhone 12/20240601_114512 121_0304 iPhone 12.JPG", path "D:/Library/Mobile Repository/Sam Mobile/Albums/2024/06 June/iPhone 12/20240601_114512 121_0403 iPhone 12.JPG", path "D:/Library/Mobile Repository/Sam Mobile/Albums/2024/06 June/iPhone 12/20240601_202042 021_0000 iPhone 12.JPG", path "D:/Library/Mobile Repository/Sam Mobile/Albums/2024/06 June/iPhone 12/20240601_202042 121_0403 iPhone 12.JPG", path "D:/Library/Mobile Repository/Sam Mobile/Albums/2024/07 July/iPhone 12/20240710_091224 072_0000 iPhone 12.JPG", path "D:/Library/Mobile Repository/Sam Mobile/Albums/2024/07 July/iPhone 12/20240710_091224 121_0403 iPhone 12.JPG", path "D:/Library/Mobile Repository/Sam Mobile/Albums/2024/07 July/iPhone 12/20240720_144830 026_0000 iPhone 12.JPG", path "D:/Library/Mobile Repository/Sam Mobile/Albums/2024/07 July/iPhone 12/20240720_144830 121_0403 iPhone 12.JPG", path "D:/Library/Mobile Repository/Sam Mobile/Albums/2024/08 August/iPhone 12/20240815_120431 049_0000 iPhone 12.JPG", path "D:/Library/Mobile Repository/Sam Mobile/Albums/2024/08 August/iPhone 12/20240815_120431 121_0403 iPhone 12.JPG", path "D:/Library/Mobile Repository/Sam Mobile/Albums/2024/08 August/iPhone 12/20240815_120445 037_0000 iPhone 12.JPG", path "D:/Library/Mobile Repository/Sam Mobile/Albums/2024/08 August/iPhone 12/20240815_120445 121_0403 iPhone 12.JPG", path "D:/Library/Mobile Repository/Sam Mobile/Albums/2024/08 August/iPhone 12/20240815_120455 041_0000 iPhone 12.JPG", path "D:/Library/Mobile Repository/Sam Mobile/Albums/2024/08 August/iPhone 12/20240815_120455 121_0403 iPhone 12.JPG", path "D:/Library/Mobile Repository/Sam Mobile/Albums/2024/09 September/iPhone 12/20240905_121403 049_0000 iPhone 12.JPG", path "D:/Library/Mobile Repository/Sam Mobile/Albums/2024/09 September/iPhone 12/20240905_121403 121_0403 iPhone 12.JPG", path "D:/Library/Mobile Repository/Sam Mobile/Albums/2024/09 September/iPhone 12/20240905_121715 028_0000 iPhone 12.JPG", path "D:/Library/Mobile Repository/Sam Mobile/Albums/2024/09 September/iPhone 12/20240905_121715 121_0403 iPhone 12.JPG", path "D:/Library/Mobile Repository/Sam Mobile/Albums/2024/09 September/iPhone 12/20240913_180323 002_6659 iPhone 12.JPG", path "D:/Library/Mobile Repository/Sam Mobile/Albums/2024/09 September/iPhone 12/20240913_180323 121_0403 iPhone 12.JPG", path "D:/Library/Mobile Repository/Sam Mobile/Albums/2024/09 September/iPhone 12/20240929_163952 080_0000 iPhone 12.JPG", path "D:/Library/Mobile Repository/Sam Mobile/Albums/2024/09 September/iPhone 12/20240929_163952 121_0403 iPhone 12.JPG", path "D:/Library/Mobile Repository/Sam Mobile/Albums/2024/09 September/iPhone 12/20240930_115327 030_0000 iPhone 12.JPG", path "D:/Library/Mobile Repository/Sam Mobile/Albums/2024/09 September/iPhone 12/20240930_115327 121_0403 iPhone 12.JPG", path "D:/Library/Mobile Repository/Sam Mobile/Albums/2024/10 October/iPhone 12/20241002_163311 063_3625 iPhone 12.JPG", path "D:/Library/Mobile Repository/Sam Mobile/Albums/2024/10 October/iPhone 12/20241002_163311 121_0403 iPhone 12.JPG", path "D:/Library/Mobile Repository/Sam Mobile/Albums/2024/10 October/iPhone 12/20241002_163316 055_0000 iPhone 12.JPG", path "D:/Library/Mobile Repository/Sam Mobile/Albums/2024/10 October/iPhone 12/20241002_163316 121_0403 iPhone 12.JPG", path "D:/Library/Mobile Repository/Sam Mobile/Albums/2024/10 October/iPhone 12/20241002_163418 073_0000 iPhone 12.JPG", path "D:/Library/Mobile Repository/Sam Mobile/Albums/2024/10 October/iPhone 12/20241002_163418 121_0403 iPhone 12.JPG", path "D:/Library/Mobile Repository/Sam Mobile/Albums/2024/10 October/iPhone 12/20241008_130027 015_0000 iPhone 12.JPG", path "D:/Library/Mobile Repository/Sam Mobile/Albums/2024/10 October/iPhone 12/20241008_130027 121_0403 iPhone 12.JPG", path "D:/Library/Mobile Repository/Sam Mobile/Albums/2024/10 October/iPhone 12/20241017_202941 091_0101 iPhone 12.JPG", path "D:/Library/Mobile Repository/Sam Mobile/Albums/2024/10 October/iPhone 12/20241017_202941 121_0403 iPhone 12.JPG", path "D:/Library/Mobile Repository/Sam Mobile/Albums/2024/10 October/iPhone 12/20241027_163100 082_0000 iPhone 12.JPG", path "D:/Library/Mobile Repository/Sam Mobile/Albums/2024/10 October/iPhone 12/20241027_163100 121_0403 iPhone 12.JPG", path "D:/Library/Mobile Repository/Sam Mobile/Albums/2024/11 November/iPhone 12/20241124_083903 048_0000 iPhone 12.JPG", path "D:/Library/Mobile Repository/Sam Mobile/Albums/2024/11 November/iPhone 12/20241124_083903 121_0403 iPhone 12.JPG", path "D:/Library/Mobile Repository/Sam Mobile/Albums/2024/11 November/iPhone 12/20241128_153530 075_0000 iPhone 12.JPG", path "D:/Library/Mobile Repository/Sam Mobile/Albums/2024/11 November/iPhone 12/20241128_153530 121_0403 iPhone 12.JPG", path "D:/Library/Mobile Repository/Sam Mobile/Albums/2024/12 December/iPhone 12/20241208_121504 060_0000 iPhone 12.JPG", path "D:/Library/Mobile Repository/Sam Mobile/Albums/2024/12 December/iPhone 12/20241208_121504 121_0403 iPhone 12.JPG", path "D:/Library/Mobile Repository/Sam Mobile/Albums/2024/12 December/iPhone 12/20241226_170945 032_0000 iPhone 12.JPG", path "D:/Library/Mobile Repository/Sam Mobile/Albums/2024/12 December/iPhone 12/20241226_170945 121_0403 iPhone 12.JPG", path "D:/Library/Mobile Repository/Sam Mobile/Albums/2024/12 December/iPhone 12/20241226_170951 038_0000 iPhone 12.JPG", path "D:/Library/Mobile Repository/Sam Mobile/Albums/2024/12 December/iPhone 12/20241226_170951 121_0403 iPhone 12.JPG", path "D:/Library/Mobile Repository/Sam Mobile/Albums/2024/12 December/iPhone 12/20241226_170958 031_0000 iPhone 12.JPG", path "D:/Library/Mobile Repository/Sam Mobile/Albums/2024/12 December/iPhone 12/20241226_170958 121_0403 iPhone 12.JPG", path "D:/Library/Mobile Repository/Sam Mobile/Albums/2024/12 December/iPhone 12/20241226_171005 030_8657 iPhone 12.JPG", path "D:/Library/Mobile Repository/Sam Mobile/Albums/2024/12 December/iPhone 12/20241226_171005 121_0403 iPhone 12.JPG"] ("Destination") -> [w7] mode=indexing
    tunnel: path "D:/Library/Mobile Repository/Sam Mobile/Duplicates" ("Destination") -> [w8]
    tunnel: [w6] -> w2 mode=indexing
    n2 = Strip Path(path=w7) -> (name=w10:string)  [unwired: 1 out]
    n3 = Build Path(base path=w8, name or relative path=w10) -> (appended path=w9:path)
    n4 = File/Directory Info(path=w7) -> (path out=w4:path, error out=w5:errorcluster)  [unwired: 1 in, 5 out]
    n5 = Move(source path=w4, error in=w5, 10:w9) -> (error out=w6:errorcluster)  [unwired: 2 in, 2 out]
  }
  "Array 2" <- w2
